vi "Engineer Ambitiously One LIne.vi"() -> ()   [LabVIEW 2025]
uses:
  <vilib>/Analysis/2dsp.llb/Complex FFT.vi
  <vilib>/Analysis/1siggen.llb/Ramp Pattern by Samples.vi
  <vilib>/Analysis/2dsp.llb/Resample (constant to constant, complex single-channel).vi
  <vilib>/Analysis/NI_AALPro.lvlib
  <vilib>/Analysis/NI_AALBase.lvlib
panel:
  out "Centerpoint Offset":cdb=-0.010717500369908635-0.08034946253234411i
  in  "Individual Plots Per Vector":bool
  in  "milliseconds to wait":u32=5
  out "XY Graph":cluster{"XY Graph - Light":cdb[]}[](graph)
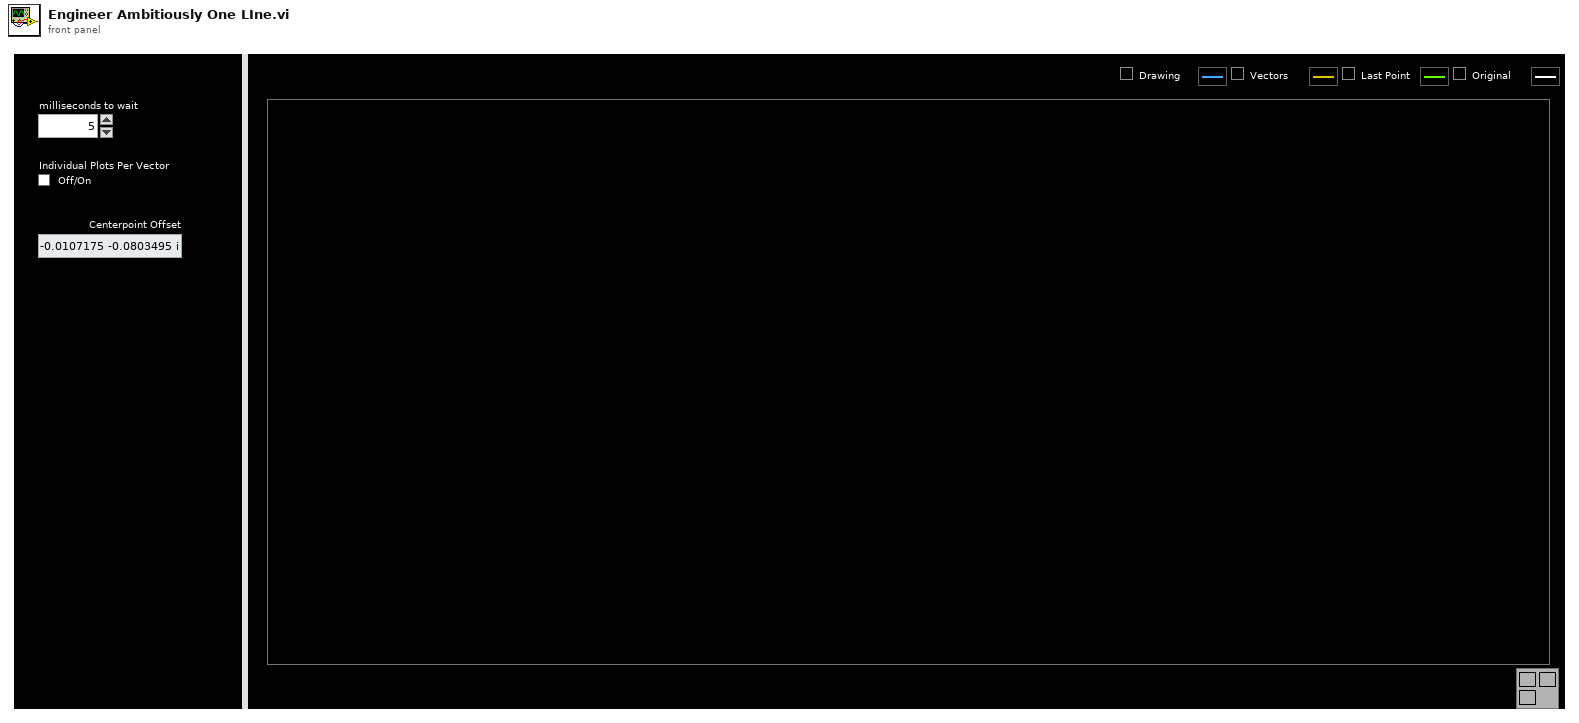
[diagram p1: front panel]
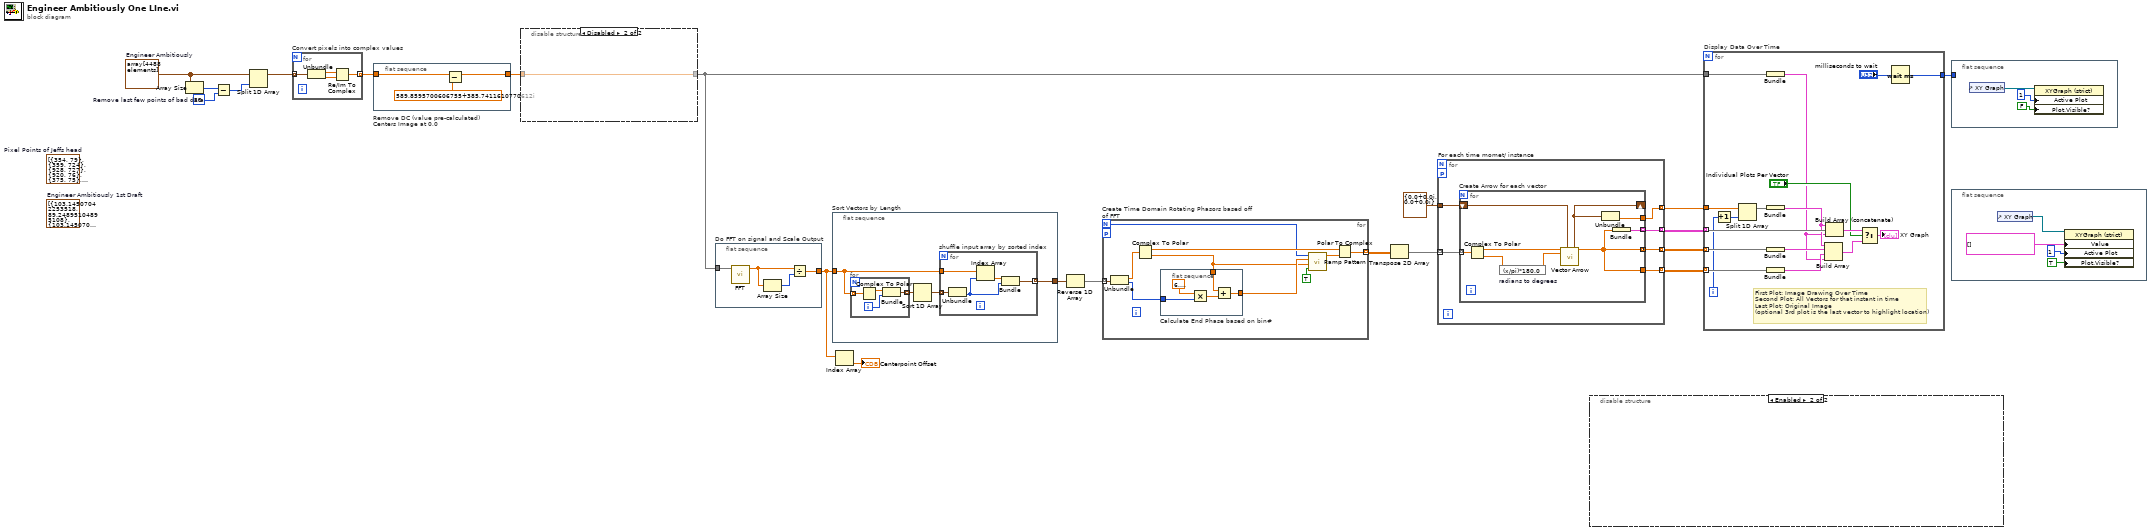
[diagram p0: block diagram]
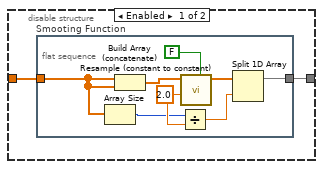
[diagram p2: hidden frame]
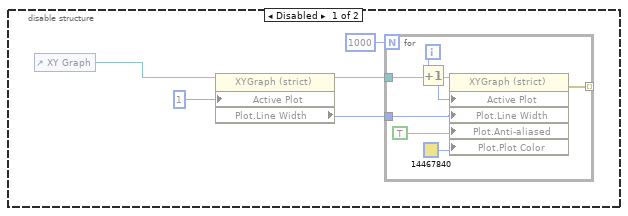
[diagram p3: hidden frame]
diagram:
  w9 = 20  # Remove last few points of bad data
  (unwired) cluster{"X":dbl, "Y":dbl}[] [{"X"=103.14507042253518, "Y"=89.24895104895108}, {"X"=103.14507042253518, "Y"=93.26013986013993}, {"X"=103.14507042253518, "Y"=95.2657342657343}, {"X"=102.14366197183094, "Y"=96.26853146853148}, {"X"=102.14366197183094, "Y"=97.27132867132866}, {"X"=102.14366197183094, "Y"=98.27412587412596}, {"X"=102.14366197183094, "Y"=99.27692307692314}, {"X"=102.14366197183094, "Y"=100.27972027972032}, {"X"=102.14366197183094, "Y"=101.2825174825175}, {"X"=102.14366197183094, "Y"=102.28531468531469}, {"X"=102.14366197183094, "Y"=103.28811188811187}, {"X"=102.14366197183094, "Y"=104.29090909090917}, {"X"=102.14366197183094, "Y"=105.29370629370635}, {"X"=102.14366197183094, "Y"=106.29650349650353}, {"X"=102.14366197183094, "Y"=107.29930069930072}, {"X"=101.14225352112672, "Y"=108.3020979020979}, {"X"=101.14225352112672, "Y"=109.30489510489508}, {"X"=101.14225352112672, "Y"=110.30769230769238}, {"X"=101.14225352112672, "Y"=111.31048951048956}, {"X"=101.14225352112672, "Y"=112.31328671328674}, {"X"=101.14225352112672, "Y"=113.31608391608393}, {"X"=101.14225352112672, "Y"=114.31888111888111}, {"X"=101.14225352112672, "Y"=115.3216783216784}, {"X"=101.14225352112672, "Y"=116.32447552447559}, {"X"=100.1408450704225, "Y"=118.33006993006995}, {"X"=100.1408450704225, "Y"=121.33846153846162}, {"X"=100.1408450704225, "Y"=123.34405594405598}, {"X"=100.1408450704225, "Y"=124.34685314685316}, {"X"=99.13943661971828, "Y"=125.34965034965035}, {"X"=98.13802816901406, "Y"=127.35524475524483}, {"X"=97.13661971830982, "Y"=130.36363636363637}, {"X"=96.1352112676056, "Y"=133.37202797202804}, {"X"=95.13380281690138, "Y"=135.3776223776224}, {"X"=94.13239436619716, "Y"=138.38601398601406}, {"X"=93.13098591549291, "Y"=139.38881118881125}, {"X"=92.1295774647887, "Y"=141.3944055944056}, {"X"=91.12816901408448, "Y"=143.39999999999998}, {"X"=90.12676056338026, "Y"=146.40839160839164}, {"X"=89.12535211267601, "Y"=148.413986013986}, {"X"=88.1239436619718, "Y"=150.41958041958048}, {"X"=86.12112676056336, "Y"=154.43076923076922}, {"X"=85.11971830985914, "Y"=157.43916083916088}, {"X"=84.11830985915489, "Y"=160.44755244755243}, {"X"=82.11549295774645, "Y"=164.45874125874127}, {"X"=81.11408450704224, "Y"=167.46713286713293}, {"X"=79.11126760563377, "Y"=172.48111888111896}, {"X"=78.10985915492955, "Y"=175.4895104895105}, {"X"=77.10845070422533, "Y"=178.49790209790217}, {"X"=76.10704225352109, "Y"=180.50349650349654}, {"X"=75.10563380281687, "Y"=182.5090909090909}, {"X"=73.10281690140843, "Y"=186.52027972027975}, {"X"=72.10140845070418, "Y"=188.5258741258741}, {"X"=71.09999999999997, "Y"=190.5314685314686}, {"X"=69.09718309859153, "Y"=193.53986013986014}, {"X"=66.09295774647885, "Y"=196.5482517482518}, {"X"=64.09014084507041, "Y"=199.55664335664335}, {"X"=62.08732394366194, "Y"=200.55944055944053}, {"X"=60.084507042253506, "Y"=203.5678321678322}, {"X"=59.08309859154926, "Y"=205.57342657342662}, {"X"=57.08028169014082, "Y"=208.58181818181822}, {"X"=56.078873239436604, "Y"=209.5846153846154}, {"X"=56.078873239436604, "Y"=211.59020979020983}, {"X"=55.07746478873236, "Y"=212.593006993007}, {"X"=55.07746478873236, "Y"=213.59580419580425}, {"X"=54.07605633802814, "Y"=213.59580419580425}, {"X"=54.07605633802814, "Y"=214.59860139860143}, {"X"=53.07464788732392, "Y"=215.6013986013986}, {"X"=53.07464788732392, "Y"=216.60419580419585}, {"X"=52.0732394366197, "Y"=216.60419580419585}, {"X"=52.0732394366197, "Y"=217.60699300699304}, {"X"=52.0732394366197, "Y"=216.60419580419585}, {"X"=54.07605633802814, "Y"=214.59860139860143}, {"X"=56.078873239436604, "Y"=211.59020979020983}, {"X"=59.08309859154926, "Y"=208.58181818181822}, {"X"=63.08873239436616, "Y"=203.5678321678322}, {"X"=65.09154929577463, "Y"=202.565034965035}, {"X"=68.09577464788731, "Y"=199.55664335664335}, {"X"=71.09999999999997, "Y"=198.55384615384617}, {"X"=73.10281690140843, "Y"=196.5482517482518}, {"X"=76.10704225352109, "Y"=194.54265734265732}, {"X"=77.10845070422533, "Y"=193.53986013986014}, {"X"=79.11126760563377, "Y"=192.53706293706296}, {"X"=82.11549295774645, "Y"=191.53426573426577}, {"X"=84.11830985915489, "Y"=190.5314685314686}, {"X"=86.12112676056336, "Y"=189.5286713286714}, {"X"=87.12253521126758, "Y"=189.5286713286714}, {"X"=89.12535211267601, "Y"=188.5258741258741}, {"X"=90.12676056338026, "Y"=188.5258741258741}, {"X"=92.1295774647887, "Y"=188.5258741258741}, {"X"=95.13380281690138, "Y"=190.5314685314686}, {"X"=98.13802816901406, "Y"=191.53426573426577}, {"X"=101.14225352112672, "Y"=192.53706293706296}, {"X"=104.1464788732394, "Y"=193.53986013986014}, {"X"=107.15070422535209, "Y"=194.54265734265732}, {"X"=110.15492957746474, "Y"=195.54545454545462}, {"X"=112.15774647887321, "Y"=195.54545454545462}, {"X"=114.16056338028164, "Y"=195.54545454545462}, {"X"=115.16197183098589, "Y"=196.5482517482518}, {"X"=116.16338028169011, "Y"=196.5482517482518}, {"X"=117.16478873239433, "Y"=196.5482517482518}, {"X"=118.16619718309855, "Y"=196.5482517482518}, {"X"=119.16760563380276, "Y"=196.5482517482518}, {"X"=118.16619718309855, "Y"=195.54545454545462}, {"X"=140.1971830985915, "Y"=210.5874125874126}, {"X"=141.19859154929574, "Y"=210.5874125874126}, {"X"=145.20422535211264, "Y"=209.5846153846154}, {"X"=145.20422535211264, "Y"=208.58181818181822}, {"X"=146.20563380281686, "Y"=208.58181818181822}, {"X"=148.2084507042253, "Y"=207.57902097902098}, {"X"=151.21267605633798, "Y"=207.57902097902098}, {"X"=154.21690140845067, "Y"=206.5762237762238}, {"X"=158.22253521126757, "Y"=205.57342657342662}, {"X"=161.22676056338022, "Y"=204.57062937062938}, {"X"=164.2309859154929, "Y"=204.57062937062938}, {"X"=167.2352112676056, "Y"=203.5678321678322}, {"X"=170.23943661971825, "Y"=203.5678321678322}, {"X"=174.24507042253515, "Y"=202.565034965035}, {"X"=176.24788732394362, "Y"=201.56223776223783}, {"X"=178.25070422535205, "Y"=200.55944055944053}, {"X"=179.2521126760563, "Y"=200.55944055944053}, {"X"=180.25352112676052, "Y"=200.55944055944053}, {"X"=183.25774647887317, "Y"=199.55664335664335}, {"X"=184.2591549295774, "Y"=199.55664335664335}, {"X"=185.2605633802816, "Y"=199.55664335664335}, {"X"=185.2605633802816, "Y"=198.55384615384617}, {"X"=186.26197183098589, "Y"=198.55384615384617}, {"X"=185.2605633802816, "Y"=198.55384615384617}, {"X"=184.2591549295774, "Y"=198.55384615384617}, {"X"=180.25352112676052, "Y"=199.55664335664335}, {"X"=177.24929577464783, "Y"=200.55944055944053}, {"X"=173.24366197183093, "Y"=201.56223776223783}, {"X"=171.2408450704225, "Y"=202.565034965035}, {"X"=168.2366197183098, "Y"=203.5678321678322}, {"X"=166.23380281690135, "Y"=203.5678321678322}, {"X"=163.2295774647887, "Y"=204.57062937062938}, {"X"=161.22676056338022, "Y"=204.57062937062938}, {"X"=158.22253521126757, "Y"=205.57342657342662}, {"X"=156.2197183098591, "Y"=205.57342657342662}, {"X"=155.21830985915489, "Y"=206.5762237762238}, {"X"=153.21549295774642, "Y"=206.5762237762238}, {"X"=152.2140845070422, "Y"=207.57902097902098}, {"X"=150.21126760563376, "Y"=207.57902097902098}, {"X"=148.2084507042253, "Y"=207.57902097902098}, {"X"=147.20704225352108, "Y"=207.57902097902098}, {"X"=145.20422535211264, "Y"=208.58181818181822}, {"X"=144.2028169014084, "Y"=208.58181818181822}, {"X"=143.20140845070418, "Y"=208.58181818181822}, {"X"=143.20140845070418, "Y"=209.5846153846154}, {"X"=142.19999999999996, "Y"=209.5846153846154}, {"X"=141.19859154929574, "Y"=209.5846153846154}, {"X"=140.1971830985915, "Y"=208.58181818181822}, {"X"=140.1971830985915, "Y"=207.57902097902098}, {"X"=140.1971830985915, "Y"=206.5762237762238}, {"X"=139.19577464788728, "Y"=206.5762237762238}, {"X"=139.19577464788728, "Y"=205.57342657342662}, {"X"=139.19577464788728, "Y"=204.57062937062938}, {"X"=138.19436619718306, "Y"=204.57062937062938}, {"X"=138.19436619718306, "Y"=203.5678321678322}, {"X"=138.19436619718306, "Y"=202.565034965035}, {"X"=138.19436619718306, "Y"=201.56223776223783}, {"X"=138.19436619718306, "Y"=200.55944055944053}, {"X"=138.19436619718306, "Y"=199.55664335664335}, {"X"=138.19436619718306, "Y"=197.55104895104898}, {"X"=139.19577464788728, "Y"=195.54545454545462}, {"X"=139.19577464788728, "Y"=193.53986013986014}, {"X"=140.1971830985915, "Y"=192.53706293706296}, {"X"=140.1971830985915, "Y"=190.5314685314686}, {"X"=141.19859154929574, "Y"=187.52307692307693}, {"X"=142.19999999999996, "Y"=186.52027972027975}, {"X"=143.20140845070418, "Y"=183.51188811188808}, {"X"=143.20140845070418, "Y"=182.5090909090909}, {"X"=144.2028169014084, "Y"=181.50629370629372}, {"X"=145.20422535211264, "Y"=178.49790209790217}, {"X"=145.20422535211264, "Y"=176.4923076923077}, {"X"=146.20563380281686, "Y"=175.4895104895105}, {"X"=147.20704225352108, "Y"=174.48671328671333}, {"X"=147.20704225352108, "Y"=173.48391608391614}, {"X"=147.20704225352108, "Y"=172.48111888111896}, {"X"=148.2084507042253, "Y"=171.47832167832166}, {"X"=148.2084507042253, "Y"=170.47552447552448}, {"X"=148.2084507042253, "Y"=169.4727272727273}, {"X"=148.2084507042253, "Y"=168.46993006993011}, {"X"=148.2084507042253, "Y"=167.46713286713293}, {"X"=149.20985915492952, "Y"=167.46713286713293}, {"X"=150.21126760563376, "Y"=167.46713286713293}, {"X"=150.21126760563376, "Y"=166.46433566433564}, {"X"=151.21267605633798, "Y"=166.46433566433564}, {"X"=153.21549295774642, "Y"=166.46433566433564}, {"X"=155.21830985915489, "Y"=165.46153846153845}, {"X"=159.2239436619718, "Y"=164.45874125874127}, {"X"=162.22816901408447, "Y"=163.4559440559441}, {"X"=165.23239436619713, "Y"=162.4531468531469}, {"X"=168.2366197183098, "Y"=161.45034965034972}, {"X"=172.2422535211267, "Y"=159.44475524475524}, {"X"=175.2464788732394, "Y"=158.44195804195806}, {"X"=178.25070422535205, "Y"=157.43916083916088}, {"X"=182.25633802816895, "Y"=156.4363636363637}, {"X"=185.2605633802816, "Y"=155.4335664335665}, {"X"=187.2633802816901, "Y"=155.4335664335665}, {"X"=190.26760563380276, "Y"=154.43076923076922}, {"X"=192.2704225352112, "Y"=154.43076923076922}, {"X"=193.27183098591541, "Y"=154.43076923076922}, {"X"=194.2732394366197, "Y"=154.43076923076922}, {"X"=195.2746478873239, "Y"=153.42797202797203}, {"X"=196.27605633802813, "Y"=153.42797202797203}, {"X"=197.27746478873235, "Y"=153.42797202797203}, {"X"=198.27887323943656, "Y"=153.42797202797203}, {"X"=199.28028169014078, "Y"=153.42797202797203}, {"X"=200.281690140845, "Y"=153.42797202797203}, {"X"=201.28309859154922, "Y"=153.42797202797203}, {"X"=199.28028169014078, "Y"=153.42797202797203}, {"X"=195.2746478873239, "Y"=154.43076923076922}, {"X"=189.26619718309854, "Y"=155.4335664335665}, {"X"=184.2591549295774, "Y"=155.4335664335665}, {"X"=178.25070422535205, "Y"=157.43916083916088}, {"X"=174.24507042253515, "Y"=158.44195804195806}, {"X"=170.23943661971825, "Y"=160.44755244755243}, {"X"=166.23380281690135, "Y"=161.45034965034972}, {"X"=161.22676056338022, "Y"=164.45874125874127}, {"X"=158.22253521126757, "Y"=165.46153846153845}, {"X"=156.2197183098591, "Y"=166.46433566433564}, {"X"=155.21830985915489, "Y"=166.46433566433564}, {"X"=153.21549295774642, "Y"=167.46713286713293}, {"X"=152.2140845070422, "Y"=167.46713286713293}, {"X"=151.21267605633798, "Y"=167.46713286713293}, {"X"=150.21126760563376, "Y"=167.46713286713293}, {"X"=150.21126760563376, "Y"=168.46993006993011}, {"X"=149.20985915492952, "Y"=168.46993006993011}, {"X"=149.20985915492952, "Y"=170.47552447552448}, {"X"=147.20704225352108, "Y"=173.48391608391614}, {"X"=145.20422535211264, "Y"=177.49510489510487}, {"X"=144.2028169014084, "Y"=179.50069930069935}, {"X"=142.19999999999996, "Y"=182.5090909090909}, {"X"=141.19859154929574, "Y"=184.51468531468538}, {"X"=141.19859154929574, "Y"=185.51748251748256}, {"X"=140.1971830985915, "Y"=185.51748251748256}, {"X"=140.1971830985915, "Y"=186.52027972027975}, {"X"=139.19577464788728, "Y"=188.5258741258741}, {"X"=138.19436619718306, "Y"=188.5258741258741}, {"X"=138.19436619718306, "Y"=189.5286713286714}, {"X"=137.19295774647884, "Y"=189.5286713286714}, {"X"=137.19295774647884, "Y"=190.5314685314686}, {"X"=136.1915492957746, "Y"=190.5314685314686}, {"X"=137.19295774647884, "Y"=191.53426573426577}, {"X"=140.1971830985915, "Y"=190.5314685314686}, {"X"=143.20140845070418, "Y"=190.5314685314686}, {"X"=145.20422535211264, "Y"=190.5314685314686}, {"X"=147.20704225352108, "Y"=189.5286713286714}, {"X"=152.2140845070422, "Y"=189.5286713286714}, {"X"=155.21830985915489, "Y"=188.5258741258741}, {"X"=162.22816901408447, "Y"=186.52027972027975}, {"X"=167.2352112676056, "Y"=185.51748251748256}, {"X"=171.2408450704225, "Y"=184.51468531468538}, {"X"=176.24788732394362, "Y"=183.51188811188808}, {"X"=179.2521126760563, "Y"=182.5090909090909}, {"X"=183.25774647887317, "Y"=180.50349650349654}, {"X"=185.2605633802816, "Y"=180.50349650349654}, {"X"=187.2633802816901, "Y"=180.50349650349654}, {"X"=189.26619718309854, "Y"=179.50069930069935}, {"X"=191.26901408450698, "Y"=179.50069930069935}, {"X"=193.27183098591541, "Y"=179.50069930069935}, {"X"=193.27183098591541, "Y"=178.49790209790217}, {"X"=194.2732394366197, "Y"=178.49790209790217}, {"X"=195.2746478873239, "Y"=178.49790209790217}, {"X"=196.27605633802813, "Y"=178.49790209790217}, {"X"=197.27746478873235, "Y"=178.49790209790217}, {"X"=196.27605633802813, "Y"=178.49790209790217}, {"X"=197.27746478873235, "Y"=178.49790209790217}, {"X"=196.27605633802813, "Y"=178.49790209790217}, {"X"=197.27746478873235, "Y"=178.49790209790217}, {"X"=198.27887323943656, "Y"=178.49790209790217}, {"X"=197.27746478873235, "Y"=178.49790209790217}, {"X"=196.27605633802813, "Y"=178.49790209790217}, {"X"=195.2746478873239, "Y"=178.49790209790217}, {"X"=192.2704225352112, "Y"=179.50069930069935}, {"X"=190.26760563380276, "Y"=180.50349650349654}, {"X"=189.26619718309854, "Y"=180.50349650349654}, {"X"=187.2633802816901, "Y"=180.50349650349654}, {"X"=186.26197183098589, "Y"=181.50629370629372}, {"X"=185.2605633802816, "Y"=181.50629370629372}, {"X"=184.2591549295774, "Y"=181.50629370629372}, {"X"=184.2591549295774, "Y"=182.5090909090909}, {"X"=183.25774647887317, "Y"=182.5090909090909}, {"X"=180.25352112676052, "Y"=183.51188811188808}, {"X"=176.24788732394362, "Y"=184.51468531468538}, {"X"=170.23943661971825, "Y"=185.51748251748256}, {"X"=165.23239436619713, "Y"=186.52027972027975}, {"X"=161.22676056338022, "Y"=187.52307692307693}, {"X"=158.22253521126757, "Y"=187.52307692307693}, {"X"=157.22112676056332, "Y"=187.52307692307693}, {"X"=156.2197183098591, "Y"=188.5258741258741}, {"X"=154.21690140845067, "Y"=188.5258741258741}, {"X"=152.2140845070422, "Y"=188.5258741258741}, {"X"=151.21267605633798, "Y"=189.5286713286714}, {"X"=147.20704225352108, "Y"=189.5286713286714}, {"X"=145.20422535211264, "Y"=189.5286713286714}, {"X"=142.19999999999996, "Y"=190.5314685314686}, {"X"=141.19859154929574, "Y"=190.5314685314686}, {"X"=140.1971830985915, "Y"=190.5314685314686}, {"X"=139.19577464788728, "Y"=190.5314685314686}, {"X"=138.19436619718306, "Y"=190.5314685314686}, {"X"=137.19295774647884, "Y"=190.5314685314686}, {"X"=136.1915492957746, "Y"=190.5314685314686}, {"X"=137.19295774647884, "Y"=190.5314685314686}, {"X"=138.19436619718306, "Y"=189.5286713286714}, {"X"=149.20985915492952, "Y"=168.46993006993011}, {"X"=200.281690140845, "Y"=153.42797202797203}, {"X"=213.29999999999995, "Y"=168.46993006993011}, {"X"=216.3042253521126, "Y"=167.46713286713293}, {"X"=218.30704225352105, "Y"=167.46713286713293}, {"X"=221.31126760563376, "Y"=166.46433566433564}, {"X"=226.31830985915485, "Y"=166.46433566433564}, {"X"=231.325352112676, "Y"=165.46153846153845}, {"X"=236.3323943661971, "Y"=164.45874125874127}, {"X"=243.34225352112668, "Y"=163.4559440559441}, {"X"=247.3478873239436, "Y"=163.4559440559441}, {"X"=251.35352112676048, "Y"=163.4559440559441}, {"X"=254.3577464788732, "Y"=163.4559440559441}, {"X"=256.36056338028163, "Y"=163.4559440559441}, {"X"=258.36338028169007, "Y"=162.4531468531469}, {"X"=259.3647887323943, "Y"=162.4531468531469}, {"X"=261.3676056338027, "Y"=162.4531468531469}, {"X"=262.36901408450694, "Y"=162.4531468531469}, {"X"=263.3704225352112, "Y"=162.4531468531469}, {"X"=264.37183098591544, "Y"=162.4531468531469}, {"X"=264.37183098591544, "Y"=161.45034965034972}, {"X"=265.37323943661966, "Y"=161.45034965034972}, {"X"=266.3746478873239, "Y"=161.45034965034972}, {"X"=267.3760563380281, "Y"=161.45034965034972}, {"X"=268.3774647887323, "Y"=161.45034965034972}, {"X"=268.3774647887323, "Y"=160.44755244755243}, {"X"=269.37887323943653, "Y"=160.44755244755243}, {"X"=269.37887323943653, "Y"=161.45034965034972}, {"X"=268.3774647887323, "Y"=161.45034965034972}, {"X"=267.3760563380281, "Y"=161.45034965034972}, {"X"=265.37323943661966, "Y"=161.45034965034972}, {"X"=262.36901408450694, "Y"=162.4531468531469}, {"X"=255.35915492957741, "Y"=164.45874125874127}, {"X"=249.35070422535205, "Y"=164.45874125874127}, {"X"=243.34225352112668, "Y"=165.46153846153845}, {"X"=240.33802816901402, "Y"=165.46153846153845}, {"X"=236.3323943661971, "Y"=165.46153846153845}, {"X"=234.32957746478866, "Y"=165.46153846153845}, {"X"=232.32676056338022, "Y"=165.46153846153845}, {"X"=231.325352112676, "Y"=166.46433566433564}, {"X"=230.32394366197178, "Y"=166.46433566433564}, {"X"=229.32253521126756, "Y"=166.46433566433564}, {"X"=228.32112676056335, "Y"=166.46433566433564}, {"X"=227.31971830985907, "Y"=166.46433566433564}, {"X"=226.31830985915485, "Y"=165.46153846153845}, {"X"=226.31830985915485, "Y"=166.46433566433564}, {"X"=225.31690140845063, "Y"=167.46713286713293}, {"X"=225.31690140845063, "Y"=168.46993006993011}, {"X"=224.31549295774641, "Y"=171.47832167832166}, {"X"=223.3140845070422, "Y"=174.48671328671333}, {"X"=221.31126760563376, "Y"=177.49510489510487}, {"X"=219.30845070422527, "Y"=180.50349650349654}, {"X"=216.3042253521126, "Y"=185.51748251748256}, {"X"=214.30140845070417, "Y"=189.5286713286714}, {"X"=212.29859154929574, "Y"=191.53426573426577}, {"X"=211.29718309859152, "Y"=193.53986013986014}, {"X"=210.29577464788724, "Y"=195.54545454545462}, {"X"=209.29436619718302, "Y"=195.54545454545462}, {"X"=209.29436619718302, "Y"=196.5482517482518}, {"X"=209.29436619718302, "Y"=197.55104895104898}, {"X"=208.2929577464788, "Y"=197.55104895104898}, {"X"=208.2929577464788, "Y"=198.55384615384617}, {"X"=207.2915492957746, "Y"=199.55664335664335}, {"X"=207.2915492957746, "Y"=200.55944055944053}, {"X"=207.2915492957746, "Y"=199.55664335664335}, {"X"=225.31690140845063, "Y"=166.46433566433564}, {"X"=261.3676056338027, "Y"=161.45034965034972}, {"X"=307.4323943661971, "Y"=155.4335664335665}, {"X"=305.4295774647887, "Y"=151.42237762237767}, {"X"=305.4295774647887, "Y"=150.41958041958048}, {"X"=304.4281690140844, "Y"=150.41958041958048}, {"X"=303.4267605633802, "Y"=150.41958041958048}, {"X"=302.42535211267597, "Y"=150.41958041958048}, {"X"=301.42394366197175, "Y"=150.41958041958048}, {"X"=300.42253521126753, "Y"=150.41958041958048}, {"X"=299.4211267605633, "Y"=150.41958041958048}, {"X"=298.4197183098591, "Y"=150.41958041958048}, {"X"=297.4183098591549, "Y"=150.41958041958048}, {"X"=296.4169014084506, "Y"=150.41958041958048}, {"X"=294.41408450704216, "Y"=151.42237762237767}, {"X"=292.4112676056337, "Y"=151.42237762237767}, {"X"=291.4098591549295, "Y"=151.42237762237767}, {"X"=290.4084507042253, "Y"=151.42237762237767}, {"X"=289.40704225352107, "Y"=151.42237762237767}, {"X"=289.40704225352107, "Y"=152.42517482517485}, {"X"=288.40563380281685, "Y"=152.42517482517485}, {"X"=287.4042253521126, "Y"=152.42517482517485}, {"X"=286.40281690140836, "Y"=153.42797202797203}, {"X"=285.40140845070414, "Y"=154.43076923076922}, {"X"=284.3999999999999, "Y"=154.43076923076922}, {"X"=283.3985915492957, "Y"=155.4335664335665}, {"X"=282.3971830985915, "Y"=156.4363636363637}, {"X"=281.39577464788727, "Y"=156.4363636363637}, {"X"=281.39577464788727, "Y"=157.43916083916088}, {"X"=280.39436619718305, "Y"=158.44195804195806}, {"X"=280.39436619718305, "Y"=159.44475524475524}, {"X"=279.39295774647877, "Y"=161.45034965034972}, {"X"=279.39295774647877, "Y"=162.4531468531469}, {"X"=280.39436619718305, "Y"=163.4559440559441}, {"X"=280.39436619718305, "Y"=164.45874125874127}, {"X"=280.39436619718305, "Y"=166.46433566433564}, {"X"=281.39577464788727, "Y"=167.46713286713293}, {"X"=282.3971830985915, "Y"=168.46993006993011}, {"X"=283.3985915492957, "Y"=169.4727272727273}, {"X"=283.3985915492957, "Y"=170.47552447552448}, {"X"=284.3999999999999, "Y"=170.47552447552448}, {"X"=284.3999999999999, "Y"=171.47832167832166}, {"X"=286.40281690140836, "Y"=173.48391608391614}, {"X"=287.4042253521126, "Y"=174.48671328671333}, {"X"=288.40563380281685, "Y"=174.48671328671333}, {"X"=288.40563380281685, "Y"=175.4895104895105}, {"X"=289.40704225352107, "Y"=176.4923076923077}, {"X"=291.4098591549295, "Y"=178.49790209790217}, {"X"=292.4112676056337, "Y"=179.50069930069935}, {"X"=293.41267605633794, "Y"=180.50349650349654}, {"X"=294.41408450704216, "Y"=181.50629370629372}, {"X"=294.41408450704216, "Y"=182.5090909090909}, {"X"=295.4154929577464, "Y"=184.51468531468538}, {"X"=296.4169014084506, "Y"=184.51468531468538}, {"X"=296.4169014084506, "Y"=186.52027972027975}, {"X"=297.4183098591549, "Y"=186.52027972027975}, {"X"=297.4183098591549, "Y"=187.52307692307693}, {"X"=298.4197183098591, "Y"=187.52307692307693}, {"X"=298.4197183098591, "Y"=188.5258741258741}, {"X"=298.4197183098591, "Y"=189.5286713286714}, {"X"=298.4197183098591, "Y"=190.5314685314686}, {"X"=298.4197183098591, "Y"=191.53426573426577}, {"X"=298.4197183098591, "Y"=192.53706293706296}, {"X"=298.4197183098591, "Y"=193.53986013986014}, {"X"=298.4197183098591, "Y"=194.54265734265732}, {"X"=297.4183098591549, "Y"=194.54265734265732}, {"X"=297.4183098591549, "Y"=195.54545454545462}, {"X"=297.4183098591549, "Y"=196.5482517482518}, {"X"=296.4169014084506, "Y"=196.5482517482518}, {"X"=295.4154929577464, "Y"=196.5482517482518}, {"X"=295.4154929577464, "Y"=197.55104895104898}, {"X"=294.41408450704216, "Y"=197.55104895104898}, {"X"=293.41267605633794, "Y"=197.55104895104898}, {"X"=293.41267605633794, "Y"=198.55384615384617}, {"X"=292.4112676056337, "Y"=198.55384615384617}, {"X"=290.4084507042253, "Y"=198.55384615384617}, {"X"=289.40704225352107, "Y"=198.55384615384617}, {"X"=288.40563380281685, "Y"=198.55384615384617}, {"X"=286.40281690140836, "Y"=199.55664335664335}, {"X"=285.40140845070414, "Y"=199.55664335664335}, {"X"=283.3985915492957, "Y"=199.55664335664335}, {"X"=282.3971830985915, "Y"=199.55664335664335}, {"X"=280.39436619718305, "Y"=199.55664335664335}, {"X"=279.39295774647877, "Y"=199.55664335664335}, {"X"=276.3887323943661, "Y"=199.55664335664335}, {"X"=274.3859154929577, "Y"=199.55664335664335}, {"X"=273.38450704225346, "Y"=200.55944055944053}, {"X"=272.38309859154924, "Y"=200.55944055944053}, {"X"=269.37887323943653, "Y"=200.55944055944053}, {"X"=267.3760563380281, "Y"=200.55944055944053}, {"X"=265.37323943661966, "Y"=200.55944055944053}, {"X"=263.3704225352112, "Y"=200.55944055944053}, {"X"=261.3676056338027, "Y"=200.55944055944053}, {"X"=259.3647887323943, "Y"=199.55664335664335}, {"X"=257.36197183098585, "Y"=199.55664335664335}, {"X"=255.35915492957741, "Y"=199.55664335664335}, {"X"=254.3577464788732, "Y"=199.55664335664335}, {"X"=254.3577464788732, "Y"=198.55384615384617}, {"X"=253.35633802816892, "Y"=198.55384615384617}, {"X"=252.3549295774647, "Y"=198.55384615384617}, {"X"=251.35352112676048, "Y"=198.55384615384617}, {"X"=250.35211267605627, "Y"=198.55384615384617}, {"X"=299.4211267605633, "Y"=190.5314685314686}, {"X"=300.42253521126753, "Y"=180.50349650349654}, {"X"=285.40140845070414, "Y"=169.4727272727273}, {"X"=281.39577464788727, "Y"=155.4335664335665}, {"X"=294.41408450704216, "Y"=148.413986013986}, {"X"=310.43661971830977, "Y"=146.40839160839164}, {"X"=375.5281690140844, "Y"=141.3944055944056}, {"X"=378.5323943661971, "Y"=141.3944055944056}, {"X"=379.5338028169013, "Y"=141.3944055944056}, {"X"=380.5352112676055, "Y"=140.39160839160843}, {"X"=381.53661971830974, "Y"=140.39160839160843}, {"X"=381.53661971830974, "Y"=139.38881118881125}, {"X"=382.538028169014, "Y"=139.38881118881125}, {"X"=383.53943661971823, "Y"=139.38881118881125}, {"X"=384.54084507042245, "Y"=139.38881118881125}, {"X"=384.54084507042245, "Y"=138.38601398601406}, {"X"=385.54225352112667, "Y"=138.38601398601406}, {"X"=387.5450704225351, "Y"=138.38601398601406}, {"X"=389.54788732394354, "Y"=138.38601398601406}, {"X"=390.54929577464776, "Y"=137.38321678321677}, {"X"=391.55070422535204, "Y"=137.38321678321677}, {"X"=392.55211267605625, "Y"=137.38321678321677}, {"X"=394.5549295774647, "Y"=136.38041958041958}, {"X"=395.5563380281689, "Y"=136.38041958041958}, {"X"=397.55915492957735, "Y"=135.3776223776224}, {"X"=399.56197183098584, "Y"=134.37482517482522}, {"X"=402.5661971830985, "Y"=134.37482517482522}, {"X"=404.56901408450693, "Y"=133.37202797202804}, {"X"=406.57183098591537, "Y"=133.37202797202804}, {"X"=408.57464788732386, "Y"=132.36923076923085}, {"X"=410.5774647887323, "Y"=132.36923076923085}, {"X"=412.58028169014074, "Y"=132.36923076923085}, {"X"=414.5830985915492, "Y"=132.36923076923085}, {"X"=416.58591549295767, "Y"=131.36643356643356}, {"X"=417.5873239436619, "Y"=131.36643356643356}, {"X"=419.5901408450703, "Y"=131.36643356643356}, {"X"=421.59295774647876, "Y"=131.36643356643356}, {"X"=422.594366197183, "Y"=130.36363636363637}, {"X"=424.5971830985914, "Y"=130.36363636363637}, {"X"=427.6014084507041, "Y"=129.3608391608392}, {"X"=430.6056338028168, "Y"=129.3608391608392}, {"X"=432.6084507042252, "Y"=129.3608391608392}, {"X"=435.61267605633793, "Y"=129.3608391608392}, {"X"=438.61690140845064, "Y"=128.358041958042}, {"X"=441.62112676056324, "Y"=128.358041958042}, {"X"=443.6239436619717, "Y"=128.358041958042}, {"X"=446.6281690140844, "Y"=128.358041958042}, {"X"=447.62957746478867, "Y"=128.358041958042}, {"X"=450.63380281690127, "Y"=128.358041958042}, {"X"=452.6366197183097, "Y"=128.358041958042}, {"X"=453.638028169014, "Y"=128.358041958042}, {"X"=455.6408450704224, "Y"=128.358041958042}, {"X"=457.64366197183085, "Y"=128.358041958042}, {"X"=458.6450704225351, "Y"=128.358041958042}, {"X"=460.64788732394356, "Y"=128.358041958042}, {"X"=461.6492957746477, "Y"=128.358041958042}, {"X"=462.650704225352, "Y"=128.358041958042}, {"X"=463.6521126760563, "Y"=128.358041958042}, {"X"=464.65352112676044, "Y"=128.358041958042}, {"X"=465.6549295774647, "Y"=128.358041958042}, {"X"=466.6563380281689, "Y"=128.358041958042}, {"X"=467.65774647887315, "Y"=128.358041958042}, {"X"=468.6591549295773, "Y"=128.358041958042}, {"X"=469.6605633802816, "Y"=128.358041958042}, {"X"=470.66197183098575, "Y"=128.358041958042}, {"X"=471.66338028169, "Y"=128.358041958042}, {"X"=472.6647887323943, "Y"=128.358041958042}, {"X"=471.66338028169, "Y"=128.358041958042}, {"X"=472.6647887323943, "Y"=128.358041958042}, {"X"=471.66338028169, "Y"=128.358041958042}, {"X"=470.66197183098575, "Y"=128.358041958042}, {"X"=469.6605633802816, "Y"=128.358041958042}, {"X"=468.6591549295773, "Y"=128.358041958042}, {"X"=467.65774647887315, "Y"=128.358041958042}, {"X"=466.6563380281689, "Y"=128.358041958042}, {"X"=465.6549295774647, "Y"=128.358041958042}, {"X"=463.6521126760563, "Y"=129.3608391608392}, {"X"=460.64788732394356, "Y"=129.3608391608392}, {"X"=457.64366197183085, "Y"=129.3608391608392}, {"X"=454.63943661971814, "Y"=130.36363636363637}, {"X"=451.63521126760554, "Y"=130.36363636363637}, {"X"=448.63098591549283, "Y"=130.36363636363637}, {"X"=446.6281690140844, "Y"=131.36643356643356}, {"X"=443.6239436619717, "Y"=131.36643356643356}, {"X"=440.6197183098591, "Y"=131.36643356643356}, {"X"=437.61549295774637, "Y"=131.36643356643356}, {"X"=435.61267605633793, "Y"=131.36643356643356}, {"X"=433.6098591549295, "Y"=131.36643356643356}, {"X"=431.607042253521, "Y"=131.36643356643356}, {"X"=428.60281690140835, "Y"=131.36643356643356}, {"X"=425.5985915492957, "Y"=131.36643356643356}, {"X"=423.5957746478872, "Y"=131.36643356643356}, {"X"=421.59295774647876, "Y"=131.36643356643356}, {"X"=419.5901408450703, "Y"=131.36643356643356}, {"X"=418.5887323943661, "Y"=131.36643356643356}, {"X"=416.58591549295767, "Y"=131.36643356643356}, {"X"=415.5845070422534, "Y"=131.36643356643356}, {"X"=414.5830985915492, "Y"=131.36643356643356}, {"X"=413.58169014084496, "Y"=131.36643356643356}, {"X"=412.58028169014074, "Y"=131.36643356643356}, {"X"=411.5788732394365, "Y"=131.36643356643356}, {"X"=410.5774647887323, "Y"=131.36643356643356}, {"X"=409.5760563380281, "Y"=131.36643356643356}, {"X"=408.57464788732386, "Y"=131.36643356643356}, {"X"=407.5732394366196, "Y"=131.36643356643356}, {"X"=406.57183098591537, "Y"=131.36643356643356}, {"X"=406.57183098591537, "Y"=132.36923076923085}, {"X"=405.57042253521115, "Y"=132.36923076923085}, {"X"=405.57042253521115, "Y"=133.37202797202804}, {"X"=404.56901408450693, "Y"=133.37202797202804}, {"X"=403.5676056338027, "Y"=134.37482517482522}, {"X"=402.5661971830985, "Y"=134.37482517482522}, {"X"=401.5647887323943, "Y"=137.38321678321677}, {"X"=400.56338028169006, "Y"=137.38321678321677}, {"X"=399.56197183098584, "Y"=138.38601398601406}, {"X"=398.56056338028156, "Y"=140.39160839160843}, {"X"=396.5577464788731, "Y"=143.39999999999998}, {"X"=394.5549295774647, "Y"=144.40279720279727}, {"X"=393.5535211267605, "Y"=146.40839160839164}, {"X"=391.55070422535204, "Y"=147.41118881118882}, {"X"=390.54929577464776, "Y"=148.413986013986}, {"X"=388.5464788732393, "Y"=149.4167832167833}, {"X"=387.5450704225351, "Y"=150.41958041958048}, {"X"=385.54225352112667, "Y"=151.42237762237767}, {"X"=384.54084507042245, "Y"=152.42517482517485}, {"X"=383.53943661971823, "Y"=153.42797202797203}, {"X"=382.538028169014, "Y"=154.43076923076922}, {"X"=381.53661971830974, "Y"=156.4363636363637}, {"X"=380.5352112676055, "Y"=159.44475524475524}, {"X"=379.5338028169013, "Y"=160.44755244755243}, {"X"=379.5338028169013, "Y"=162.4531468531469}, {"X"=377.53098591549286, "Y"=165.46153846153845}, {"X"=377.53098591549286, "Y"=167.46713286713293}, {"X"=376.52957746478864, "Y"=168.46993006993011}, {"X"=375.5281690140844, "Y"=170.47552447552448}, {"X"=375.5281690140844, "Y"=171.47832167832166}, {"X"=375.5281690140844, "Y"=172.48111888111896}, {"X"=374.5267605633802, "Y"=172.48111888111896}, {"X"=374.5267605633802, "Y"=173.48391608391614}, {"X"=373.52535211267593, "Y"=174.48671328671333}, {"X"=373.52535211267593, "Y"=175.4895104895105}, {"X"=372.5239436619717, "Y"=175.4895104895105}, {"X"=372.5239436619717, "Y"=176.4923076923077}, {"X"=372.5239436619717, "Y"=177.49510489510487}, {"X"=371.5225352112675, "Y"=179.50069930069935}, {"X"=371.5225352112675, "Y"=180.50349650349654}, {"X"=371.5225352112675, "Y"=181.50629370629372}, {"X"=371.5225352112675, "Y"=182.5090909090909}, {"X"=371.5225352112675, "Y"=183.51188811188808}, {"X"=371.5225352112675, "Y"=184.51468531468538}, {"X"=371.5225352112675, "Y"=185.51748251748256}, {"X"=371.5225352112675, "Y"=186.52027972027975}, {"X"=370.5211267605633, "Y"=187.52307692307693}, {"X"=370.5211267605633, "Y"=188.5258741258741}, {"X"=370.5211267605633, "Y"=189.5286713286714}, {"X"=370.5211267605633, "Y"=190.5314685314686}, {"X"=370.5211267605633, "Y"=191.53426573426577}, {"X"=370.5211267605633, "Y"=192.53706293706296}, {"X"=370.5211267605633, "Y"=193.53986013986014}, {"X"=370.5211267605633, "Y"=194.54265734265732}, {"X"=371.5225352112675, "Y"=195.54545454545462}, {"X"=371.5225352112675, "Y"=196.5482517482518}, {"X"=371.5225352112675, "Y"=197.55104895104898}, {"X"=371.5225352112675, "Y"=198.55384615384617}, {"X"=372.5239436619717, "Y"=198.55384615384617}, {"X"=372.5239436619717, "Y"=199.55664335664335}, {"X"=373.52535211267593, "Y"=199.55664335664335}, {"X"=374.5267605633802, "Y"=200.55944055944053}, {"X"=375.5281690140844, "Y"=200.55944055944053}, {"X"=376.52957746478864, "Y"=200.55944055944053}, {"X"=376.52957746478864, "Y"=201.56223776223783}, {"X"=378.5323943661971, "Y"=201.56223776223783}, {"X"=379.5338028169013, "Y"=201.56223776223783}, {"X"=382.538028169014, "Y"=201.56223776223783}, {"X"=384.54084507042245, "Y"=201.56223776223783}, {"X"=386.5436619718309, "Y"=201.56223776223783}, {"X"=387.5450704225351, "Y"=201.56223776223783}, {"X"=389.54788732394354, "Y"=200.55944055944053}, {"X"=391.55070422535204, "Y"=200.55944055944053}, {"X"=393.5535211267605, "Y"=200.55944055944053}, {"X"=395.5563380281689, "Y"=199.55664335664335}, {"X"=397.55915492957735, "Y"=199.55664335664335}, {"X"=399.56197183098584, "Y"=198.55384615384617}, {"X"=402.5661971830985, "Y"=198.55384615384617}, {"X"=404.56901408450693, "Y"=197.55104895104898}, {"X"=406.57183098591537, "Y"=197.55104895104898}, {"X"=409.5760563380281, "Y"=196.5482517482518}, {"X"=410.5774647887323, "Y"=195.54545454545462}, {"X"=412.58028169014074, "Y"=195.54545454545462}, {"X"=414.5830985915492, "Y"=195.54545454545462}, {"X"=417.5873239436619, "Y"=193.53986013986014}, {"X"=419.5901408450703, "Y"=193.53986013986014}, {"X"=421.59295774647876, "Y"=192.53706293706296}, {"X"=423.5957746478872, "Y"=191.53426573426577}, {"X"=425.5985915492957, "Y"=191.53426573426577}, {"X"=427.6014084507041, "Y"=190.5314685314686}, {"X"=429.60422535211256, "Y"=190.5314685314686}, {"X"=430.6056338028168, "Y"=189.5286713286714}, {"X"=431.607042253521, "Y"=189.5286713286714}, {"X"=432.6084507042252, "Y"=188.5258741258741}, {"X"=433.6098591549295, "Y"=188.5258741258741}, {"X"=434.6112676056337, "Y"=188.5258741258741}, {"X"=435.61267605633793, "Y"=188.5258741258741}, {"X"=435.61267605633793, "Y"=187.52307692307693}, {"X"=435.61267605633793, "Y"=188.5258741258741}, {"X"=434.6112676056337, "Y"=188.5258741258741}, {"X"=434.6112676056337, "Y"=187.52307692307693}, {"X"=373.52535211267593, "Y"=198.55384615384617}, {"X"=367.5169014084506, "Y"=185.51748251748256}, {"X"=373.52535211267593, "Y"=173.48391608391614}, {"X"=373.52535211267593, "Y"=174.48671328671333}, {"X"=378.5323943661971, "Y"=173.48391608391614}, {"X"=379.5338028169013, "Y"=173.48391608391614}, {"X"=380.5352112676055, "Y"=173.48391608391614}, {"X"=381.53661971830974, "Y"=173.48391608391614}, {"X"=382.538028169014, "Y"=173.48391608391614}, {"X"=383.53943661971823, "Y"=173.48391608391614}, {"X"=383.53943661971823, "Y"=172.48111888111896}, {"X"=384.54084507042245, "Y"=172.48111888111896}, {"X"=385.54225352112667, "Y"=172.48111888111896}, {"X"=387.5450704225351, "Y"=172.48111888111896}, {"X"=388.5464788732393, "Y"=172.48111888111896}, {"X"=389.54788732394354, "Y"=172.48111888111896}, {"X"=390.54929577464776, "Y"=172.48111888111896}, {"X"=392.55211267605625, "Y"=171.47832167832166}, {"X"=393.5535211267605, "Y"=171.47832167832166}, {"X"=394.5549295774647, "Y"=171.47832167832166}, {"X"=395.5563380281689, "Y"=171.47832167832166}, {"X"=396.5577464788731, "Y"=171.47832167832166}, {"X"=398.56056338028156, "Y"=170.47552447552448}, {"X"=399.56197183098584, "Y"=170.47552447552448}, {"X"=401.5647887323943, "Y"=170.47552447552448}, {"X"=402.5661971830985, "Y"=169.4727272727273}, {"X"=403.5676056338027, "Y"=169.4727272727273}, {"X"=405.57042253521115, "Y"=169.4727272727273}, {"X"=406.57183098591537, "Y"=168.46993006993011}, {"X"=408.57464788732386, "Y"=168.46993006993011}, {"X"=410.5774647887323, "Y"=168.46993006993011}, {"X"=412.58028169014074, "Y"=167.46713286713293}, {"X"=413.58169014084496, "Y"=167.46713286713293}, {"X"=415.5845070422534, "Y"=167.46713286713293}, {"X"=418.5887323943661, "Y"=167.46713286713293}, {"X"=419.5901408450703, "Y"=167.46713286713293}, {"X"=420.59154929577454, "Y"=166.46433566433564}, {"X"=421.59295774647876, "Y"=166.46433566433564}, {"X"=423.5957746478872, "Y"=166.46433566433564}, {"X"=423.5957746478872, "Y"=165.46153846153845}, {"X"=424.5971830985914, "Y"=165.46153846153845}, {"X"=425.5985915492957, "Y"=165.46153846153845}, {"X"=427.6014084507041, "Y"=164.45874125874127}, {"X"=428.60281690140835, "Y"=164.45874125874127}, {"X"=430.6056338028168, "Y"=164.45874125874127}, {"X"=431.607042253521, "Y"=164.45874125874127}, {"X"=433.6098591549295, "Y"=164.45874125874127}, {"X"=435.61267605633793, "Y"=164.45874125874127}, {"X"=436.61408450704215, "Y"=163.4559440559441}, {"X"=437.61549295774637, "Y"=163.4559440559441}, {"X"=438.61690140845064, "Y"=163.4559440559441}, {"X"=439.6183098591548, "Y"=163.4559440559441}, {"X"=440.6197183098591, "Y"=163.4559440559441}, {"X"=441.62112676056324, "Y"=162.4531468531469}, {"X"=442.6225352112675, "Y"=162.4531468531469}, {"X"=443.6239436619717, "Y"=162.4531468531469}, {"X"=444.62535211267596, "Y"=162.4531468531469}, {"X"=444.62535211267596, "Y"=163.4559440559441}, {"X"=445.6267605633801, "Y"=163.4559440559441}, {"X"=445.6267605633801, "Y"=162.4531468531469}, {"X"=445.6267605633801, "Y"=163.4559440559441}, {"X"=444.62535211267596, "Y"=163.4559440559441}, {"X"=443.6239436619717, "Y"=163.4559440559441}, {"X"=442.6225352112675, "Y"=163.4559440559441}, {"X"=441.62112676056324, "Y"=163.4559440559441}, {"X"=440.6197183098591, "Y"=163.4559440559441}, {"X"=439.6183098591548, "Y"=163.4559440559441}, {"X"=438.61690140845064, "Y"=163.4559440559441}, {"X"=437.61549295774637, "Y"=163.4559440559441}, {"X"=434.6112676056337, "Y"=163.4559440559441}, {"X"=429.60422535211256, "Y"=164.45874125874127}, {"X"=425.5985915492957, "Y"=164.45874125874127}, {"X"=422.594366197183, "Y"=164.45874125874127}, {"X"=419.5901408450703, "Y"=165.46153846153845}, {"X"=417.5873239436619, "Y"=165.46153846153845}, {"X"=414.5830985915492, "Y"=167.46713286713293}, {"X"=411.5788732394365, "Y"=167.46713286713293}, {"X"=409.5760563380281, "Y"=168.46993006993011}, {"X"=406.57183098591537, "Y"=169.4727272727273}, {"X"=403.5676056338027, "Y"=169.4727272727273}, {"X"=402.5661971830985, "Y"=170.47552447552448}, {"X"=401.5647887323943, "Y"=170.47552447552448}, {"X"=400.56338028169006, "Y"=170.47552447552448}, {"X"=399.56197183098584, "Y"=170.47552447552448}, {"X"=396.5577464788731, "Y"=170.47552447552448}, {"X"=392.55211267605625, "Y"=171.47832167832166}, {"X"=389.54788732394354, "Y"=172.48111888111896}, {"X"=384.54084507042245, "Y"=172.48111888111896}, {"X"=382.538028169014, "Y"=172.48111888111896}, {"X"=381.53661971830974, "Y"=173.48391608391614}, {"X"=380.5352112676055, "Y"=173.48391608391614}, {"X"=379.5338028169013, "Y"=173.48391608391614}, {"X"=378.5323943661971, "Y"=173.48391608391614}, {"X"=377.53098591549286, "Y"=173.48391608391614}, {"X"=376.52957746478864, "Y"=173.48391608391614}, {"X"=375.5281690140844, "Y"=173.48391608391614}, {"X"=374.5267605633802, "Y"=173.48391608391614}, {"X"=374.5267605633802, "Y"=172.48111888111896}, {"X"=375.5281690140844, "Y"=172.48111888111896}, {"X"=406.57183098591537, "Y"=131.36643356643356}, {"X"=470.66197183098575, "Y"=128.358041958042}, {"X"=408.57464788732386, "Y"=132.36923076923085}, {"X"=368.51830985915484, "Y"=178.49790209790217}, {"X"=372.5239436619717, "Y"=197.55104895104898}, {"X"=434.6112676056337, "Y"=187.52307692307693}, {"X"=442.6225352112675, "Y"=192.53706293706296}, {"X"=446.6281690140844, "Y"=191.53426573426577}, {"X"=448.63098591549283, "Y"=190.5314685314686}, {"X"=448.63098591549283, "Y"=189.5286713286714}, {"X"=450.63380281690127, "Y"=188.5258741258741}, {"X"=453.638028169014, "Y"=186.52027972027975}, {"X"=454.63943661971814, "Y"=185.51748251748256}, {"X"=455.6408450704224, "Y"=184.51468531468538}, {"X"=456.6422535211267, "Y"=183.51188811188808}, {"X"=458.6450704225351, "Y"=181.50629370629372}, {"X"=461.6492957746477, "Y"=178.49790209790217}, {"X"=463.6521126760563, "Y"=177.49510489510487}, {"X"=464.65352112676044, "Y"=176.4923076923077}, {"X"=465.6549295774647, "Y"=175.4895104895105}, {"X"=466.6563380281689, "Y"=173.48391608391614}, {"X"=467.65774647887315, "Y"=173.48391608391614}, {"X"=468.6591549295773, "Y"=171.47832167832166}, {"X"=469.6605633802816, "Y"=170.47552447552448}, {"X"=472.6647887323943, "Y"=167.46713286713293}, {"X"=473.66619718309846, "Y"=166.46433566433564}, {"X"=475.6690140845069, "Y"=164.45874125874127}, {"X"=477.67183098591534, "Y"=161.45034965034972}, {"X"=478.6732394366196, "Y"=160.44755244755243}, {"X"=478.6732394366196, "Y"=158.44195804195806}, {"X"=480.67605633802805, "Y"=156.4363636363637}, {"X"=482.6788732394365, "Y"=154.43076923076922}, {"X"=483.68028169014076, "Y"=153.42797202797203}, {"X"=485.6830985915492, "Y"=152.42517482517485}, {"X"=486.68450704225336, "Y"=151.42237762237767}, {"X"=486.68450704225336, "Y"=150.41958041958048}, {"X"=488.6873239436618, "Y"=149.4167832167833}, {"X"=489.68873239436607, "Y"=148.413986013986}, {"X"=491.6915492957745, "Y"=146.40839160839164}, {"X"=492.6929577464788, "Y"=145.40559440559446}, {"X"=492.6929577464788, "Y"=144.40279720279727}, {"X"=493.69436619718294, "Y"=143.39999999999998}, {"X"=494.6957746478872, "Y"=142.3972027972028}, {"X"=495.6971830985914, "Y"=141.3944055944056}, {"X"=496.69859154929566, "Y"=141.3944055944056}, {"X"=496.69859154929566, "Y"=140.39160839160843}, {"X"=497.69999999999993, "Y"=139.38881118881125}, {"X"=498.7014084507041, "Y"=138.38601398601406}, {"X"=498.7014084507041, "Y"=137.38321678321677}, {"X"=499.70281690140837, "Y"=137.38321678321677}, {"X"=499.70281690140837, "Y"=136.38041958041958}, {"X"=499.70281690140837, "Y"=135.3776223776224}, {"X"=500.70422535211253, "Y"=135.3776223776224}, {"X"=500.70422535211253, "Y"=136.38041958041958}, {"X"=500.70422535211253, "Y"=137.38321678321677}, {"X"=500.70422535211253, "Y"=138.38601398601406}, {"X"=500.70422535211253, "Y"=139.38881118881125}, {"X"=499.70281690140837, "Y"=139.38881118881125}, {"X"=499.70281690140837, "Y"=140.39160839160843}, {"X"=499.70281690140837, "Y"=141.3944055944056}, {"X"=499.70281690140837, "Y"=142.3972027972028}, {"X"=498.7014084507041, "Y"=146.40839160839164}, {"X"=497.69999999999993, "Y"=147.41118881118882}, {"X"=496.69859154929566, "Y"=149.4167832167833}, {"X"=496.69859154929566, "Y"=151.42237762237767}, {"X"=495.6971830985914, "Y"=152.42517482517485}, {"X"=495.6971830985914, "Y"=154.43076923076922}, {"X"=494.6957746478872, "Y"=157.43916083916088}, {"X"=493.69436619718294, "Y"=159.44475524475524}, {"X"=493.69436619718294, "Y"=161.45034965034972}, {"X"=492.6929577464788, "Y"=164.45874125874127}, {"X"=492.6929577464788, "Y"=166.46433566433564}, {"X"=491.6915492957745, "Y"=168.46993006993011}, {"X"=491.6915492957745, "Y"=170.47552447552448}, {"X"=490.69014084507035, "Y"=172.48111888111896}, {"X"=490.69014084507035, "Y"=173.48391608391614}, {"X"=489.68873239436607, "Y"=175.4895104895105}, {"X"=489.68873239436607, "Y"=177.49510489510487}, {"X"=488.6873239436618, "Y"=179.50069930069935}, {"X"=488.6873239436618, "Y"=180.50349650349654}, {"X"=488.6873239436618, "Y"=181.50629370629372}, {"X"=488.6873239436618, "Y"=182.5090909090909}, {"X"=488.6873239436618, "Y"=183.51188811188808}, {"X"=488.6873239436618, "Y"=184.51468531468538}, {"X"=488.6873239436618, "Y"=185.51748251748256}, {"X"=488.6873239436618, "Y"=186.52027972027975}, {"X"=488.6873239436618, "Y"=187.52307692307693}, {"X"=488.6873239436618, "Y"=188.5258741258741}, {"X"=489.68873239436607, "Y"=189.5286713286714}, {"X"=490.69014084507035, "Y"=189.5286713286714}, {"X"=490.69014084507035, "Y"=190.5314685314686}, {"X"=491.6915492957745, "Y"=190.5314685314686}, {"X"=492.6929577464788, "Y"=189.5286713286714}, {"X"=493.69436619718294, "Y"=189.5286713286714}, {"X"=494.6957746478872, "Y"=189.5286713286714}, {"X"=494.6957746478872, "Y"=188.5258741258741}, {"X"=496.69859154929566, "Y"=188.5258741258741}, {"X"=497.69999999999993, "Y"=186.52027972027975}, {"X"=498.7014084507041, "Y"=185.51748251748256}, {"X"=500.70422535211253, "Y"=183.51188811188808}, {"X"=502.70704225352097, "Y"=181.50629370629372}, {"X"=504.7098591549294, "Y"=179.50069930069935}, {"X"=505.7112676056337, "Y"=178.49790209790217}, {"X"=508.7154929577464, "Y"=175.4895104895105}, {"X"=509.71690140845055, "Y"=173.48391608391614}, {"X"=510.71830985915483, "Y"=172.48111888111896}, {"X"=511.719718309859, "Y"=169.4727272727273}, {"X"=513.7225352112674, "Y"=167.46713286713293}, {"X"=514.7239436619717, "Y"=165.46153846153845}, {"X"=515.725352112676, "Y"=164.45874125874127}, {"X"=516.7267605633801, "Y"=162.4531468531469}, {"X"=518.7295774647886, "Y"=159.44475524475524}, {"X"=520.732394366197, "Y"=156.4363636363637}, {"X"=521.7338028169013, "Y"=155.4335664335665}, {"X"=523.7366197183097, "Y"=152.42517482517485}, {"X"=524.738028169014, "Y"=150.41958041958048}, {"X"=525.7394366197182, "Y"=148.413986013986}, {"X"=526.7408450704224, "Y"=147.41118881118882}, {"X"=527.7422535211266, "Y"=146.40839160839164}, {"X"=528.7436619718309, "Y"=144.40279720279727}, {"X"=530.7464788732393, "Y"=143.39999999999998}, {"X"=531.7478873239436, "Y"=142.3972027972028}, {"X"=532.7492957746477, "Y"=141.3944055944056}, {"X"=534.7521126760562, "Y"=138.38601398601406}, {"X"=535.7535211267605, "Y"=137.38321678321677}, {"X"=536.7549295774646, "Y"=136.38041958041958}, {"X"=536.7549295774646, "Y"=135.3776223776224}, {"X"=537.7563380281689, "Y"=134.37482517482522}, {"X"=538.7577464788731, "Y"=132.36923076923085}, {"X"=539.7591549295773, "Y"=130.36363636363637}, {"X"=541.7619718309858, "Y"=128.358041958042}, {"X"=541.7619718309858, "Y"=127.35524475524483}, {"X"=542.76338028169, "Y"=126.35244755244753}, {"X"=543.7647887323942, "Y"=125.34965034965035}, {"X"=544.7661971830985, "Y"=124.34685314685316}, {"X"=544.7661971830985, "Y"=123.34405594405598}, {"X"=544.7661971830985, "Y"=122.3412587412588}, {"X"=545.7676056338026, "Y"=122.3412587412588}, {"X"=545.7676056338026, "Y"=121.33846153846162}, {"X"=546.7690140845069, "Y"=121.33846153846162}, {"X"=546.7690140845069, "Y"=120.33566433566432}, {"X"=601.8464788732393, "Y"=129.3608391608392}, {"X"=601.8464788732393, "Y"=131.36643356643356}, {"X"=604.8507042253519, "Y"=127.35524475524483}, {"X"=605.8521126760562, "Y"=126.35244755244753}, {"X"=605.8521126760562, "Y"=125.34965034965035}, {"X"=605.8521126760562, "Y"=124.34685314685316}, {"X"=604.8507042253519, "Y"=123.34405594405598}, {"X"=604.8507042253519, "Y"=122.3412587412588}, {"X"=603.8492957746478, "Y"=122.3412587412588}, {"X"=602.8478873239435, "Y"=122.3412587412588}, {"X"=602.8478873239435, "Y"=121.33846153846162}, {"X"=601.8464788732393, "Y"=121.33846153846162}, {"X"=600.8450704225351, "Y"=121.33846153846162}, {"X"=599.8436619718308, "Y"=121.33846153846162}, {"X"=598.8422535211266, "Y"=121.33846153846162}, {"X"=597.8408450704223, "Y"=121.33846153846162}, {"X"=596.8394366197182, "Y"=122.3412587412588}, {"X"=594.8366197183097, "Y"=122.3412587412588}, {"X"=592.8338028169013, "Y"=122.3412587412588}, {"X"=592.8338028169013, "Y"=123.34405594405598}, {"X"=589.8295774647886, "Y"=124.34685314685316}, {"X"=588.8281690140843, "Y"=125.34965034965035}, {"X"=586.8253521126759, "Y"=125.34965034965035}, {"X"=583.8211267605633, "Y"=126.35244755244753}, {"X"=582.819718309859, "Y"=127.35524475524483}, {"X"=580.8169014084506, "Y"=128.358041958042}, {"X"=578.8140845070421, "Y"=129.3608391608392}, {"X"=576.8112676056337, "Y"=130.36363636363637}, {"X"=573.807042253521, "Y"=132.36923076923085}, {"X"=572.8056338028167, "Y"=133.37202797202804}, {"X"=571.8042253521126, "Y"=135.3776223776224}, {"X"=570.8028169014083, "Y"=135.3776223776224}, {"X"=568.7999999999998, "Y"=137.38321678321677}, {"X"=567.7985915492957, "Y"=138.38601398601406}, {"X"=566.7971830985914, "Y"=140.39160839160843}, {"X"=565.7957746478872, "Y"=141.3944055944056}, {"X"=563.7929577464787, "Y"=143.39999999999998}, {"X"=562.7915492957745, "Y"=144.40279720279727}, {"X"=560.7887323943661, "Y"=145.40559440559446}, {"X"=559.7873239436618, "Y"=146.40839160839164}, {"X"=558.7859154929577, "Y"=147.41118881118882}, {"X"=557.7845070422534, "Y"=148.413986013986}, {"X"=557.7845070422534, "Y"=149.4167832167833}, {"X"=556.7830985915491, "Y"=150.41958041958048}, {"X"=554.7802816901407, "Y"=152.42517482517485}, {"X"=553.7788732394365, "Y"=154.43076923076922}, {"X"=552.7774647887322, "Y"=156.4363636363637}, {"X"=551.7760563380281, "Y"=157.43916083916088}, {"X"=550.7746478873238, "Y"=159.44475524475524}, {"X"=549.7732394366196, "Y"=161.45034965034972}, {"X"=549.7732394366196, "Y"=162.4531468531469}, {"X"=547.7704225352111, "Y"=165.46153846153845}, {"X"=546.7690140845069, "Y"=167.46713286713293}, {"X"=546.7690140845069, "Y"=169.4727272727273}, {"X"=545.7676056338026, "Y"=170.47552447552448}, {"X"=544.7661971830985, "Y"=171.47832167832166}, {"X"=544.7661971830985, "Y"=173.48391608391614}, {"X"=543.7647887323942, "Y"=174.48671328671333}, {"X"=542.76338028169, "Y"=176.4923076923077}, {"X"=542.76338028169, "Y"=178.49790209790217}, {"X"=541.7619718309858, "Y"=180.50349650349654}, {"X"=541.7619718309858, "Y"=181.50629370629372}, {"X"=542.76338028169, "Y"=181.50629370629372}, {"X"=542.76338028169, "Y"=183.51188811188808}, {"X"=542.76338028169, "Y"=185.51748251748256}, {"X"=543.7647887323942, "Y"=186.52027972027975}, {"X"=544.7661971830985, "Y"=187.52307692307693}, {"X"=546.7690140845069, "Y"=187.52307692307693}, {"X"=547.7704225352111, "Y"=187.52307692307693}, {"X"=548.7718309859154, "Y"=188.5258741258741}, {"X"=551.7760563380281, "Y"=188.5258741258741}, {"X"=552.7774647887322, "Y"=188.5258741258741}, {"X"=554.7802816901407, "Y"=188.5258741258741}, {"X"=556.7830985915491, "Y"=187.52307692307693}, {"X"=558.7859154929577, "Y"=187.52307692307693}, {"X"=560.7887323943661, "Y"=186.52027972027975}, {"X"=562.7915492957745, "Y"=185.51748251748256}, {"X"=564.794366197183, "Y"=183.51188811188808}, {"X"=567.7985915492957, "Y"=181.50629370629372}, {"X"=568.7999999999998, "Y"=180.50349650349654}, {"X"=569.8014084507041, "Y"=178.49790209790217}, {"X"=570.8028169014083, "Y"=176.4923076923077}, {"X"=571.8042253521126, "Y"=173.48391608391614}, {"X"=572.8056338028167, "Y"=172.48111888111896}, {"X"=572.8056338028167, "Y"=170.47552447552448}, {"X"=572.8056338028167, "Y"=169.4727272727273}, {"X"=572.8056338028167, "Y"=168.46993006993011}, {"X"=572.8056338028167, "Y"=165.46153846153845}, {"X"=572.8056338028167, "Y"=164.45874125874127}, {"X"=572.8056338028167, "Y"=163.4559440559441}, {"X"=571.8042253521126, "Y"=163.4559440559441}, {"X"=571.8042253521126, "Y"=162.4531468531469}, {"X"=571.8042253521126, "Y"=161.45034965034972}, {"X"=570.8028169014083, "Y"=160.44755244755243}, {"X"=570.8028169014083, "Y"=159.44475524475524}, {"X"=570.8028169014083, "Y"=158.44195804195806}, {"X"=570.8028169014083, "Y"=159.44475524475524}, {"X"=571.8042253521126, "Y"=159.44475524475524}, {"X"=572.8056338028167, "Y"=160.44755244755243}, {"X"=573.807042253521, "Y"=160.44755244755243}, {"X"=574.8084507042253, "Y"=160.44755244755243}, {"X"=575.8098591549294, "Y"=160.44755244755243}, {"X"=576.8112676056337, "Y"=160.44755244755243}, {"X"=578.8140845070421, "Y"=160.44755244755243}, {"X"=580.8169014084506, "Y"=160.44755244755243}, {"X"=581.8183098591547, "Y"=160.44755244755243}, {"X"=583.8211267605633, "Y"=160.44755244755243}, {"X"=585.8239436619717, "Y"=160.44755244755243}, {"X"=586.8253521126759, "Y"=160.44755244755243}, {"X"=588.8281690140843, "Y"=161.45034965034972}, {"X"=589.8295774647886, "Y"=161.45034965034972}, {"X"=589.8295774647886, "Y"=162.4531468531469}, {"X"=590.8309859154928, "Y"=162.4531468531469}, {"X"=591.832394366197, "Y"=162.4531468531469}, {"X"=591.832394366197, "Y"=163.4559440559441}, {"X"=593.8352112676055, "Y"=163.4559440559441}, {"X"=594.8366197183097, "Y"=163.4559440559441}, {"X"=595.8380281690139, "Y"=163.4559440559441}, {"X"=595.8380281690139, "Y"=162.4531468531469}, {"X"=595.8380281690139, "Y"=163.4559440559441}, {"X"=595.8380281690139, "Y"=162.4531468531469}, {"X"=595.8380281690139, "Y"=163.4559440559441}, {"X"=593.8352112676055, "Y"=165.46153846153845}, {"X"=592.8338028169013, "Y"=168.46993006993011}, {"X"=590.8309859154928, "Y"=171.47832167832166}, {"X"=588.8281690140843, "Y"=174.48671328671333}, {"X"=587.8267605633802, "Y"=176.4923076923077}, {"X"=585.8239436619717, "Y"=179.50069930069935}, {"X"=585.8239436619717, "Y"=181.50629370629372}, {"X"=584.8225352112674, "Y"=181.50629370629372}, {"X"=584.8225352112674, "Y"=182.5090909090909}, {"X"=584.8225352112674, "Y"=183.51188811188808}, {"X"=583.8211267605633, "Y"=183.51188811188808}, {"X"=583.8211267605633, "Y"=184.51468531468538}, {"X"=583.8211267605633, "Y"=185.51748251748256}, {"X"=582.819718309859, "Y"=185.51748251748256}, {"X"=582.819718309859, "Y"=186.52027972027975}, {"X"=581.8183098591547, "Y"=187.52307692307693}, {"X"=581.8183098591547, "Y"=188.5258741258741}, {"X"=580.8169014084506, "Y"=188.5258741258741}, {"X"=580.8169014084506, "Y"=187.52307692307693}, {"X"=582.819718309859, "Y"=187.52307692307693}, {"X"=591.832394366197, "Y"=187.52307692307693}, {"X"=593.8352112676055, "Y"=187.52307692307693}, {"X"=594.8366197183097, "Y"=187.52307692307693}, {"X"=595.8380281690139, "Y"=187.52307692307693}, {"X"=596.8394366197182, "Y"=186.52027972027975}, {"X"=599.8436619718308, "Y"=186.52027972027975}, {"X"=603.8492957746478, "Y"=185.51748251748256}, {"X"=604.8507042253519, "Y"=184.51468531468538}, {"X"=607.8549295774646, "Y"=183.51188811188808}, {"X"=609.8577464788731, "Y"=182.5090909090909}, {"X"=611.8605633802815, "Y"=182.5090909090909}, {"X"=614.8647887323942, "Y"=181.50629370629372}, {"X"=616.8676056338027, "Y"=180.50349650349654}, {"X"=617.869014084507, "Y"=180.50349650349654}, {"X"=619.8718309859154, "Y"=179.50069930069935}, {"X"=621.8746478873238, "Y"=178.49790209790217}, {"X"=624.8788732394364, "Y"=177.49510489510487}, {"X"=625.8802816901407, "Y"=176.4923076923077}, {"X"=626.881690140845, "Y"=176.4923076923077}, {"X"=627.8830985915491, "Y"=175.4895104895105}, {"X"=628.8845070422534, "Y"=175.4895104895105}, {"X"=629.8859154929576, "Y"=175.4895104895105}, {"X"=630.8873239436618, "Y"=174.48671328671333}, {"X"=631.888732394366, "Y"=174.48671328671333}, {"X"=632.8901408450703, "Y"=174.48671328671333}, {"X"=631.888732394366, "Y"=174.48671328671333}, {"X"=629.8859154929576, "Y"=174.48671328671333}, {"X"=624.8788732394364, "Y"=176.4923076923077}, {"X"=621.8746478873238, "Y"=177.49510489510487}, {"X"=619.8718309859154, "Y"=178.49790209790217}, {"X"=615.8661971830984, "Y"=180.50349650349654}, {"X"=613.86338028169, "Y"=181.50629370629372}, {"X"=612.8619718309858, "Y"=181.50629370629372}, {"X"=610.8591549295774, "Y"=183.51188811188808}, {"X"=609.8577464788731, "Y"=183.51188811188808}, {"X"=608.8563380281689, "Y"=183.51188811188808}, {"X"=608.8563380281689, "Y"=184.51468531468538}, {"X"=607.8549295774646, "Y"=184.51468531468538}, {"X"=607.8549295774646, "Y"=183.51188811188808}, {"X"=609.8577464788731, "Y"=182.5090909090909}, {"X"=610.8591549295774, "Y"=180.50349650349654}, {"X"=611.8605633802815, "Y"=177.49510489510487}, {"X"=612.8619718309858, "Y"=175.4895104895105}, {"X"=612.8619718309858, "Y"=173.48391608391614}, {"X"=614.8647887323942, "Y"=170.47552447552448}, {"X"=614.8647887323942, "Y"=169.4727272727273}, {"X"=615.8661971830984, "Y"=166.46433566433564}, {"X"=616.8676056338027, "Y"=164.45874125874127}, {"X"=617.869014084507, "Y"=162.4531468531469}, {"X"=617.869014084507, "Y"=160.44755244755243}, {"X"=618.8704225352111, "Y"=159.44475524475524}, {"X"=619.8718309859154, "Y"=156.4363636363637}, {"X"=621.8746478873238, "Y"=152.42517482517485}, {"X"=622.876056338028, "Y"=151.42237762237767}, {"X"=622.876056338028, "Y"=150.41958041958048}, {"X"=624.8788732394364, "Y"=147.41118881118882}, {"X"=626.881690140845, "Y"=145.40559440559446}, {"X"=627.8830985915491, "Y"=142.3972027972028}, {"X"=628.8845070422534, "Y"=141.3944055944056}, {"X"=629.8859154929576, "Y"=139.38881118881125}, {"X"=630.8873239436618, "Y"=136.38041958041958}, {"X"=631.888732394366, "Y"=136.38041958041958}, {"X"=631.888732394366, "Y"=135.3776223776224}, {"X"=632.8901408450703, "Y"=135.3776223776224}, {"X"=632.8901408450703, "Y"=134.37482517482522}, {"X"=632.8901408450703, "Y"=133.37202797202804}, {"X"=633.8915492957744, "Y"=133.37202797202804}, {"X"=632.8901408450703, "Y"=133.37202797202804}, {"X"=631.888732394366, "Y"=133.37202797202804}, {"X"=630.8873239436618, "Y"=133.37202797202804}, {"X"=629.8859154929576, "Y"=134.37482517482522}, {"X"=628.8845070422534, "Y"=134.37482517482522}, {"X"=624.8788732394364, "Y"=135.3776223776224}, {"X"=621.8746478873238, "Y"=135.3776223776224}, {"X"=618.8704225352111, "Y"=136.38041958041958}, {"X"=615.8661971830984, "Y"=136.38041958041958}, {"X"=612.8619718309858, "Y"=136.38041958041958}, {"X"=610.8591549295774, "Y"=137.38321678321677}, {"X"=609.8577464788731, "Y"=137.38321678321677}, {"X"=608.8563380281689, "Y"=137.38321678321677}, {"X"=607.8549295774646, "Y"=137.38321678321677}, {"X"=606.8535211267604, "Y"=138.38601398601406}, {"X"=605.8521126760562, "Y"=138.38601398601406}, {"X"=606.8535211267604, "Y"=138.38601398601406}, {"X"=607.8549295774646, "Y"=137.38321678321677}, {"X"=608.8563380281689, "Y"=137.38321678321677}, {"X"=609.8577464788731, "Y"=137.38321678321677}, {"X"=612.8619718309858, "Y"=137.38321678321677}, {"X"=615.8661971830984, "Y"=136.38041958041958}, {"X"=619.8718309859154, "Y"=135.3776223776224}, {"X"=623.8774647887323, "Y"=134.37482517482522}, {"X"=627.8830985915491, "Y"=133.37202797202804}, {"X"=631.888732394366, "Y"=133.37202797202804}, {"X"=637.8971830985914, "Y"=132.36923076923085}, {"X"=641.9028169014083, "Y"=131.36643356643356}, {"X"=645.9084507042252, "Y"=130.36363636363637}, {"X"=649.914084507042, "Y"=130.36363636363637}, {"X"=651.9169014084506, "Y"=129.3608391608392}, {"X"=653.919718309859, "Y"=129.3608391608392}, {"X"=655.9225352112675, "Y"=129.3608391608392}, {"X"=656.9239436619716, "Y"=129.3608391608392}, {"X"=657.9253521126759, "Y"=129.3608391608392}, {"X"=658.9267605633801, "Y"=129.3608391608392}, {"X"=659.9281690140843, "Y"=129.3608391608392}, {"X"=660.9295774647886, "Y"=129.3608391608392}, {"X"=661.9309859154928, "Y"=129.3608391608392}, {"X"=662.9323943661971, "Y"=129.3608391608392}, {"X"=662.9323943661971, "Y"=130.36363636363637}, {"X"=661.9309859154928, "Y"=130.36363636363637}, {"X"=661.9309859154928, "Y"=129.3608391608392}, {"X"=630.8873239436618, "Y"=134.37482517482522}, {"X"=608.8563380281689, "Y"=174.48671328671333}, {"X"=631.888732394366, "Y"=172.48111888111896}, {"X"=637.8971830985914, "Y"=174.48671328671333}, {"X"=640.901408450704, "Y"=176.4923076923077}, {"X"=641.9028169014083, "Y"=175.4895104895105}, {"X"=642.9042253521126, "Y"=174.48671328671333}, {"X"=643.9056338028167, "Y"=174.48671328671333}, {"X"=646.9098591549294, "Y"=172.48111888111896}, {"X"=649.914084507042, "Y"=170.47552447552448}, {"X"=651.9169014084506, "Y"=168.46993006993011}, {"X"=653.919718309859, "Y"=166.46433566433564}, {"X"=653.919718309859, "Y"=165.46153846153845}, {"X"=654.9211267605632, "Y"=164.45874125874127}, {"X"=656.9239436619716, "Y"=163.4559440559441}, {"X"=657.9253521126759, "Y"=161.45034965034972}, {"X"=659.9281690140843, "Y"=160.44755244755243}, {"X"=660.9295774647886, "Y"=158.44195804195806}, {"X"=663.9338028169012, "Y"=156.4363636363637}, {"X"=664.9352112676055, "Y"=154.43076923076922}, {"X"=665.9366197183097, "Y"=153.42797202797203}, {"X"=667.9394366197181, "Y"=153.42797202797203}, {"X"=668.9408450704224, "Y"=151.42237762237767}, {"X"=670.9436619718308, "Y"=150.41958041958048}, {"X"=672.9464788732392, "Y"=148.413986013986}, {"X"=675.950704225352, "Y"=147.41118881118882}, {"X"=677.9535211267604, "Y"=146.40839160839164}, {"X"=678.9549295774647, "Y"=145.40559440559446}, {"X"=679.9563380281688, "Y"=144.40279720279727}, {"X"=682.9605633802815, "Y"=140.39160839160843}, {"X"=683.9619718309857, "Y"=140.39160839160843}, {"X"=683.9619718309857, "Y"=139.38881118881125}, {"X"=684.96338028169, "Y"=139.38881118881125}, {"X"=684.96338028169, "Y"=138.38601398601406}, {"X"=685.9647887323943, "Y"=138.38601398601406}, {"X"=685.9647887323943, "Y"=137.38321678321677}, {"X"=685.9647887323943, "Y"=136.38041958041958}, {"X"=685.9647887323943, "Y"=137.38321678321677}, {"X"=685.9647887323943, "Y"=138.38601398601406}, {"X"=684.96338028169, "Y"=139.38881118881125}, {"X"=684.96338028169, "Y"=140.39160839160843}, {"X"=683.9619718309857, "Y"=141.3944055944056}, {"X"=683.9619718309857, "Y"=143.39999999999998}, {"X"=681.9591549295773, "Y"=147.41118881118882}, {"X"=681.9591549295773, "Y"=149.4167832167833}, {"X"=680.9577464788731, "Y"=151.42237762237767}, {"X"=679.9563380281688, "Y"=154.43076923076922}, {"X"=679.9563380281688, "Y"=156.4363636363637}, {"X"=678.9549295774647, "Y"=157.43916083916088}, {"X"=678.9549295774647, "Y"=158.44195804195806}, {"X"=678.9549295774647, "Y"=159.44475524475524}, {"X"=678.9549295774647, "Y"=160.44755244755243}, {"X"=678.9549295774647, "Y"=161.45034965034972}, {"X"=678.9549295774647, "Y"=162.4531468531469}, {"X"=678.9549295774647, "Y"=163.4559440559441}, {"X"=679.9563380281688, "Y"=163.4559440559441}, {"X"=679.9563380281688, "Y"=164.45874125874127}, {"X"=680.9577464788731, "Y"=164.45874125874127}, {"X"=681.9591549295773, "Y"=163.4559440559441}, {"X"=683.9619718309857, "Y"=163.4559440559441}, {"X"=685.9647887323943, "Y"=162.4531468531469}, {"X"=688.9690140845069, "Y"=160.44755244755243}, {"X"=688.9690140845069, "Y"=159.44475524475524}, {"X"=691.9732394366196, "Y"=157.43916083916088}, {"X"=693.976056338028, "Y"=155.4335664335665}, {"X"=694.9774647887323, "Y"=154.43076923076922}, {"X"=696.9802816901407, "Y"=154.43076923076922}, {"X"=698.9830985915492, "Y"=152.42517482517485}, {"X"=700.9859154929576, "Y"=151.42237762237767}, {"X"=703.9901408450703, "Y"=149.4167832167833}, {"X"=704.9915492957745, "Y"=149.4167832167833}, {"X"=707.9957746478872, "Y"=147.41118881118882}, {"X"=710.9999999999998, "Y"=145.40559440559446}, {"X"=713.0028169014083, "Y"=143.39999999999998}, {"X"=715.0056338028168, "Y"=142.3972027972028}, {"X"=717.0084507042252, "Y"=141.3944055944056}, {"X"=719.0112676056336, "Y"=139.38881118881125}, {"X"=721.0140845070421, "Y"=137.38321678321677}, {"X"=724.0183098591548, "Y"=136.38041958041958}, {"X"=726.0211267605632, "Y"=133.37202797202804}, {"X"=728.0239436619717, "Y"=131.36643356643356}, {"X"=729.0253521126759, "Y"=130.36363636363637}, {"X"=730.0267605633801, "Y"=130.36363636363637}, {"X"=731.0281690140844, "Y"=128.358041958042}, {"X"=732.0295774647885, "Y"=127.35524475524483}, {"X"=733.0309859154928, "Y"=126.35244755244753}, {"X"=733.0309859154928, "Y"=125.34965034965035}, {"X"=734.032394366197, "Y"=124.34685314685316}, {"X"=734.032394366197, "Y"=123.34405594405598}, {"X"=734.032394366197, "Y"=122.3412587412588}, {"X"=735.0338028169012, "Y"=122.3412587412588}, {"X"=739.0394366197181, "Y"=126.35244755244753}, {"X"=737.0366197183097, "Y"=130.36363636363637}, {"X"=736.0352112676054, "Y"=131.36643356643356}, {"X"=736.0352112676054, "Y"=132.36923076923085}, {"X"=735.0338028169012, "Y"=133.37202797202804}, {"X"=734.032394366197, "Y"=135.3776223776224}, {"X"=733.0309859154928, "Y"=137.38321678321677}, {"X"=731.0281690140844, "Y"=140.39160839160843}, {"X"=730.0267605633801, "Y"=144.40279720279727}, {"X"=729.0253521126759, "Y"=145.40559440559446}, {"X"=728.0239436619717, "Y"=147.41118881118882}, {"X"=728.0239436619717, "Y"=149.4167832167833}, {"X"=727.0225352112674, "Y"=149.4167832167833}, {"X"=727.0225352112674, "Y"=150.41958041958048}, {"X"=727.0225352112674, "Y"=151.42237762237767}, {"X"=726.0211267605632, "Y"=152.42517482517485}, {"X"=726.0211267605632, "Y"=153.42797202797203}, {"X"=726.0211267605632, "Y"=154.43076923076922}, {"X"=725.019718309859, "Y"=154.43076923076922}, {"X"=725.019718309859, "Y"=156.4363636363637}, {"X"=725.019718309859, "Y"=157.43916083916088}, {"X"=724.0183098591548, "Y"=158.44195804195806}, {"X"=724.0183098591548, "Y"=160.44755244755243}, {"X"=724.0183098591548, "Y"=161.45034965034972}, {"X"=723.0169014084505, "Y"=161.45034965034972}, {"X"=724.0183098591548, "Y"=161.45034965034972}, {"X"=724.0183098591548, "Y"=162.4531468531469}, {"X"=724.0183098591548, "Y"=163.4559440559441}, {"X"=725.019718309859, "Y"=163.4559440559441}, {"X"=725.019718309859, "Y"=164.45874125874127}, {"X"=726.0211267605632, "Y"=164.45874125874127}, {"X"=727.0225352112674, "Y"=164.45874125874127}, {"X"=728.0239436619717, "Y"=164.45874125874127}, {"X"=729.0253521126759, "Y"=164.45874125874127}, {"X"=731.0281690140844, "Y"=164.45874125874127}, {"X"=733.0309859154928, "Y"=164.45874125874127}, {"X"=736.0352112676054, "Y"=163.4559440559441}, {"X"=737.0366197183097, "Y"=163.4559440559441}, {"X"=740.0408450704224, "Y"=163.4559440559441}, {"X"=743.045070422535, "Y"=162.4531468531469}, {"X"=745.0478873239434, "Y"=162.4531468531469}, {"X"=748.0521126760561, "Y"=162.4531468531469}, {"X"=750.0549295774646, "Y"=162.4531468531469}, {"X"=753.0591549295773, "Y"=161.45034965034972}, {"X"=755.0619718309857, "Y"=161.45034965034972}, {"X"=757.0647887323942, "Y"=161.45034965034972}, {"X"=760.0690140845069, "Y"=160.44755244755243}, {"X"=762.0718309859153, "Y"=160.44755244755243}, {"X"=763.0732394366196, "Y"=160.44755244755243}, {"X"=764.0746478873237, "Y"=160.44755244755243}, {"X"=766.0774647887322, "Y"=160.44755244755243}, {"X"=767.0788732394365, "Y"=160.44755244755243}, {"X"=768.0802816901406, "Y"=159.44475524475524}, {"X"=769.0816901408449, "Y"=159.44475524475524}, {"X"=769.0816901408449, "Y"=158.44195804195806}, {"X"=770.0830985915491, "Y"=158.44195804195806}, {"X"=771.0845070422533, "Y"=157.43916083916088}, {"X"=772.0859154929576, "Y"=157.43916083916088}, {"X"=770.0830985915491, "Y"=157.43916083916088}, {"X"=768.0802816901406, "Y"=158.44195804195806}, {"X"=766.0774647887322, "Y"=158.44195804195806}, {"X"=763.0732394366196, "Y"=159.44475524475524}, {"X"=760.0690140845069, "Y"=160.44755244755243}, {"X"=756.06338028169, "Y"=160.44755244755243}, {"X"=754.0605633802816, "Y"=161.45034965034972}, {"X"=750.0549295774646, "Y"=161.45034965034972}, {"X"=747.050704225352, "Y"=161.45034965034972}, {"X"=746.0492957746477, "Y"=162.4531468531469}, {"X"=742.0436619718308, "Y"=163.4559440559441}, {"X"=740.0408450704224, "Y"=163.4559440559441}, {"X"=739.0394366197181, "Y"=163.4559440559441}, {"X"=736.0352112676054, "Y"=163.4559440559441}, {"X"=735.0338028169012, "Y"=163.4559440559441}, {"X"=733.0309859154928, "Y"=164.45874125874127}, {"X"=732.0295774647885, "Y"=164.45874125874127}, {"X"=731.0281690140844, "Y"=164.45874125874127}, {"X"=729.0253521126759, "Y"=164.45874125874127}, {"X"=728.0239436619717, "Y"=164.45874125874127}, {"X"=727.0225352112674, "Y"=164.45874125874127}, {"X"=727.0225352112674, "Y"=163.4559440559441}, {"X"=727.0225352112674, "Y"=164.45874125874127}, {"X"=726.0211267605632, "Y"=163.4559440559441}, {"X"=725.019718309859, "Y"=161.45034965034972}, {"X"=725.019718309859, "Y"=160.44755244755243}, {"X"=725.019718309859, "Y"=159.44475524475524}, {"X"=725.019718309859, "Y"=157.43916083916088}, {"X"=725.019718309859, "Y"=156.4363636363637}, {"X"=726.0211267605632, "Y"=154.43076923076922}, {"X"=726.0211267605632, "Y"=153.42797202797203}, {"X"=727.0225352112674, "Y"=151.42237762237767}, {"X"=728.0239436619717, "Y"=148.413986013986}, {"X"=728.0239436619717, "Y"=147.41118881118882}, {"X"=728.0239436619717, "Y"=146.40839160839164}, {"X"=729.0253521126759, "Y"=146.40839160839164}, {"X"=729.0253521126759, "Y"=145.40559440559446}, {"X"=729.0253521126759, "Y"=144.40279720279727}, {"X"=729.0253521126759, "Y"=143.39999999999998}, {"X"=729.0253521126759, "Y"=144.40279720279727}, {"X"=730.0267605633801, "Y"=144.40279720279727}, {"X"=731.0281690140844, "Y"=144.40279720279727}, {"X"=732.0295774647885, "Y"=144.40279720279727}, {"X"=733.0309859154928, "Y"=144.40279720279727}, {"X"=734.032394366197, "Y"=144.40279720279727}, {"X"=738.038028169014, "Y"=144.40279720279727}, {"X"=741.0422535211266, "Y"=143.39999999999998}, {"X"=743.045070422535, "Y"=143.39999999999998}, {"X"=746.0492957746477, "Y"=142.3972027972028}, {"X"=750.0549295774646, "Y"=142.3972027972028}, {"X"=751.0563380281689, "Y"=141.3944055944056}, {"X"=753.0591549295773, "Y"=141.3944055944056}, {"X"=755.0619718309857, "Y"=141.3944055944056}, {"X"=757.0647887323942, "Y"=141.3944055944056}, {"X"=758.0661971830984, "Y"=140.39160839160843}, {"X"=759.0676056338026, "Y"=140.39160839160843}, {"X"=760.0690140845069, "Y"=140.39160839160843}, {"X"=761.070422535211, "Y"=140.39160839160843}, {"X"=762.0718309859153, "Y"=140.39160839160843}, {"X"=763.0732394366196, "Y"=140.39160839160843}, {"X"=764.0746478873237, "Y"=140.39160839160843}, {"X"=764.0746478873237, "Y"=139.38881118881125}, {"X"=765.076056338028, "Y"=139.38881118881125}, {"X"=766.0774647887322, "Y"=139.38881118881125}, {"X"=766.0774647887322, "Y"=138.38601398601406}, {"X"=766.0774647887322, "Y"=139.38881118881125}, {"X"=765.076056338028, "Y"=139.38881118881125}, {"X"=763.0732394366196, "Y"=139.38881118881125}, {"X"=763.0732394366196, "Y"=140.39160839160843}, {"X"=762.0718309859153, "Y"=140.39160839160843}, {"X"=759.0676056338026, "Y"=140.39160839160843}, {"X"=757.0647887323942, "Y"=141.3944055944056}, {"X"=751.0563380281689, "Y"=142.3972027972028}, {"X"=747.050704225352, "Y"=143.39999999999998}, {"X"=744.0464788732393, "Y"=143.39999999999998}, {"X"=741.0422535211266, "Y"=143.39999999999998}, {"X"=740.0408450704224, "Y"=144.40279720279727}, {"X"=739.0394366197181, "Y"=144.40279720279727}, {"X"=738.038028169014, "Y"=144.40279720279727}, {"X"=737.0366197183097, "Y"=144.40279720279727}, {"X"=736.0352112676054, "Y"=144.40279720279727}, {"X"=735.0338028169012, "Y"=145.40559440559446}, {"X"=734.032394366197, "Y"=145.40559440559446}, {"X"=733.0309859154928, "Y"=145.40559440559446}, {"X"=732.0295774647885, "Y"=145.40559440559446}, {"X"=731.0281690140844, "Y"=145.40559440559446}, {"X"=731.0281690140844, "Y"=146.40839160839164}, {"X"=730.0267605633801, "Y"=145.40559440559446}, {"X"=730.0267605633801, "Y"=143.39999999999998}, {"X"=731.0281690140844, "Y"=142.3972027972028}, {"X"=731.0281690140844, "Y"=140.39160839160843}, {"X"=733.0309859154928, "Y"=137.38321678321677}, {"X"=734.032394366197, "Y"=135.3776223776224}, {"X"=735.0338028169012, "Y"=133.37202797202804}, {"X"=736.0352112676054, "Y"=132.36923076923085}, {"X"=736.0352112676054, "Y"=131.36643356643356}, {"X"=737.0366197183097, "Y"=131.36643356643356}, {"X"=737.0366197183097, "Y"=129.3608391608392}, {"X"=738.038028169014, "Y"=128.358041958042}, {"X"=738.038028169014, "Y"=127.35524475524483}, {"X"=739.0394366197181, "Y"=127.35524475524483}, {"X"=739.0394366197181, "Y"=126.35244755244753}, {"X"=739.0394366197181, "Y"=125.34965034965035}, {"X"=739.0394366197181, "Y"=124.34685314685316}, {"X"=740.0408450704224, "Y"=124.34685314685316}, {"X"=740.0408450704224, "Y"=123.34405594405598}, {"X"=741.0422535211266, "Y"=123.34405594405598}, {"X"=742.0436619718308, "Y"=123.34405594405598}, {"X"=743.045070422535, "Y"=123.34405594405598}, {"X"=744.0464788732393, "Y"=122.3412587412588}, {"X"=747.050704225352, "Y"=122.3412587412588}, {"X"=748.0521126760561, "Y"=121.33846153846162}, {"X"=749.0535211267604, "Y"=121.33846153846162}, {"X"=753.0591549295773, "Y"=120.33566433566432}, {"X"=756.06338028169, "Y"=120.33566433566432}, {"X"=758.0661971830984, "Y"=120.33566433566432}, {"X"=760.0690140845069, "Y"=119.33286713286714}, {"X"=763.0732394366196, "Y"=119.33286713286714}, {"X"=764.0746478873237, "Y"=118.33006993006995}, {"X"=768.0802816901406, "Y"=117.32727272727277}, {"X"=770.0830985915491, "Y"=117.32727272727277}, {"X"=772.0859154929576, "Y"=117.32727272727277}, {"X"=774.088732394366, "Y"=117.32727272727277}, {"X"=776.0915492957745, "Y"=117.32727272727277}, {"X"=777.0929577464786, "Y"=117.32727272727277}, {"X"=778.0943661971829, "Y"=116.32447552447559}, {"X"=779.0957746478871, "Y"=116.32447552447559}, {"X"=780.0971830985914, "Y"=116.32447552447559}, {"X"=781.0985915492956, "Y"=116.32447552447559}, {"X"=782.0999999999998, "Y"=116.32447552447559}, {"X"=783.1014084507041, "Y"=116.32447552447559}, {"X"=784.1028169014082, "Y"=116.32447552447559}, {"X"=783.1014084507041, "Y"=116.32447552447559}, {"X"=782.0999999999998, "Y"=115.3216783216784}, {"X"=799.1239436619717, "Y"=120.33566433566432}, {"X"=795.1183098591547, "Y"=125.34965034965035}, {"X"=794.1169014084505, "Y"=125.34965034965035}, {"X"=793.1154929577463, "Y"=127.35524475524483}, {"X"=792.1140845070421, "Y"=128.358041958042}, {"X"=791.1126760563378, "Y"=130.36363636363637}, {"X"=790.1112676056337, "Y"=131.36643356643356}, {"X"=789.1098591549294, "Y"=133.37202797202804}, {"X"=786.1056338028167, "Y"=137.38321678321677}, {"X"=785.1042253521125, "Y"=138.38601398601406}, {"X"=785.1042253521125, "Y"=140.39160839160843}, {"X"=783.1014084507041, "Y"=142.3972027972028}, {"X"=782.0999999999998, "Y"=142.3972027972028}, {"X"=782.0999999999998, "Y"=143.39999999999998}, {"X"=781.0985915492956, "Y"=144.40279720279727}, {"X"=780.0971830985914, "Y"=146.40839160839164}, {"X"=779.0957746478871, "Y"=147.41118881118882}, {"X"=779.0957746478871, "Y"=148.413986013986}, {"X"=779.0957746478871, "Y"=149.4167832167833}, {"X"=778.0943661971829, "Y"=150.41958041958048}, {"X"=777.0929577464786, "Y"=151.42237762237767}, {"X"=777.0929577464786, "Y"=152.42517482517485}, {"X"=776.0915492957745, "Y"=152.42517482517485}, {"X"=776.0915492957745, "Y"=153.42797202797203}, {"X"=776.0915492957745, "Y"=154.43076923076922}, {"X"=776.0915492957745, "Y"=155.4335664335665}, {"X"=776.0915492957745, "Y"=156.4363636363637}, {"X"=777.0929577464786, "Y"=156.4363636363637}, {"X"=778.0943661971829, "Y"=157.43916083916088}, {"X"=779.0957746478871, "Y"=157.43916083916088}, {"X"=780.0971830985914, "Y"=157.43916083916088}, {"X"=780.0971830985914, "Y"=158.44195804195806}, {"X"=781.0985915492956, "Y"=158.44195804195806}, {"X"=783.1014084507041, "Y"=159.44475524475524}, {"X"=784.1028169014082, "Y"=159.44475524475524}, {"X"=786.1056338028167, "Y"=159.44475524475524}, {"X"=788.1084507042252, "Y"=158.44195804195806}, {"X"=790.1112676056337, "Y"=157.43916083916088}, {"X"=792.1140845070421, "Y"=157.43916083916088}, {"X"=794.1169014084505, "Y"=156.4363636363637}, {"X"=797.1211267605632, "Y"=156.4363636363637}, {"X"=800.1253521126758, "Y"=156.4363636363637}, {"X"=801.1267605633801, "Y"=155.4335664335665}, {"X"=803.1295774647886, "Y"=155.4335664335665}, {"X"=804.1309859154927, "Y"=154.43076923076922}, {"X"=805.132394366197, "Y"=154.43076923076922}, {"X"=808.1366197183097, "Y"=153.42797202797203}, {"X"=809.1380281690139, "Y"=153.42797202797203}, {"X"=810.1394366197181, "Y"=153.42797202797203}, {"X"=811.1408450704223, "Y"=153.42797202797203}, {"X"=812.1422535211266, "Y"=153.42797202797203}, {"X"=813.1436619718307, "Y"=153.42797202797203}, {"X"=814.145070422535, "Y"=153.42797202797203}, {"X"=815.1464788732393, "Y"=153.42797202797203}, {"X"=816.1478873239435, "Y"=153.42797202797203}, {"X"=817.1492957746477, "Y"=153.42797202797203}, {"X"=817.1492957746477, "Y"=154.43076923076922}, {"X"=817.1492957746477, "Y"=153.42797202797203}, {"X"=817.1492957746477, "Y"=154.43076923076922}, {"X"=817.1492957746477, "Y"=153.42797202797203}, {"X"=816.1478873239435, "Y"=153.42797202797203}, {"X"=815.1464788732393, "Y"=154.43076923076922}, {"X"=814.145070422535, "Y"=154.43076923076922}, {"X"=813.1436619718307, "Y"=154.43076923076922}, {"X"=811.1408450704223, "Y"=154.43076923076922}, {"X"=811.1408450704223, "Y"=155.4335664335665}, {"X"=810.1394366197181, "Y"=155.4335664335665}, {"X"=806.1338028169013, "Y"=156.4363636363637}, {"X"=803.1295774647886, "Y"=156.4363636363637}, {"X"=801.1267605633801, "Y"=157.43916083916088}, {"X"=799.1239436619717, "Y"=157.43916083916088}, {"X"=795.1183098591547, "Y"=157.43916083916088}, {"X"=793.1154929577463, "Y"=157.43916083916088}, {"X"=789.1098591549294, "Y"=157.43916083916088}, {"X"=787.107042253521, "Y"=157.43916083916088}, {"X"=784.1028169014082, "Y"=156.4363636363637}, {"X"=781.0985915492956, "Y"=156.4363636363637}, {"X"=780.0971830985914, "Y"=156.4363636363637}, {"X"=780.0971830985914, "Y"=155.4335664335665}, {"X"=778.0943661971829, "Y"=155.4335664335665}, {"X"=776.0915492957745, "Y"=154.43076923076922}, {"X"=775.0901408450702, "Y"=153.42797202797203}, {"X"=775.0901408450702, "Y"=152.42517482517485}, {"X"=775.0901408450702, "Y"=151.42237762237767}, {"X"=775.0901408450702, "Y"=150.41958041958048}, {"X"=775.0901408450702, "Y"=148.413986013986}, {"X"=775.0901408450702, "Y"=147.41118881118882}, {"X"=776.0915492957745, "Y"=146.40839160839164}, {"X"=777.0929577464786, "Y"=145.40559440559446}, {"X"=778.0943661971829, "Y"=145.40559440559446}, {"X"=778.0943661971829, "Y"=144.40279720279727}, {"X"=779.0957746478871, "Y"=144.40279720279727}, {"X"=780.0971830985914, "Y"=143.39999999999998}, {"X"=780.0971830985914, "Y"=142.3972027972028}, {"X"=780.0971830985914, "Y"=141.3944055944056}, {"X"=780.0971830985914, "Y"=140.39160839160843}, {"X"=781.0985915492956, "Y"=140.39160839160843}, {"X"=780.0971830985914, "Y"=140.39160839160843}, {"X"=780.0971830985914, "Y"=141.3944055944056}, {"X"=781.0985915492956, "Y"=141.3944055944056}, {"X"=782.0999999999998, "Y"=141.3944055944056}, {"X"=783.1014084507041, "Y"=141.3944055944056}, {"X"=784.1028169014082, "Y"=141.3944055944056}, {"X"=787.107042253521, "Y"=141.3944055944056}, {"X"=789.1098591549294, "Y"=141.3944055944056}, {"X"=793.1154929577463, "Y"=141.3944055944056}, {"X"=797.1211267605632, "Y"=140.39160839160843}, {"X"=802.1281690140843, "Y"=140.39160839160843}, {"X"=805.132394366197, "Y"=139.38881118881125}, {"X"=807.1352112676054, "Y"=139.38881118881125}, {"X"=810.1394366197181, "Y"=139.38881118881125}, {"X"=812.1422535211266, "Y"=138.38601398601406}, {"X"=815.1464788732393, "Y"=138.38601398601406}, {"X"=819.1521126760562, "Y"=138.38601398601406}, {"X"=820.1535211267603, "Y"=137.38321678321677}, {"X"=821.1549295774646, "Y"=137.38321678321677}, {"X"=822.1563380281688, "Y"=137.38321678321677}, {"X"=824.1591549295773, "Y"=137.38321678321677}, {"X"=826.1619718309857, "Y"=137.38321678321677}, {"X"=827.1633802816899, "Y"=137.38321678321677}, {"X"=828.1647887323942, "Y"=137.38321678321677}, {"X"=829.1661971830983, "Y"=137.38321678321677}, {"X"=830.1676056338026, "Y"=137.38321678321677}, {"X"=831.1690140845069, "Y"=137.38321678321677}, {"X"=831.1690140845069, "Y"=136.38041958041958}, {"X"=832.1704225352111, "Y"=136.38041958041958}, {"X"=832.1704225352111, "Y"=136.38041958041958}, {"X"=830.1676056338026, "Y"=136.38041958041958}, {"X"=828.1647887323942, "Y"=137.38321678321677}, {"X"=821.1549295774646, "Y"=138.38601398601406}, {"X"=816.1478873239435, "Y"=138.38601398601406}, {"X"=809.1380281690139, "Y"=140.39160839160843}, {"X"=806.1338028169013, "Y"=140.39160839160843}, {"X"=800.1253521126758, "Y"=141.3944055944056}, {"X"=797.1211267605632, "Y"=141.3944055944056}, {"X"=795.1183098591547, "Y"=142.3972027972028}, {"X"=792.1140845070421, "Y"=142.3972027972028}, {"X"=789.1098591549294, "Y"=142.3972027972028}, {"X"=788.1084507042252, "Y"=142.3972027972028}, {"X"=787.107042253521, "Y"=142.3972027972028}, {"X"=786.1056338028167, "Y"=142.3972027972028}, {"X"=785.1042253521125, "Y"=142.3972027972028}, {"X"=784.1028169014082, "Y"=142.3972027972028}, {"X"=783.1014084507041, "Y"=142.3972027972028}, {"X"=782.0999999999998, "Y"=142.3972027972028}, {"X"=781.0985915492956, "Y"=142.3972027972028}, {"X"=780.0971830985914, "Y"=142.3972027972028}, {"X"=781.0985915492956, "Y"=141.3944055944056}, {"X"=781.0985915492956, "Y"=140.39160839160843}, {"X"=782.0999999999998, "Y"=139.38881118881125}, {"X"=783.1014084507041, "Y"=138.38601398601406}, {"X"=785.1042253521125, "Y"=136.38041958041958}, {"X"=786.1056338028167, "Y"=134.37482517482522}, {"X"=789.1098591549294, "Y"=131.36643356643356}, {"X"=790.1112676056337, "Y"=130.36363636363637}, {"X"=790.1112676056337, "Y"=129.3608391608392}, {"X"=791.1126760563378, "Y"=127.35524475524483}, {"X"=792.1140845070421, "Y"=126.35244755244753}, {"X"=793.1154929577463, "Y"=125.34965034965035}, {"X"=793.1154929577463, "Y"=124.34685314685316}, {"X"=794.1169014084505, "Y"=123.34405594405598}, {"X"=794.1169014084505, "Y"=122.3412587412588}, {"X"=795.1183098591547, "Y"=121.33846153846162}, {"X"=795.1183098591547, "Y"=120.33566433566432}, {"X"=796.119718309859, "Y"=120.33566433566432}, {"X"=797.1211267605632, "Y"=120.33566433566432}, {"X"=798.1225352112674, "Y"=120.33566433566432}, {"X"=800.1253521126758, "Y"=120.33566433566432}, {"X"=802.1281690140843, "Y"=120.33566433566432}, {"X"=804.1309859154927, "Y"=120.33566433566432}, {"X"=809.1380281690139, "Y"=119.33286713286714}, {"X"=812.1422535211266, "Y"=118.33006993006995}, {"X"=817.1492957746477, "Y"=118.33006993006995}, {"X"=819.1521126760562, "Y"=118.33006993006995}, {"X"=824.1591549295773, "Y"=118.33006993006995}, {"X"=827.1633802816899, "Y"=117.32727272727277}, {"X"=829.1661971830983, "Y"=117.32727272727277}, {"X"=831.1690140845069, "Y"=117.32727272727277}, {"X"=833.1718309859153, "Y"=117.32727272727277}, {"X"=835.1746478873238, "Y"=118.33006993006995}, {"X"=836.1760563380279, "Y"=118.33006993006995}, {"X"=837.1774647887322, "Y"=118.33006993006995}, {"X"=838.1788732394364, "Y"=118.33006993006995}, {"X"=839.1802816901406, "Y"=118.33006993006995}, {"X"=840.1816901408449, "Y"=118.33006993006995}, {"X"=841.1830985915491, "Y"=118.33006993006995}, {"X"=842.1845070422534, "Y"=118.33006993006995}, {"X"=841.1830985915491, "Y"=118.33006993006995}, {"X"=842.1845070422534, "Y"=118.33006993006995}, {"X"=841.1830985915491, "Y"=118.33006993006995}, {"X"=797.1211267605632, "Y"=120.33566433566432}, {"X"=775.0901408450702, "Y"=150.41958041958048}, {"X"=814.145070422535, "Y"=155.4335664335665}, {"X"=826.1619718309857, "Y"=161.45034965034972}, {"X"=832.1704225352111, "Y"=156.4363636363637}, {"X"=835.1746478873238, "Y"=154.43076923076922}, {"X"=836.1760563380279, "Y"=153.42797202797203}, {"X"=836.1760563380279, "Y"=152.42517482517485}, {"X"=837.1774647887322, "Y"=151.42237762237767}, {"X"=839.1802816901406, "Y"=148.413986013986}, {"X"=840.1816901408449, "Y"=146.40839160839164}, {"X"=841.1830985915491, "Y"=144.40279720279727}, {"X"=842.1845070422534, "Y"=143.39999999999998}, {"X"=843.1859154929575, "Y"=140.39160839160843}, {"X"=844.1873239436618, "Y"=140.39160839160843}, {"X"=844.1873239436618, "Y"=139.38881118881125}, {"X"=846.1901408450702, "Y"=136.38041958041958}, {"X"=846.1901408450702, "Y"=135.3776223776224}, {"X"=848.1929577464787, "Y"=133.37202797202804}, {"X"=848.1929577464787, "Y"=131.36643356643356}, {"X"=848.1929577464787, "Y"=130.36363636363637}, {"X"=849.194366197183, "Y"=130.36363636363637}, {"X"=849.194366197183, "Y"=129.3608391608392}, {"X"=849.194366197183, "Y"=128.358041958042}, {"X"=849.194366197183, "Y"=127.35524475524483}, {"X"=850.1957746478871, "Y"=126.35244755244753}, {"X"=850.1957746478871, "Y"=125.34965034965035}, {"X"=850.1957746478871, "Y"=124.34685314685316}, {"X"=850.1957746478871, "Y"=123.34405594405598}, {"X"=851.1971830985914, "Y"=123.34405594405598}, {"X"=852.1985915492955, "Y"=122.3412587412588}, {"X"=853.1999999999998, "Y"=121.33846153846162}, {"X"=854.201408450704, "Y"=121.33846153846162}, {"X"=854.201408450704, "Y"=120.33566433566432}, {"X"=855.2028169014083, "Y"=120.33566433566432}, {"X"=856.2042253521124, "Y"=119.33286713286714}, {"X"=857.2056338028167, "Y"=118.33006993006995}, {"X"=858.207042253521, "Y"=118.33006993006995}, {"X"=859.2084507042251, "Y"=117.32727272727277}, {"X"=860.2098591549294, "Y"=117.32727272727277}, {"X"=862.2126760563378, "Y"=116.32447552447559}, {"X"=864.2154929577463, "Y"=116.32447552447559}, {"X"=864.2154929577463, "Y"=115.3216783216784}, {"X"=866.2183098591547, "Y"=115.3216783216784}, {"X"=867.219718309859, "Y"=115.3216783216784}, {"X"=869.2225352112674, "Y"=115.3216783216784}, {"X"=871.2253521126759, "Y"=114.31888111888111}, {"X"=872.22676056338, "Y"=114.31888111888111}, {"X"=873.2281690140843, "Y"=114.31888111888111}, {"X"=874.2295774647886, "Y"=114.31888111888111}, {"X"=875.2309859154927, "Y"=114.31888111888111}, {"X"=876.232394366197, "Y"=114.31888111888111}, {"X"=877.2338028169012, "Y"=114.31888111888111}, {"X"=878.2352112676055, "Y"=114.31888111888111}, {"X"=878.2352112676055, "Y"=115.3216783216784}, {"X"=879.2366197183096, "Y"=115.3216783216784}, {"X"=880.2380281690139, "Y"=115.3216783216784}, {"X"=881.239436619718, "Y"=115.3216783216784}, {"X"=881.239436619718, "Y"=116.32447552447559}, {"X"=882.2408450704223, "Y"=116.32447552447559}, {"X"=882.2408450704223, "Y"=117.32727272727277}, {"X"=882.2408450704223, "Y"=118.33006993006995}, {"X"=882.2408450704223, "Y"=119.33286713286714}, {"X"=882.2408450704223, "Y"=120.33566433566432}, {"X"=882.2408450704223, "Y"=121.33846153846162}, {"X"=881.239436619718, "Y"=121.33846153846162}, {"X"=881.239436619718, "Y"=122.3412587412588}, {"X"=880.2380281690139, "Y"=123.34405594405598}, {"X"=878.2352112676055, "Y"=125.34965034965035}, {"X"=878.2352112676055, "Y"=126.35244755244753}, {"X"=877.2338028169012, "Y"=127.35524475524483}, {"X"=875.2309859154927, "Y"=128.358041958042}, {"X"=873.2281690140843, "Y"=129.3608391608392}, {"X"=871.2253521126759, "Y"=130.36363636363637}, {"X"=869.2225352112674, "Y"=131.36643356643356}, {"X"=867.219718309859, "Y"=132.36923076923085}, {"X"=865.2169014084506, "Y"=133.37202797202804}, {"X"=863.214084507042, "Y"=134.37482517482522}, {"X"=862.2126760563378, "Y"=135.3776223776224}, {"X"=859.2084507042251, "Y"=136.38041958041958}, {"X"=857.2056338028167, "Y"=137.38321678321677}, {"X"=855.2028169014083, "Y"=139.38881118881125}, {"X"=854.201408450704, "Y"=139.38881118881125}, {"X"=852.1985915492955, "Y"=140.39160839160843}, {"X"=849.194366197183, "Y"=141.3944055944056}, {"X"=849.194366197183, "Y"=142.3972027972028}, {"X"=847.1915492957744, "Y"=142.3972027972028}, {"X"=847.1915492957744, "Y"=143.39999999999998}, {"X"=846.1901408450702, "Y"=143.39999999999998}, {"X"=845.188732394366, "Y"=143.39999999999998}, {"X"=845.188732394366, "Y"=144.40279720279727}, {"X"=844.1873239436618, "Y"=144.40279720279727}, {"X"=844.1873239436618, "Y"=145.40559440559446}, {"X"=843.1859154929575, "Y"=145.40559440559446}, {"X"=844.1873239436618, "Y"=145.40559440559446}, {"X"=844.1873239436618, "Y"=146.40839160839164}, {"X"=845.188732394366, "Y"=146.40839160839164}, {"X"=848.1929577464787, "Y"=147.41118881118882}, {"X"=850.1957746478871, "Y"=148.413986013986}, {"X"=853.1999999999998, "Y"=149.4167832167833}, {"X"=855.2028169014083, "Y"=150.41958041958048}, {"X"=856.2042253521124, "Y"=151.42237762237767}, {"X"=859.2084507042251, "Y"=152.42517482517485}, {"X"=862.2126760563378, "Y"=153.42797202797203}, {"X"=865.2169014084506, "Y"=154.43076923076922}, {"X"=868.2211267605632, "Y"=156.4363636363637}, {"X"=869.2225352112674, "Y"=157.43916083916088}, {"X"=872.22676056338, "Y"=159.44475524475524}, {"X"=874.2295774647886, "Y"=160.44755244755243}, {"X"=875.2309859154927, "Y"=161.45034965034972}, {"X"=876.232394366197, "Y"=162.4531468531469}, {"X"=877.2338028169012, "Y"=163.4559440559441}, {"X"=878.2352112676055, "Y"=164.45874125874127}, {"X"=879.2366197183096, "Y"=164.45874125874127}, {"X"=880.2380281690139, "Y"=165.46153846153845}, {"X"=881.239436619718, "Y"=165.46153846153845}, {"X"=881.239436619718, "Y"=166.46433566433564}, {"X"=881.239436619718, "Y"=167.46713286713293}, {"X"=882.2408450704223, "Y"=167.46713286713293}, {"X"=883.2422535211266, "Y"=167.46713286713293}, {"X"=883.2422535211266, "Y"=168.46993006993011}, {"X"=884.2436619718308, "Y"=168.46993006993011}, {"X"=883.2422535211266, "Y"=168.46993006993011}, {"X"=892.2549295774646, "Y"=165.46153846153845}, {"X"=896.2605633802815, "Y"=168.46993006993011}, {"X"=900.2661971830984, "Y"=167.46713286713293}, {"X"=902.2690140845068, "Y"=167.46713286713293}, {"X"=906.2746478873237, "Y"=166.46433566433564}, {"X"=911.2816901408448, "Y"=165.46153846153845}, {"X"=920.2943661971829, "Y"=163.4559440559441}, {"X"=925.301408450704, "Y"=162.4531468531469}, {"X"=937.3183098591547, "Y"=159.44475524475524}, {"X"=945.3295774647885, "Y"=157.43916083916088}, {"X"=952.3394366197182, "Y"=156.4363636363637}, {"X"=963.3549295774645, "Y"=156.4363636363637}, {"X"=970.3647887323942, "Y"=158.44195804195806}, {"X"=977.3746478873237, "Y"=162.4531468531469}, {"X"=982.3816901408449, "Y"=166.46433566433564}, {"X"=984.3845070422532, "Y"=169.4727272727273}, {"X"=987.388732394366, "Y"=174.48671328671333}, {"X"=989.3915492957743, "Y"=181.50629370629372}, {"X"=988.3901408450703, "Y"=187.52307692307693}, {"X"=986.3873239436617, "Y"=192.53706293706296}, {"X"=983.3830985915491, "Y"=197.55104895104898}, {"X"=978.376056338028, "Y"=202.565034965035}, {"X"=975.3718309859152, "Y"=205.57342657342662}, {"X"=972.3676056338026, "Y"=207.57902097902098}, {"X"=968.3619718309857, "Y"=210.5874125874126}, {"X"=962.3535211267603, "Y"=212.593006993007}, {"X"=959.3492957746477, "Y"=213.59580419580425}, {"X"=956.3450704225351, "Y"=213.59580419580425}, {"X"=951.3380281690139, "Y"=214.59860139860143}, {"X"=948.3338028169012, "Y"=214.59860139860143}, {"X"=945.3295774647885, "Y"=214.59860139860143}, {"X"=937.3183098591547, "Y"=214.59860139860143}, {"X"=933.3126760563379, "Y"=214.59860139860143}, {"X"=928.3056338028167, "Y"=213.59580419580425}, {"X"=922.2971830985913, "Y"=213.59580419580425}, {"X"=914.2859154929575, "Y"=212.593006993007}, {"X"=908.2774647887322, "Y"=212.593006993007}, {"X"=902.2690140845068, "Y"=212.593006993007}, {"X"=893.2563380281688, "Y"=212.593006993007}, {"X"=888.2492957746476, "Y"=212.593006993007}, {"X"=880.2380281690139, "Y"=211.59020979020983}, {"X"=870.2239436619716, "Y"=210.5874125874126}, {"X"=863.214084507042, "Y"=208.58181818181822}, {"X"=857.2056338028167, "Y"=207.57902097902098}, {"X"=852.1985915492955, "Y"=206.5762237762238}, {"X"=840.1816901408449, "Y"=204.57062937062938}, {"X"=832.1704225352111, "Y"=203.5678321678322}, {"X"=826.1619718309857, "Y"=202.565034965035}, {"X"=817.1492957746477, "Y"=202.565034965035}, {"X"=806.1338028169013, "Y"=200.55944055944053}, {"X"=797.1211267605632, "Y"=199.55664335664335}, {"X"=786.1056338028167, "Y"=198.55384615384617}, {"X"=770.0830985915491, "Y"=197.55104895104898}, {"X"=757.0647887323942, "Y"=197.55104895104898}, {"X"=742.0436619718308, "Y"=196.5482517482518}, {"X"=728.0239436619717, "Y"=195.54545454545462}, {"X"=707.9957746478872, "Y"=195.54545454545462}, {"X"=692.9746478873237, "Y"=195.54545454545462}, {"X"=681.9591549295773, "Y"=195.54545454545462}, {"X"=666.9380281690139, "Y"=196.5482517482518}, {"X"=651.9169014084506, "Y"=196.5482517482518}, {"X"=630.8873239436618, "Y"=196.5482517482518}, {"X"=616.8676056338027, "Y"=197.55104895104898}, {"X"=599.8436619718308, "Y"=198.55384615384617}, {"X"=583.8211267605633, "Y"=200.55944055944053}, {"X"=562.7915492957745, "Y"=202.565034965035}, {"X"=547.7704225352111, "Y"=204.57062937062938}, {"X"=532.7492957746477, "Y"=207.57902097902098}, {"X"=524.738028169014, "Y"=208.58181818181822}, {"X"=503.70845070422524, "Y"=212.593006993007}, {"X"=495.6971830985914, "Y"=213.59580419580425}, {"X"=483.68028169014076, "Y"=214.59860139860143}, {"X"=473.66619718309846, "Y"=215.6013986013986}, {"X"=459.6464788732393, "Y"=216.60419580419585}, {"X"=447.62957746478867, "Y"=217.60699300699304}, {"X"=436.61408450704215, "Y"=218.60979020979022}, {"X"=426.5999999999999, "Y"=219.61258741258746}, {"X"=413.58169014084496, "Y"=220.61538461538464}, {"X"=403.5676056338027, "Y"=220.61538461538464}, {"X"=392.55211267605625, "Y"=221.61818181818182}, {"X"=385.54225352112667, "Y"=221.61818181818182}, {"X"=369.51971830985906, "Y"=220.61538461538464}, {"X"=358.5042253521126, "Y"=220.61538461538464}, {"X"=350.4929577464788, "Y"=220.61538461538464}, {"X"=339.47746478873233, "Y"=219.61258741258746}, {"X"=328.4619718309858, "Y"=218.60979020979022}, {"X"=313.4408450704224, "Y"=217.60699300699304}, {"X"=302.42535211267597, "Y"=215.6013986013986}, {"X"=290.4084507042253, "Y"=215.6013986013986}, {"X"=278.39154929577455, "Y"=215.6013986013986}, {"X"=265.37323943661966, "Y"=215.6013986013986}, {"X"=252.3549295774647, "Y"=216.60419580419585}, {"X"=241.33943661971824, "Y"=217.60699300699304}, {"X"=231.325352112676, "Y"=218.60979020979022}, {"X"=214.30140845070417, "Y"=219.61258741258746}, {"X"=204.28732394366193, "Y"=220.61538461538464}, {"X"=194.2732394366197, "Y"=221.61818181818182}, {"X"=185.2605633802816, "Y"=222.62097902097906}, {"X"=179.2521126760563, "Y"=223.62377622377625}, {"X"=169.23802816901403, "Y"=225.62937062937067}, {"X"=158.22253521126757, "Y"=227.63496503496503}, {"X"=147.20704225352108, "Y"=229.64055944055946}, {"X"=129.18169014084503, "Y"=233.6517482517483}, {"X"=118.16619718309855, "Y"=235.65734265734267}, {"X"=104.1464788732394, "Y"=237.6629370629371}, {"X"=92.1295774647887, "Y"=240.6713286713287}, {"X"=80.11267605633799, "Y"=242.67692307692312}, {"X"=68.09577464788731, "Y"=244.68251748251748}, {"X"=55.07746478873236, "Y"=247.6909090909091}, {"X"=43.060563380281664, "Y"=249.6965034965035}, {"X"=31.04366197183097, "Y"=253.70769230769235}, {"X"=13.018309859154911, "Y"=259.72447552447557}, {"X"=1.0014084507042185, "Y"=263.73566433566435}, {"X"=-10.01408450704227, "Y"=268.7496503496504}, {"X"=-20.02816901408451, "Y"=273.7636363636364}, {"X"=-31.043661971830993, "Y"=279.7804195804196}, {"X"=-40.056338028169016, "Y"=284.7944055944056}, {"X"=-47.066197183098595, "Y"=289.8083916083916}, {"X"=-53.07464788732395, "Y"=295.8251748251748}, {"X"=-59.083098591549295, "Y"=300.83916083916085}, {"X"=-66.09295774647887, "Y"=309.86433566433567}, {"X"=-71.1, "Y"=317.8867132867133}, {"X"=-77.10845070422535, "Y"=328.91748251748254}, {"X"=-83.1169014084507, "Y"=337.94265734265736}, {"X"=-89.12535211267604, "Y"=348.9734265734266}, {"X"=-92.12957746478872, "Y"=357.9986013986014}, {"X"=-93.13098591549294, "Y"=367.0237762237762}, {"X"=-93.13098591549294, "Y"=372.03776223776225}, {"X"=-92.12957746478872, "Y"=376.04895104895104}, {"X"=-90.12676056338027, "Y"=385.0741258741259}, {"X"=-86.12112676056337, "Y"=394.0993006993007}, {"X"=-84.11830985915492, "Y"=397.10769230769233}, {"X"=-82.11549295774647, "Y"=400.11608391608394}, {"X"=-79.1112676056338, "Y"=402.12167832167836}, {"X"=-74.10422535211268, "Y"=405.13006993006996}, {"X"=-69.09718309859154, "Y"=406.13286713286715}, {"X"=-64.09014084507042, "Y"=408.13846153846157}, {"X"=-58.08169014084507, "Y"=410.14405594405594}, {"X"=-54.07605633802817, "Y"=410.14405594405594}, {"X"=-51.0718309859155, "Y"=409.14125874125875}, {"X"=-46.06478873239437, "Y"=407.13566433566433}, {"X"=-39.05492957746479, "Y"=403.12447552447554}, {"X"=-34.04788732394367, "Y"=399.11328671328675}, {"X"=-29.04084507042254, "Y"=395.1020979020979}, {"X"=-23.032394366197188, "Y"=391.0909090909091}, {"X"=-19.026760563380293, "Y"=387.0797202797203}, {"X"=-16.022535211267616, "Y"=385.0741258741259}, {"X"=-13.01830985915494, "Y"=383.0685314685315}, {"X"=-11.015492957746488, "Y"=381.06293706293707}, {"X"=-6.008450704225368, "Y"=377.0517482517483}, {"X"=-4.0056338028169165, "Y"=374.0433566433567}, {"X"=-1.4210854715202004e-14, "Y"=372.03776223776225}, {"X"=2.002816901408437, "Y"=370.03216783216783}, {"X"=6.008450704225339, "Y"=367.0237762237762}, {"X"=8.01126760563379, "Y"=366.02097902097904}, {"X"=10.014084507042242, "Y"=365.01818181818186}, {"X"=13.018309859154911, "Y"=364.0153846153846}, {"X"=15.021126760563362, "Y"=364.0153846153846}, {"X"=17.023943661971813, "Y"=364.0153846153846}, {"X"=18.025352112676046, "Y"=364.0153846153846}, {"X"=20.028169014084497, "Y"=364.0153846153846}, {"X"=21.029577464788716, "Y"=364.0153846153846}, {"X"=22.030985915492934, "Y"=365.01818181818186}, {"X"=22.030985915492934, "Y"=366.02097902097904}, {"X"=22.030985915492934, "Y"=365.01818181818186}, {"X"=21.029577464788716, "Y"=364.0153846153846}, {"X"=16.022535211267595, "Y"=368.02657342657346}, {"X"=20.028169014084497, "Y"=369.02937062937065}, {"X"=21.029577464788716, "Y"=369.02937062937065}, {"X"=23.032394366197167, "Y"=368.02657342657346}, {"X"=23.032394366197167, "Y"=367.0237762237762}, {"X"=24.033802816901385, "Y"=366.02097902097904}, {"X"=26.036619718309836, "Y"=364.0153846153846}, {"X"=28.039436619718288, "Y"=362.00979020979025}, {"X"=30.04225352112674, "Y"=360.00419580419583}, {"X"=31.04366197183097, "Y"=359.0013986013986}, {"X"=34.04788732394364, "Y"=355.993006993007}, {"X"=35.049295774647874, "Y"=353.9874125874126}, {"X"=37.05211267605631, "Y"=352.9846153846154}, {"X"=38.05352112676054, "Y"=350.979020979021}, {"X"=40.056338028168994, "Y"=349.9762237762238}, {"X"=41.05774647887321, "Y"=348.9734265734266}, {"X"=44.0619718309859, "Y"=345.965034965035}, {"X"=46.06478873239435, "Y"=344.9622377622378}, {"X"=47.066197183098566, "Y"=342.9566433566434}, {"X"=49.06901408450702, "Y"=340.95104895104896}, {"X"=51.07183098591547, "Y"=339.9482517482518}, {"X"=53.07464788732392, "Y"=337.94265734265736}, {"X"=55.07746478873236, "Y"=336.9398601398602}, {"X"=59.08309859154926, "Y"=333.93146853146857}, {"X"=61.085915492957724, "Y"=331.92587412587415}, {"X"=62.08732394366194, "Y"=329.9202797202797}, {"X"=64.09014084507041, "Y"=328.91748251748254}, {"X"=66.09295774647885, "Y"=326.9118881118881}, {"X"=68.09577464788731, "Y"=323.9034965034965}, {"X"=69.09718309859153, "Y"=322.90069930069933}, {"X"=70.09859154929575, "Y"=320.8951048951049}, {"X"=73.10281690140843, "Y"=316.8839160839161}, {"X"=74.10422535211265, "Y"=314.8783216783217}, {"X"=75.10563380281687, "Y"=311.8699300699301}, {"X"=76.10704225352109, "Y"=308.8615384615385}, {"X"=77.10845070422533, "Y"=306.85594405594406}, {"X"=78.10985915492955, "Y"=304.8503496503497}, {"X"=79.11126760563377, "Y"=303.84755244755246}, {"X"=79.11126760563377, "Y"=302.8447552447553}, {"X"=79.11126760563377, "Y"=301.84195804195804}, {"X"=80.11267605633799, "Y"=300.83916083916085}, {"X"=80.11267605633799, "Y"=299.83636363636367}, {"X"=81.11408450704224, "Y"=298.83356643356643}, {"X"=81.11408450704224, "Y"=297.83076923076925}, {"X"=82.11549295774645, "Y"=295.8251748251748}, {"X"=83.11690140845067, "Y"=294.82237762237764}, {"X"=83.11690140845067, "Y"=293.81958041958046}, {"X"=83.11690140845067, "Y"=292.8167832167832}, {"X"=84.11830985915489, "Y"=292.8167832167832}, {"X"=84.11830985915489, "Y"=291.81398601398604}, {"X"=84.11830985915489, "Y"=290.81118881118886}, {"X"=85.11971830985914, "Y"=289.8083916083916}, {"X"=85.11971830985914, "Y"=288.80559440559443}, {"X"=85.11971830985914, "Y"=289.8083916083916}, {"X"=85.11971830985914, "Y"=290.81118881118886}, {"X"=85.11971830985914, "Y"=291.81398601398604}, {"X"=85.11971830985914, "Y"=293.81958041958046}, {"X"=85.11971830985914, "Y"=294.82237762237764}, {"X"=85.11971830985914, "Y"=295.8251748251748}, {"X"=85.11971830985914, "Y"=297.83076923076925}, {"X"=85.11971830985914, "Y"=299.83636363636367}, {"X"=84.11830985915489, "Y"=301.84195804195804}, {"X"=84.11830985915489, "Y"=303.84755244755246}, {"X"=84.11830985915489, "Y"=306.85594405594406}, {"X"=84.11830985915489, "Y"=309.86433566433567}, {"X"=83.11690140845067, "Y"=313.8755244755245}, {"X"=83.11690140845067, "Y"=316.8839160839161}, {"X"=81.11408450704224, "Y"=322.90069930069933}, {"X"=80.11267605633799, "Y"=326.9118881118881}, {"X"=80.11267605633799, "Y"=327.91468531468536}, {"X"=78.10985915492955, "Y"=333.93146853146857}, {"X"=77.10845070422533, "Y"=337.94265734265736}, {"X"=76.10704225352109, "Y"=340.95104895104896}, {"X"=75.10563380281687, "Y"=342.9566433566434}, {"X"=74.10422535211265, "Y"=345.965034965035}, {"X"=74.10422535211265, "Y"=347.9706293706294}, {"X"=73.10281690140843, "Y"=349.9762237762238}, {"X"=72.10140845070418, "Y"=352.9846153846154}, {"X"=71.09999999999997, "Y"=356.9958041958042}, {"X"=70.09859154929575, "Y"=357.9986013986014}, {"X"=69.09718309859153, "Y"=361.006993006993}, {"X"=68.09577464788731, "Y"=363.01258741258744}, {"X"=68.09577464788731, "Y"=365.01818181818186}, {"X"=67.09436619718306, "Y"=367.0237762237762}, {"X"=67.09436619718306, "Y"=368.02657342657346}, {"X"=67.09436619718306, "Y"=369.02937062937065}, {"X"=66.09295774647885, "Y"=369.02937062937065}, {"X"=66.09295774647885, "Y"=370.03216783216783}, {"X"=66.09295774647885, "Y"=371.03496503496507}, {"X"=66.09295774647885, "Y"=372.03776223776225}, {"X"=65.09154929577463, "Y"=372.03776223776225}, {"X"=65.09154929577463, "Y"=373.04055944055943}, {"X"=65.09154929577463, "Y"=374.0433566433567}, {"X"=64.09014084507041, "Y"=374.0433566433567}, {"X"=64.09014084507041, "Y"=375.04615384615386}, {"X"=64.09014084507041, "Y"=376.04895104895104}, {"X"=63.08873239436616, "Y"=376.04895104895104}, {"X"=63.08873239436616, "Y"=375.04615384615386}, {"X"=64.09014084507041, "Y"=375.04615384615386}, {"X"=63.08873239436616, "Y"=375.04615384615386}, {"X"=63.08873239436616, "Y"=374.0433566433567}, {"X"=63.08873239436616, "Y"=373.04055944055943}, {"X"=64.09014084507041, "Y"=373.04055944055943}, {"X"=64.09014084507041, "Y"=372.03776223776225}, {"X"=65.09154929577463, "Y"=370.03216783216783}, {"X"=65.09154929577463, "Y"=368.02657342657346}, {"X"=66.09295774647885, "Y"=367.0237762237762}, {"X"=67.09436619718306, "Y"=364.0153846153846}, {"X"=69.09718309859153, "Y"=359.0013986013986}, {"X"=70.09859154929575, "Y"=356.9958041958042}, {"X"=72.10140845070418, "Y"=351.9818181818182}, {"X"=73.10281690140843, "Y"=348.9734265734266}, {"X"=74.10422535211265, "Y"=346.96783216783217}, {"X"=74.10422535211265, "Y"=345.965034965035}, {"X"=75.10563380281687, "Y"=344.9622377622378}, {"X"=75.10563380281687, "Y"=343.95944055944057}, {"X"=75.10563380281687, "Y"=342.9566433566434}, {"X"=75.10563380281687, "Y"=341.9538461538462}, {"X"=75.10563380281687, "Y"=340.95104895104896}, {"X"=75.10563380281687, "Y"=339.9482517482518}, {"X"=75.10563380281687, "Y"=340.95104895104896}, {"X"=74.10422535211265, "Y"=340.95104895104896}, {"X"=73.10281690140843, "Y"=340.95104895104896}, {"X"=73.10281690140843, "Y"=341.9538461538462}, {"X"=72.10140845070418, "Y"=341.9538461538462}, {"X"=71.09999999999997, "Y"=341.9538461538462}, {"X"=71.09999999999997, "Y"=342.9566433566434}, {"X"=70.09859154929575, "Y"=342.9566433566434}, {"X"=68.09577464788731, "Y"=343.95944055944057}, {"X"=64.09014084507041, "Y"=344.9622377622378}, {"X"=63.08873239436616, "Y"=344.9622377622378}, {"X"=60.084507042253506, "Y"=345.965034965035}, {"X"=57.08028169014082, "Y"=346.96783216783217}, {"X"=55.07746478873236, "Y"=346.96783216783217}, {"X"=51.07183098591547, "Y"=346.96783216783217}, {"X"=48.0676056338028, "Y"=346.96783216783217}, {"X"=47.066197183098566, "Y"=346.96783216783217}, {"X"=45.063380281690115, "Y"=346.96783216783217}, {"X"=44.0619718309859, "Y"=346.96783216783217}, {"X"=43.060563380281664, "Y"=346.96783216783217}, {"X"=42.059154929577446, "Y"=346.96783216783217}, {"X"=41.05774647887321, "Y"=346.96783216783217}, {"X"=43.060563380281664, "Y"=346.96783216783217}, {"X"=45.063380281690115, "Y"=347.9706293706294}, {"X"=47.066197183098566, "Y"=347.9706293706294}, {"X"=52.0732394366197, "Y"=347.9706293706294}, {"X"=53.07464788732392, "Y"=347.9706293706294}, {"X"=58.08169014084504, "Y"=346.96783216783217}, {"X"=59.08309859154926, "Y"=345.965034965035}, {"X"=62.08732394366194, "Y"=344.9622377622378}, {"X"=65.09154929577463, "Y"=343.95944055944057}, {"X"=67.09436619718306, "Y"=343.95944055944057}, {"X"=67.09436619718306, "Y"=342.9566433566434}, {"X"=69.09718309859153, "Y"=342.9566433566434}, {"X"=70.09859154929575, "Y"=341.9538461538462}, {"X"=71.09999999999997, "Y"=341.9538461538462}, {"X"=72.10140845070418, "Y"=340.95104895104896}, {"X"=73.10281690140843, "Y"=340.95104895104896}, {"X"=74.10422535211265, "Y"=340.95104895104896}, {"X"=74.10422535211265, "Y"=339.9482517482518}, {"X"=75.10563380281687, "Y"=339.9482517482518}, {"X"=76.10704225352109, "Y"=339.9482517482518}, {"X"=77.10845070422533, "Y"=339.9482517482518}, {"X"=77.10845070422533, "Y"=338.94545454545454}, {"X"=78.10985915492955, "Y"=338.94545454545454}, {"X"=77.10845070422533, "Y"=338.94545454545454}, {"X"=76.10704225352109, "Y"=338.94545454545454}, {"X"=116.16338028169011, "Y"=307.8587412587413}, {"X"=115.16197183098589, "Y"=307.8587412587413}, {"X"=112.15774647887321, "Y"=316.8839160839161}, {"X"=111.15633802816899, "Y"=317.8867132867133}, {"X"=110.15492957746474, "Y"=319.8923076923077}, {"X"=110.15492957746474, "Y"=322.90069930069933}, {"X"=109.15352112676052, "Y"=324.90629370629375}, {"X"=108.1521126760563, "Y"=325.90909090909093}, {"X"=107.15070422535209, "Y"=329.9202797202797}, {"X"=105.14788732394362, "Y"=334.93426573426575}, {"X"=104.1464788732394, "Y"=337.94265734265736}, {"X"=102.14366197183094, "Y"=340.95104895104896}, {"X"=101.14225352112672, "Y"=343.95944055944057}, {"X"=99.13943661971828, "Y"=346.96783216783217}, {"X"=97.13661971830982, "Y"=349.9762237762238}, {"X"=97.13661971830982, "Y"=350.979020979021}, {"X"=96.1352112676056, "Y"=352.9846153846154}, {"X"=95.13380281690138, "Y"=353.9874125874126}, {"X"=94.13239436619716, "Y"=355.993006993007}, {"X"=94.13239436619716, "Y"=356.9958041958042}, {"X"=93.13098591549291, "Y"=357.9986013986014}, {"X"=93.13098591549291, "Y"=360.00419580419583}, {"X"=92.1295774647887, "Y"=362.00979020979025}, {"X"=92.1295774647887, "Y"=363.01258741258744}, {"X"=91.12816901408448, "Y"=364.0153846153846}, {"X"=91.12816901408448, "Y"=365.01818181818186}, {"X"=91.12816901408448, "Y"=366.02097902097904}, {"X"=90.12676056338026, "Y"=366.02097902097904}, {"X"=90.12676056338026, "Y"=367.0237762237762}, {"X"=91.12816901408448, "Y"=367.0237762237762}, {"X"=91.12816901408448, "Y"=366.02097902097904}, {"X"=91.12816901408448, "Y"=365.01818181818186}, {"X"=92.1295774647887, "Y"=364.0153846153846}, {"X"=93.13098591549291, "Y"=362.00979020979025}, {"X"=93.13098591549291, "Y"=361.006993006993}, {"X"=95.13380281690138, "Y"=356.9958041958042}, {"X"=100.1408450704225, "Y"=351.9818181818182}, {"X"=102.14366197183094, "Y"=347.9706293706294}, {"X"=105.14788732394362, "Y"=344.9622377622378}, {"X"=109.15352112676052, "Y"=340.95104895104896}, {"X"=111.15633802816899, "Y"=337.94265734265736}, {"X"=114.16056338028164, "Y"=334.93426573426575}, {"X"=116.16338028169011, "Y"=332.9286713286713}, {"X"=119.16760563380276, "Y"=329.9202797202797}, {"X"=121.17042253521123, "Y"=326.9118881118881}, {"X"=123.17323943661967, "Y"=322.90069930069933}, {"X"=125.17605633802813, "Y"=319.8923076923077}, {"X"=126.17746478873235, "Y"=317.8867132867133}, {"X"=127.17887323943657, "Y"=315.8811188811189}, {"X"=129.18169014084503, "Y"=312.8727272727273}, {"X"=130.18309859154925, "Y"=309.86433566433567}, {"X"=132.18591549295772, "Y"=306.85594405594406}, {"X"=133.18732394366194, "Y"=305.8531468531469}, {"X"=134.18873239436616, "Y"=304.8503496503497}, {"X"=134.18873239436616, "Y"=303.84755244755246}, {"X"=135.19014084507037, "Y"=302.8447552447553}, {"X"=136.1915492957746, "Y"=301.84195804195804}, {"X"=137.19295774647884, "Y"=300.83916083916085}, {"X"=138.19436619718306, "Y"=300.83916083916085}, {"X"=138.19436619718306, "Y"=299.83636363636367}, {"X"=139.19577464788728, "Y"=299.83636363636367}, {"X"=140.1971830985915, "Y"=299.83636363636367}, {"X"=140.1971830985915, "Y"=300.83916083916085}, {"X"=141.19859154929574, "Y"=300.83916083916085}, {"X"=141.19859154929574, "Y"=301.84195804195804}, {"X"=140.1971830985915, "Y"=303.84755244755246}, {"X"=140.1971830985915, "Y"=306.85594405594406}, {"X"=139.19577464788728, "Y"=310.8671328671329}, {"X"=138.19436619718306, "Y"=313.8755244755245}, {"X"=138.19436619718306, "Y"=318.8895104895105}, {"X"=137.19295774647884, "Y"=322.90069930069933}, {"X"=136.1915492957746, "Y"=326.9118881118881}, {"X"=134.18873239436616, "Y"=330.92307692307696}, {"X"=133.18732394366194, "Y"=333.93146853146857}, {"X"=132.18591549295772, "Y"=336.9398601398602}, {"X"=131.18450704225347, "Y"=339.9482517482518}, {"X"=130.18309859154925, "Y"=340.95104895104896}, {"X"=128.18028169014082, "Y"=344.9622377622378}, {"X"=127.17887323943657, "Y"=346.96783216783217}, {"X"=126.17746478873235, "Y"=348.9734265734266}, {"X"=124.17464788732391, "Y"=350.979020979021}, {"X"=123.17323943661967, "Y"=353.9874125874126}, {"X"=122.17183098591545, "Y"=355.993006993007}, {"X"=121.17042253521123, "Y"=355.993006993007}, {"X"=121.17042253521123, "Y"=357.9986013986014}, {"X"=120.16901408450701, "Y"=360.00419580419583}, {"X"=120.16901408450701, "Y"=361.006993006993}, {"X"=119.16760563380276, "Y"=362.00979020979025}, {"X"=119.16760563380276, "Y"=363.01258741258744}, {"X"=119.16760563380276, "Y"=364.0153846153846}, {"X"=118.16619718309855, "Y"=365.01818181818186}, {"X"=118.16619718309855, "Y"=366.02097902097904}, {"X"=118.16619718309855, "Y"=367.0237762237762}, {"X"=118.16619718309855, "Y"=366.02097902097904}, {"X"=119.16760563380276, "Y"=366.02097902097904}, {"X"=119.16760563380276, "Y"=365.01818181818186}, {"X"=120.16901408450701, "Y"=363.01258741258744}, {"X"=123.17323943661967, "Y"=356.9958041958042}, {"X"=126.17746478873235, "Y"=352.9846153846154}, {"X"=129.18169014084503, "Y"=347.9706293706294}, {"X"=132.18591549295772, "Y"=343.95944055944057}, {"X"=136.1915492957746, "Y"=337.94265734265736}, {"X"=139.19577464788728, "Y"=333.93146853146857}, {"X"=142.19999999999996, "Y"=329.9202797202797}, {"X"=146.20563380281686, "Y"=325.90909090909093}, {"X"=148.2084507042253, "Y"=323.9034965034965}, {"X"=150.21126760563376, "Y"=319.8923076923077}, {"X"=153.21549295774642, "Y"=316.8839160839161}, {"X"=155.21830985915489, "Y"=313.8755244755245}, {"X"=156.2197183098591, "Y"=312.8727272727273}, {"X"=157.22112676056332, "Y"=310.8671328671329}, {"X"=158.22253521126757, "Y"=309.86433566433567}, {"X"=159.2239436619718, "Y"=308.8615384615385}, {"X"=160.225352112676, "Y"=308.8615384615385}, {"X"=160.225352112676, "Y"=307.8587412587413}, {"X"=161.22676056338022, "Y"=307.8587412587413}, {"X"=163.2295774647887, "Y"=307.8587412587413}, {"X"=163.2295774647887, "Y"=308.8615384615385}, {"X"=163.2295774647887, "Y"=309.86433566433567}, {"X"=164.2309859154929, "Y"=309.86433566433567}, {"X"=164.2309859154929, "Y"=311.8699300699301}, {"X"=164.2309859154929, "Y"=314.8783216783217}, {"X"=164.2309859154929, "Y"=316.8839160839161}, {"X"=164.2309859154929, "Y"=319.8923076923077}, {"X"=164.2309859154929, "Y"=321.8979020979021}, {"X"=163.2295774647887, "Y"=324.90629370629375}, {"X"=162.22816901408447, "Y"=327.91468531468536}, {"X"=161.22676056338022, "Y"=332.9286713286713}, {"X"=160.225352112676, "Y"=335.93706293706293}, {"X"=158.22253521126757, "Y"=338.94545454545454}, {"X"=157.22112676056332, "Y"=342.9566433566434}, {"X"=155.21830985915489, "Y"=345.965034965035}, {"X"=153.21549295774642, "Y"=348.9734265734266}, {"X"=151.21267605633798, "Y"=351.9818181818182}, {"X"=150.21126760563376, "Y"=354.9902097902098}, {"X"=149.20985915492952, "Y"=357.9986013986014}, {"X"=148.2084507042253, "Y"=361.006993006993}, {"X"=147.20704225352108, "Y"=361.006993006993}, {"X"=146.20563380281686, "Y"=363.01258741258744}, {"X"=146.20563380281686, "Y"=364.0153846153846}, {"X"=145.20422535211264, "Y"=366.02097902097904}, {"X"=144.2028169014084, "Y"=367.0237762237762}, {"X"=144.2028169014084, "Y"=368.02657342657346}, {"X"=144.2028169014084, "Y"=369.02937062937065}, {"X"=144.2028169014084, "Y"=370.03216783216783}, {"X"=143.20140845070418, "Y"=371.03496503496507}, {"X"=143.20140845070418, "Y"=372.03776223776225}, {"X"=142.19999999999996, "Y"=372.03776223776225}, {"X"=142.19999999999996, "Y"=373.04055944055943}, {"X"=142.19999999999996, "Y"=372.03776223776225}, {"X"=142.19999999999996, "Y"=371.03496503496507}, {"X"=174.24507042253515, "Y"=364.0153846153846}, {"X"=172.2422535211267, "Y"=369.02937062937065}, {"X"=177.24929577464783, "Y"=361.006993006993}, {"X"=178.25070422535205, "Y"=357.9986013986014}, {"X"=178.25070422535205, "Y"=356.9958041958042}, {"X"=179.2521126760563, "Y"=354.9902097902098}, {"X"=179.2521126760563, "Y"=353.9874125874126}, {"X"=180.25352112676052, "Y"=351.9818181818182}, {"X"=181.25492957746474, "Y"=348.9734265734266}, {"X"=182.25633802816895, "Y"=344.9622377622378}, {"X"=183.25774647887317, "Y"=341.9538461538462}, {"X"=184.2591549295774, "Y"=338.94545454545454}, {"X"=185.2605633802816, "Y"=336.9398601398602}, {"X"=185.2605633802816, "Y"=332.9286713286713}, {"X"=187.2633802816901, "Y"=327.91468531468536}, {"X"=188.26478873239432, "Y"=324.90629370629375}, {"X"=188.26478873239432, "Y"=321.8979020979021}, {"X"=189.26619718309854, "Y"=318.8895104895105}, {"X"=189.26619718309854, "Y"=317.8867132867133}, {"X"=189.26619718309854, "Y"=316.8839160839161}, {"X"=189.26619718309854, "Y"=315.8811188811189}, {"X"=189.26619718309854, "Y"=314.8783216783217}, {"X"=189.26619718309854, "Y"=313.8755244755245}, {"X"=189.26619718309854, "Y"=312.8727272727273}, {"X"=189.26619718309854, "Y"=311.8699300699301}, {"X"=189.26619718309854, "Y"=312.8727272727273}, {"X"=188.26478873239432, "Y"=312.8727272727273}, {"X"=188.26478873239432, "Y"=313.8755244755245}, {"X"=179.2521126760563, "Y"=308.8615384615385}, {"X"=182.25633802816895, "Y"=309.86433566433567}, {"X"=184.2591549295774, "Y"=307.8587412587413}, {"X"=185.2605633802816, "Y"=306.85594405594406}, {"X"=186.26197183098589, "Y"=306.85594405594406}, {"X"=187.2633802816901, "Y"=305.8531468531469}, {"X"=188.26478873239432, "Y"=305.8531468531469}, {"X"=190.26760563380276, "Y"=303.84755244755246}, {"X"=194.2732394366197, "Y"=302.8447552447553}, {"X"=195.2746478873239, "Y"=302.8447552447553}, {"X"=199.28028169014078, "Y"=301.84195804195804}, {"X"=202.28450704225344, "Y"=301.84195804195804}, {"X"=205.28873239436615, "Y"=300.83916083916085}, {"X"=207.2915492957746, "Y"=300.83916083916085}, {"X"=208.2929577464788, "Y"=299.83636363636367}, {"X"=209.29436619718302, "Y"=299.83636363636367}, {"X"=210.29577464788724, "Y"=299.83636363636367}, {"X"=211.29718309859152, "Y"=299.83636363636367}, {"X"=212.29859154929574, "Y"=299.83636363636367}, {"X"=213.29999999999995, "Y"=299.83636363636367}, {"X"=213.29999999999995, "Y"=300.83916083916085}, {"X"=214.30140845070417, "Y"=300.83916083916085}, {"X"=214.30140845070417, "Y"=301.84195804195804}, {"X"=214.30140845070417, "Y"=302.8447552447553}, {"X"=214.30140845070417, "Y"=303.84755244755246}, {"X"=213.29999999999995, "Y"=303.84755244755246}, {"X"=212.29859154929574, "Y"=305.8531468531469}, {"X"=211.29718309859152, "Y"=307.8587412587413}, {"X"=209.29436619718302, "Y"=309.86433566433567}, {"X"=208.2929577464788, "Y"=311.8699300699301}, {"X"=207.2915492957746, "Y"=313.8755244755245}, {"X"=205.28873239436615, "Y"=315.8811188811189}, {"X"=201.28309859154922, "Y"=319.8923076923077}, {"X"=199.28028169014078, "Y"=321.8979020979021}, {"X"=196.27605633802813, "Y"=323.9034965034965}, {"X"=193.27183098591541, "Y"=325.90909090909093}, {"X"=192.2704225352112, "Y"=326.9118881118881}, {"X"=191.26901408450698, "Y"=327.91468531468536}, {"X"=190.26760563380276, "Y"=327.91468531468536}, {"X"=190.26760563380276, "Y"=328.91748251748254}, {"X"=189.26619718309854, "Y"=328.91748251748254}, {"X"=188.26478873239432, "Y"=329.9202797202797}, {"X"=187.2633802816901, "Y"=329.9202797202797}, {"X"=187.2633802816901, "Y"=330.92307692307696}, {"X"=187.2633802816901, "Y"=330.92307692307696}, {"X"=188.26478873239432, "Y"=329.9202797202797}, {"X"=189.26619718309854, "Y"=329.9202797202797}, {"X"=191.26901408450698, "Y"=328.91748251748254}, {"X"=194.2732394366197, "Y"=327.91468531468536}, {"X"=198.27887323943656, "Y"=327.91468531468536}, {"X"=200.281690140845, "Y"=327.91468531468536}, {"X"=203.2859154929577, "Y"=327.91468531468536}, {"X"=205.28873239436615, "Y"=328.91748251748254}, {"X"=206.29014084507037, "Y"=329.9202797202797}, {"X"=208.2929577464788, "Y"=330.92307692307696}, {"X"=209.29436619718302, "Y"=330.92307692307696}, {"X"=210.29577464788724, "Y"=332.9286713286713}, {"X"=211.29718309859152, "Y"=333.93146853146857}, {"X"=212.29859154929574, "Y"=335.93706293706293}, {"X"=214.30140845070417, "Y"=338.94545454545454}, {"X"=215.3028169014084, "Y"=340.95104895104896}, {"X"=216.3042253521126, "Y"=340.95104895104896}, {"X"=216.3042253521126, "Y"=341.9538461538462}, {"X"=216.3042253521126, "Y"=342.9566433566434}, {"X"=217.30563380281683, "Y"=342.9566433566434}, {"X"=217.30563380281683, "Y"=343.95944055944057}, {"X"=218.30704225352105, "Y"=344.9622377622378}, {"X"=218.30704225352105, "Y"=346.96783216783217}, {"X"=218.30704225352105, "Y"=347.9706293706294}, {"X"=218.30704225352105, "Y"=349.9762237762238}, {"X"=217.30563380281683, "Y"=349.9762237762238}, {"X"=217.30563380281683, "Y"=351.9818181818182}, {"X"=215.3028169014084, "Y"=353.9874125874126}, {"X"=214.30140845070417, "Y"=354.9902097902098}, {"X"=212.29859154929574, "Y"=355.993006993007}, {"X"=208.2929577464788, "Y"=357.9986013986014}, {"X"=206.29014084507037, "Y"=359.0013986013986}, {"X"=203.2859154929577, "Y"=360.00419580419583}, {"X"=200.281690140845, "Y"=362.00979020979025}, {"X"=194.2732394366197, "Y"=364.0153846153846}, {"X"=191.26901408450698, "Y"=365.01818181818186}, {"X"=188.26478873239432, "Y"=366.02097902097904}, {"X"=186.26197183098589, "Y"=366.02097902097904}, {"X"=184.2591549295774, "Y"=366.02097902097904}, {"X"=182.25633802816895, "Y"=367.0237762237762}, {"X"=180.25352112676052, "Y"=367.0237762237762}, {"X"=179.2521126760563, "Y"=368.02657342657346}, {"X"=178.25070422535205, "Y"=368.02657342657346}, {"X"=177.24929577464783, "Y"=368.02657342657346}, {"X"=176.24788732394362, "Y"=368.02657342657346}, {"X"=176.24788732394362, "Y"=369.02937062937065}, {"X"=175.2464788732394, "Y"=369.02937062937065}, {"X"=174.24507042253515, "Y"=369.02937062937065}, {"X"=174.24507042253515, "Y"=370.03216783216783}, {"X"=175.2464788732394, "Y"=369.02937062937065}, {"X"=175.2464788732394, "Y"=368.02657342657346}, {"X"=216.3042253521126, "Y"=352.9846153846154}, {"X"=223.3140845070422, "Y"=351.9818181818182}, {"X"=225.31690140845063, "Y"=353.9874125874126}, {"X"=230.32394366197178, "Y"=352.9846153846154}, {"X"=235.33098591549287, "Y"=350.979020979021}, {"X"=237.33380281690137, "Y"=350.979020979021}, {"X"=242.34084507042246, "Y"=349.9762237762238}, {"X"=246.3464788732394, "Y"=348.9734265734266}, {"X"=248.34929577464783, "Y"=348.9734265734266}, {"X"=256.36056338028163, "Y"=346.96783216783217}, {"X"=261.3676056338027, "Y"=344.9622377622378}, {"X"=264.37183098591544, "Y"=344.9622377622378}, {"X"=267.3760563380281, "Y"=343.95944055944057}, {"X"=269.37887323943653, "Y"=342.9566433566434}, {"X"=270.38028169014075, "Y"=342.9566433566434}, {"X"=271.381690140845, "Y"=342.9566433566434}, {"X"=272.38309859154924, "Y"=342.9566433566434}, {"X"=271.381690140845, "Y"=342.9566433566434}, {"X"=271.381690140845, "Y"=341.9538461538462}, {"X"=270.38028169014075, "Y"=341.9538461538462}, {"X"=269.37887323943653, "Y"=341.9538461538462}, {"X"=236.3323943661971, "Y"=349.9762237762238}, {"X"=233.32816901408444, "Y"=350.979020979021}, {"X"=236.3323943661971, "Y"=345.965034965035}, {"X"=238.3352112676056, "Y"=341.9538461538462}, {"X"=238.3352112676056, "Y"=339.9482517482518}, {"X"=239.3366197183098, "Y"=338.94545454545454}, {"X"=240.33802816901402, "Y"=337.94265734265736}, {"X"=241.33943661971824, "Y"=335.93706293706293}, {"X"=242.34084507042246, "Y"=333.93146853146857}, {"X"=244.3436619718309, "Y"=330.92307692307696}, {"X"=246.3464788732394, "Y"=327.91468531468536}, {"X"=246.3464788732394, "Y"=326.9118881118881}, {"X"=247.3478873239436, "Y"=323.9034965034965}, {"X"=249.35070422535205, "Y"=320.8951048951049}, {"X"=250.35211267605627, "Y"=318.8895104895105}, {"X"=251.35352112676048, "Y"=315.8811188811189}, {"X"=252.3549295774647, "Y"=314.8783216783217}, {"X"=253.35633802816892, "Y"=312.8727272727273}, {"X"=253.35633802816892, "Y"=311.8699300699301}, {"X"=254.3577464788732, "Y"=308.8615384615385}, {"X"=255.35915492957741, "Y"=307.8587412587413}, {"X"=255.35915492957741, "Y"=306.85594405594406}, {"X"=256.36056338028163, "Y"=306.85594405594406}, {"X"=256.36056338028163, "Y"=305.8531468531469}, {"X"=256.36056338028163, "Y"=304.8503496503497}, {"X"=255.35915492957741, "Y"=304.8503496503497}, {"X"=254.3577464788732, "Y"=304.8503496503497}, {"X"=253.35633802816892, "Y"=304.8503496503497}, {"X"=252.3549295774647, "Y"=305.8531468531469}, {"X"=250.35211267605627, "Y"=305.8531468531469}, {"X"=249.35070422535205, "Y"=305.8531468531469}, {"X"=247.3478873239436, "Y"=306.85594405594406}, {"X"=245.34507042253517, "Y"=306.85594405594406}, {"X"=241.33943661971824, "Y"=307.8587412587413}, {"X"=237.33380281690137, "Y"=308.8615384615385}, {"X"=236.3323943661971, "Y"=309.86433566433567}, {"X"=235.33098591549287, "Y"=310.8671328671329}, {"X"=234.32957746478866, "Y"=310.8671328671329}, {"X"=233.32816901408444, "Y"=310.8671328671329}, {"X"=232.32676056338022, "Y"=310.8671328671329}, {"X"=231.325352112676, "Y"=310.8671328671329}, {"X"=231.325352112676, "Y"=311.8699300699301}, {"X"=231.325352112676, "Y"=310.8671328671329}, {"X"=232.32676056338022, "Y"=310.8671328671329}, {"X"=234.32957746478866, "Y"=310.8671328671329}, {"X"=237.33380281690137, "Y"=309.86433566433567}, {"X"=244.3436619718309, "Y"=308.8615384615385}, {"X"=250.35211267605627, "Y"=307.8587412587413}, {"X"=259.3647887323943, "Y"=306.85594405594406}, {"X"=260.3661971830985, "Y"=305.8531468531469}, {"X"=267.3760563380281, "Y"=304.8503496503497}, {"X"=271.381690140845, "Y"=303.84755244755246}, {"X"=275.3873239436619, "Y"=302.8447552447553}, {"X"=276.3887323943661, "Y"=302.8447552447553}, {"X"=277.39014084507033, "Y"=302.8447552447553}, {"X"=280.39436619718305, "Y"=302.8447552447553}, {"X"=281.39577464788727, "Y"=301.84195804195804}, {"X"=282.3971830985915, "Y"=301.84195804195804}, {"X"=283.3985915492957, "Y"=301.84195804195804}, {"X"=284.3999999999999, "Y"=301.84195804195804}, {"X"=285.40140845070414, "Y"=301.84195804195804}, {"X"=284.3999999999999, "Y"=301.84195804195804}, {"X"=296.4169014084506, "Y"=310.8671328671329}, {"X"=297.4183098591549, "Y"=310.8671328671329}, {"X"=301.42394366197175, "Y"=308.8615384615385}, {"X"=308.43380281690133, "Y"=306.85594405594406}, {"X"=311.438028169014, "Y"=305.8531468531469}, {"X"=313.4408450704224, "Y"=304.8503496503497}, {"X"=316.44507042253514, "Y"=303.84755244755246}, {"X"=319.4492957746478, "Y"=303.84755244755246}, {"X"=320.450704225352, "Y"=303.84755244755246}, {"X"=325.45774647887316, "Y"=302.8447552447553}, {"X"=327.4605633802816, "Y"=301.84195804195804}, {"X"=329.46338028169004, "Y"=301.84195804195804}, {"X"=330.46478873239425, "Y"=300.83916083916085}, {"X"=332.46760563380275, "Y"=300.83916083916085}, {"X"=333.46901408450697, "Y"=300.83916083916085}, {"X"=334.4704225352112, "Y"=300.83916083916085}, {"X"=335.4718309859154, "Y"=300.83916083916085}, {"X"=336.4732394366196, "Y"=300.83916083916085}, {"X"=337.47464788732384, "Y"=300.83916083916085}, {"X"=338.47605633802806, "Y"=300.83916083916085}, {"X"=338.47605633802806, "Y"=299.83636363636367}, {"X"=337.47464788732384, "Y"=300.83916083916085}, {"X"=335.4718309859154, "Y"=300.83916083916085}, {"X"=329.46338028169004, "Y"=302.8447552447553}, {"X"=325.45774647887316, "Y"=304.8503496503497}, {"X"=323.4549295774647, "Y"=305.8531468531469}, {"X"=321.45211267605623, "Y"=305.8531468531469}, {"X"=320.450704225352, "Y"=305.8531468531469}, {"X"=319.4492957746478, "Y"=306.85594405594406}, {"X"=318.4478873239436, "Y"=305.8531468531469}, {"X"=318.4478873239436, "Y"=306.85594405594406}, {"X"=318.4478873239436, "Y"=305.8531468531469}, {"X"=319.4492957746478, "Y"=305.8531468531469}, {"X"=318.4478873239436, "Y"=306.85594405594406}, {"X"=317.44647887323936, "Y"=307.8587412587413}, {"X"=317.44647887323936, "Y"=308.8615384615385}, {"X"=315.4436619718309, "Y"=311.8699300699301}, {"X"=313.4408450704224, "Y"=315.8811188811189}, {"X"=312.4394366197182, "Y"=317.8867132867133}, {"X"=309.43521126760555, "Y"=321.8979020979021}, {"X"=304.4281690140844, "Y"=328.91748251748254}, {"X"=300.42253521126753, "Y"=333.93146853146857}, {"X"=299.4211267605633, "Y"=335.93706293706293}, {"X"=298.4197183098591, "Y"=337.94265734265736}, {"X"=297.4183098591549, "Y"=337.94265734265736}, {"X"=296.4169014084506, "Y"=339.9482517482518}, {"X"=296.4169014084506, "Y"=340.95104895104896}, {"X"=295.4154929577464, "Y"=340.95104895104896}, {"X"=296.4169014084506, "Y"=339.9482517482518}, {"X"=296.4169014084506, "Y"=338.94545454545454}, {"X"=316.44507042253514, "Y"=304.8503496503497}, {"X"=335.4718309859154, "Y"=299.83636363636367}, {"X"=359.5056338028168, "Y"=301.84195804195804}, {"X"=352.49577464788723, "Y"=303.84755244755246}, {"X"=352.49577464788723, "Y"=304.8503496503497}, {"X"=353.49718309859145, "Y"=304.8503496503497}, {"X"=354.49859154929567, "Y"=303.84755244755246}, {"X"=355.4999999999999, "Y"=303.84755244755246}, {"X"=357.5028169014084, "Y"=303.84755244755246}, {"X"=360.50704225352104, "Y"=303.84755244755246}, {"X"=362.5098591549295, "Y"=303.84755244755246}, {"X"=369.51971830985906, "Y"=301.84195804195804}, {"X"=373.52535211267593, "Y"=300.83916083916085}, {"X"=378.5323943661971, "Y"=299.83636363636367}, {"X"=386.5436619718309, "Y"=297.83076923076925}, {"X"=392.55211267605625, "Y"=296.82797202797207}, {"X"=396.5577464788731, "Y"=295.8251748251748}, {"X"=400.56338028169006, "Y"=294.82237762237764}, {"X"=405.57042253521115, "Y"=294.82237762237764}, {"X"=407.5732394366196, "Y"=294.82237762237764}, {"X"=408.57464788732386, "Y"=294.82237762237764}, {"X"=409.5760563380281, "Y"=293.81958041958046}, {"X"=410.5774647887323, "Y"=293.81958041958046}, {"X"=411.5788732394365, "Y"=293.81958041958046}, {"X"=412.58028169014074, "Y"=293.81958041958046}, {"X"=411.5788732394365, "Y"=293.81958041958046}, {"X"=410.5774647887323, "Y"=294.82237762237764}, {"X"=409.5760563380281, "Y"=294.82237762237764}, {"X"=408.57464788732386, "Y"=294.82237762237764}, {"X"=406.57183098591537, "Y"=294.82237762237764}, {"X"=400.56338028169006, "Y"=296.82797202797207}, {"X"=392.55211267605625, "Y"=297.83076923076925}, {"X"=390.54929577464776, "Y"=297.83076923076925}, {"X"=384.54084507042245, "Y"=298.83356643356643}, {"X"=381.53661971830974, "Y"=298.83356643356643}, {"X"=380.5352112676055, "Y"=299.83636363636367}, {"X"=379.5338028169013, "Y"=299.83636363636367}, {"X"=378.5323943661971, "Y"=299.83636363636367}, {"X"=377.53098591549286, "Y"=299.83636363636367}, {"X"=378.5323943661971, "Y"=299.83636363636367}, {"X"=377.53098591549286, "Y"=299.83636363636367}, {"X"=377.53098591549286, "Y"=300.83916083916085}, {"X"=376.52957746478864, "Y"=303.84755244755246}, {"X"=374.5267605633802, "Y"=311.8699300699301}, {"X"=373.52535211267593, "Y"=313.8755244755245}, {"X"=370.5211267605633, "Y"=321.8979020979021}, {"X"=369.51971830985906, "Y"=325.90909090909093}, {"X"=368.51830985915484, "Y"=329.9202797202797}, {"X"=367.5169014084506, "Y"=332.9286713286713}, {"X"=366.5154929577464, "Y"=333.93146853146857}, {"X"=366.5154929577464, "Y"=335.93706293706293}, {"X"=366.5154929577464, "Y"=336.9398601398602}, {"X"=365.5140845070422, "Y"=336.9398601398602}, {"X"=364.5126760563379, "Y"=336.9398601398602}, {"X"=363.5112676056337, "Y"=336.9398601398602}, {"X"=362.5098591549295, "Y"=337.94265734265736}, {"X"=359.5056338028168, "Y"=338.94545454545454}, {"X"=358.5042253521126, "Y"=338.94545454545454}, {"X"=355.4999999999999, "Y"=339.9482517482518}, {"X"=352.49577464788723, "Y"=340.95104895104896}, {"X"=347.4887323943661, "Y"=341.9538461538462}, {"X"=344.4845070422534, "Y"=342.9566433566434}, {"X"=343.4830985915492, "Y"=342.9566433566434}, {"X"=342.481690140845, "Y"=342.9566433566434}, {"X"=340.47887323943655, "Y"=343.95944055944057}, {"X"=338.47605633802806, "Y"=343.95944055944057}, {"X"=337.47464788732384, "Y"=344.9622377622378}, {"X"=336.4732394366196, "Y"=344.9622377622378}, {"X"=337.47464788732384, "Y"=344.9622377622378}, {"X"=338.47605633802806, "Y"=344.9622377622378}, {"X"=339.47746478873233, "Y"=343.95944055944057}, {"X"=342.481690140845, "Y"=343.95944055944057}, {"X"=346.48732394366186, "Y"=342.9566433566434}, {"X"=352.49577464788723, "Y"=340.95104895104896}, {"X"=357.5028169014084, "Y"=338.94545454545454}, {"X"=367.5169014084506, "Y"=334.93426573426575}, {"X"=375.5281690140844, "Y"=331.92587412587415}, {"X"=381.53661971830974, "Y"=328.91748251748254}, {"X"=385.54225352112667, "Y"=327.91468531468536}, {"X"=390.54929577464776, "Y"=325.90909090909093}, {"X"=393.5535211267605, "Y"=324.90629370629375}, {"X"=395.5563380281689, "Y"=324.90629370629375}, {"X"=396.5577464788731, "Y"=324.90629370629375}, {"X"=396.5577464788731, "Y"=323.9034965034965}, {"X"=397.55915492957735, "Y"=323.9034965034965}, {"X"=422.594366197183, "Y"=297.83076923076925}, {"X"=419.5901408450703, "Y"=301.84195804195804}, {"X"=418.5887323943661, "Y"=303.84755244755246}, {"X"=417.5873239436619, "Y"=303.84755244755246}, {"X"=415.5845070422534, "Y"=304.8503496503497}, {"X"=415.5845070422534, "Y"=306.85594405594406}, {"X"=414.5830985915492, "Y"=307.8587412587413}, {"X"=413.58169014084496, "Y"=308.8615384615385}, {"X"=412.58028169014074, "Y"=309.86433566433567}, {"X"=411.5788732394365, "Y"=311.8699300699301}, {"X"=410.5774647887323, "Y"=312.8727272727273}, {"X"=409.5760563380281, "Y"=314.8783216783217}, {"X"=408.57464788732386, "Y"=316.8839160839161}, {"X"=407.5732394366196, "Y"=318.8895104895105}, {"X"=406.57183098591537, "Y"=320.8951048951049}, {"X"=406.57183098591537, "Y"=321.8979020979021}, {"X"=405.57042253521115, "Y"=321.8979020979021}, {"X"=405.57042253521115, "Y"=322.90069930069933}, {"X"=405.57042253521115, "Y"=323.9034965034965}, {"X"=405.57042253521115, "Y"=324.90629370629375}, {"X"=405.57042253521115, "Y"=325.90909090909093}, {"X"=405.57042253521115, "Y"=326.9118881118881}, {"X"=405.57042253521115, "Y"=327.91468531468536}, {"X"=405.57042253521115, "Y"=328.91748251748254}, {"X"=406.57183098591537, "Y"=329.9202797202797}, {"X"=406.57183098591537, "Y"=330.92307692307696}, {"X"=407.5732394366196, "Y"=330.92307692307696}, {"X"=408.57464788732386, "Y"=331.92587412587415}, {"X"=410.5774647887323, "Y"=331.92587412587415}, {"X"=411.5788732394365, "Y"=331.92587412587415}, {"X"=414.5830985915492, "Y"=331.92587412587415}, {"X"=417.5873239436619, "Y"=329.9202797202797}, {"X"=418.5887323943661, "Y"=329.9202797202797}, {"X"=420.59154929577454, "Y"=327.91468531468536}, {"X"=423.5957746478872, "Y"=325.90909090909093}, {"X"=424.5971830985914, "Y"=324.90629370629375}, {"X"=426.5999999999999, "Y"=323.9034965034965}, {"X"=428.60281690140835, "Y"=322.90069930069933}, {"X"=429.60422535211256, "Y"=321.8979020979021}, {"X"=431.607042253521, "Y"=320.8951048951049}, {"X"=433.6098591549295, "Y"=318.8895104895105}, {"X"=436.61408450704215, "Y"=316.8839160839161}, {"X"=437.61549295774637, "Y"=315.8811188811189}, {"X"=438.61690140845064, "Y"=313.8755244755245}, {"X"=439.6183098591548, "Y"=311.8699300699301}, {"X"=440.6197183098591, "Y"=308.8615384615385}, {"X"=441.62112676056324, "Y"=308.8615384615385}, {"X"=440.6197183098591, "Y"=305.8531468531469}, {"X"=440.6197183098591, "Y"=303.84755244755246}, {"X"=440.6197183098591, "Y"=302.8447552447553}, {"X"=440.6197183098591, "Y"=301.84195804195804}, {"X"=439.6183098591548, "Y"=301.84195804195804}, {"X"=439.6183098591548, "Y"=300.83916083916085}, {"X"=439.6183098591548, "Y"=299.83636363636367}, {"X"=439.6183098591548, "Y"=298.83356643356643}, {"X"=439.6183098591548, "Y"=297.83076923076925}, {"X"=438.61690140845064, "Y"=297.83076923076925}, {"X"=435.61267605633793, "Y"=296.82797202797207}, {"X"=433.6098591549295, "Y"=296.82797202797207}, {"X"=431.607042253521, "Y"=296.82797202797207}, {"X"=430.6056338028168, "Y"=296.82797202797207}, {"X"=428.60281690140835, "Y"=296.82797202797207}, {"X"=426.5999999999999, "Y"=296.82797202797207}, {"X"=425.5985915492957, "Y"=296.82797202797207}, {"X"=424.5971830985914, "Y"=297.83076923076925}, {"X"=422.594366197183, "Y"=298.83356643356643}, {"X"=420.59154929577454, "Y"=299.83636363636367}, {"X"=419.5901408450703, "Y"=300.83916083916085}, {"X"=418.5887323943661, "Y"=301.84195804195804}, {"X"=417.5873239436619, "Y"=302.8447552447553}, {"X"=417.5873239436619, "Y"=303.84755244755246}, {"X"=427.6014084507041, "Y"=296.82797202797207}, {"X"=438.61690140845064, "Y"=294.82237762237764}, {"X"=458.6450704225351, "Y"=298.83356643356643}, {"X"=457.64366197183085, "Y"=301.84195804195804}, {"X"=457.64366197183085, "Y"=302.8447552447553}, {"X"=456.6422535211267, "Y"=303.84755244755246}, {"X"=456.6422535211267, "Y"=304.8503496503497}, {"X"=456.6422535211267, "Y"=305.8531468531469}, {"X"=455.6408450704224, "Y"=307.8587412587413}, {"X"=455.6408450704224, "Y"=308.8615384615385}, {"X"=455.6408450704224, "Y"=309.86433566433567}, {"X"=455.6408450704224, "Y"=310.8671328671329}, {"X"=454.63943661971814, "Y"=313.8755244755245}, {"X"=454.63943661971814, "Y"=314.8783216783217}, {"X"=453.638028169014, "Y"=316.8839160839161}, {"X"=453.638028169014, "Y"=318.8895104895105}, {"X"=453.638028169014, "Y"=319.8923076923077}, {"X"=453.638028169014, "Y"=320.8951048951049}, {"X"=453.638028169014, "Y"=322.90069930069933}, {"X"=452.6366197183097, "Y"=323.9034965034965}, {"X"=452.6366197183097, "Y"=324.90629370629375}, {"X"=452.6366197183097, "Y"=325.90909090909093}, {"X"=452.6366197183097, "Y"=326.9118881118881}, {"X"=452.6366197183097, "Y"=327.91468531468536}, {"X"=453.638028169014, "Y"=328.91748251748254}, {"X"=453.638028169014, "Y"=329.9202797202797}, {"X"=454.63943661971814, "Y"=330.92307692307696}, {"X"=456.6422535211267, "Y"=331.92587412587415}, {"X"=458.6450704225351, "Y"=331.92587412587415}, {"X"=459.6464788732393, "Y"=330.92307692307696}, {"X"=461.6492957746477, "Y"=330.92307692307696}, {"X"=464.65352112676044, "Y"=329.9202797202797}, {"X"=467.65774647887315, "Y"=328.91748251748254}, {"X"=469.6605633802816, "Y"=326.9118881118881}, {"X"=472.6647887323943, "Y"=324.90629370629375}, {"X"=474.66760563380274, "Y"=323.9034965034965}, {"X"=475.6690140845069, "Y"=322.90069930069933}, {"X"=477.67183098591534, "Y"=320.8951048951049}, {"X"=482.6788732394365, "Y"=317.8867132867133}, {"X"=483.68028169014076, "Y"=316.8839160839161}, {"X"=486.68450704225336, "Y"=314.8783216783217}, {"X"=489.68873239436607, "Y"=309.86433566433567}, {"X"=490.69014084507035, "Y"=307.8587412587413}, {"X"=492.6929577464788, "Y"=304.8503496503497}, {"X"=495.6971830985914, "Y"=300.83916083916085}, {"X"=495.6971830985914, "Y"=298.83356643356643}, {"X"=496.69859154929566, "Y"=296.82797202797207}, {"X"=496.69859154929566, "Y"=295.8251748251748}, {"X"=497.69999999999993, "Y"=293.81958041958046}, {"X"=497.69999999999993, "Y"=292.8167832167832}, {"X"=497.69999999999993, "Y"=291.81398601398604}, {"X"=497.69999999999993, "Y"=290.81118881118886}, {"X"=498.7014084507041, "Y"=290.81118881118886}, {"X"=498.7014084507041, "Y"=289.8083916083916}, {"X"=498.7014084507041, "Y"=288.80559440559443}, {"X"=497.69999999999993, "Y"=288.80559440559443}, {"X"=496.69859154929566, "Y"=289.8083916083916}, {"X"=496.69859154929566, "Y"=290.81118881118886}, {"X"=495.6971830985914, "Y"=291.81398601398604}, {"X"=495.6971830985914, "Y"=292.8167832167832}, {"X"=494.6957746478872, "Y"=294.82237762237764}, {"X"=493.69436619718294, "Y"=296.82797202797207}, {"X"=492.6929577464788, "Y"=299.83636363636367}, {"X"=492.6929577464788, "Y"=300.83916083916085}, {"X"=490.69014084507035, "Y"=305.8531468531469}, {"X"=488.6873239436618, "Y"=310.8671328671329}, {"X"=487.68591549295763, "Y"=312.8727272727273}, {"X"=486.68450704225336, "Y"=316.8839160839161}, {"X"=485.6830985915492, "Y"=318.8895104895105}, {"X"=485.6830985915492, "Y"=320.8951048951049}, {"X"=485.6830985915492, "Y"=321.8979020979021}, {"X"=484.6816901408449, "Y"=321.8979020979021}, {"X"=484.6816901408449, "Y"=322.90069930069933}, {"X"=484.6816901408449, "Y"=323.9034965034965}, {"X"=484.6816901408449, "Y"=324.90629370629375}, {"X"=484.6816901408449, "Y"=325.90909090909093}, {"X"=484.6816901408449, "Y"=326.9118881118881}, {"X"=483.68028169014076, "Y"=326.9118881118881}, {"X"=484.6816901408449, "Y"=326.9118881118881}, {"X"=484.6816901408449, "Y"=325.90909090909093}, {"X"=483.68028169014076, "Y"=324.90629370629375}, {"X"=482.6788732394365, "Y"=324.90629370629375}, {"X"=482.6788732394365, "Y"=323.9034965034965}, {"X"=491.6915492957745, "Y"=328.91748251748254}, {"X"=492.6929577464788, "Y"=327.91468531468536}, {"X"=494.6957746478872, "Y"=329.9202797202797}, {"X"=496.69859154929566, "Y"=329.9202797202797}, {"X"=497.69999999999993, "Y"=329.9202797202797}, {"X"=498.7014084507041, "Y"=329.9202797202797}, {"X"=499.70281690140837, "Y"=329.9202797202797}, {"X"=500.70422535211253, "Y"=329.9202797202797}, {"X"=501.7056338028168, "Y"=329.9202797202797}, {"X"=503.70845070422524, "Y"=329.9202797202797}, {"X"=504.7098591549294, "Y"=329.9202797202797}, {"X"=505.7112676056337, "Y"=329.9202797202797}, {"X"=507.7140845070421, "Y"=329.9202797202797}, {"X"=509.71690140845055, "Y"=329.9202797202797}, {"X"=510.71830985915483, "Y"=329.9202797202797}, {"X"=511.719718309859, "Y"=329.9202797202797}, {"X"=513.7225352112674, "Y"=328.91748251748254}, {"X"=514.7239436619717, "Y"=328.91748251748254}, {"X"=515.725352112676, "Y"=328.91748251748254}, {"X"=516.7267605633801, "Y"=328.91748251748254}, {"X"=517.7281690140844, "Y"=328.91748251748254}, {"X"=518.7295774647886, "Y"=327.91468531468536}, {"X"=519.7309859154929, "Y"=327.91468531468536}, {"X"=520.732394366197, "Y"=326.9118881118881}, {"X"=521.7338028169013, "Y"=326.9118881118881}, {"X"=522.7352112676055, "Y"=325.90909090909093}, {"X"=522.7352112676055, "Y"=324.90629370629375}, {"X"=523.7366197183097, "Y"=323.9034965034965}, {"X"=523.7366197183097, "Y"=322.90069930069933}, {"X"=523.7366197183097, "Y"=321.8979020979021}, {"X"=523.7366197183097, "Y"=320.8951048951049}, {"X"=523.7366197183097, "Y"=319.8923076923077}, {"X"=523.7366197183097, "Y"=318.8895104895105}, {"X"=522.7352112676055, "Y"=317.8867132867133}, {"X"=522.7352112676055, "Y"=316.8839160839161}, {"X"=521.7338028169013, "Y"=315.8811188811189}, {"X"=520.732394366197, "Y"=314.8783216783217}, {"X"=520.732394366197, "Y"=313.8755244755245}, {"X"=519.7309859154929, "Y"=313.8755244755245}, {"X"=519.7309859154929, "Y"=312.8727272727273}, {"X"=517.7281690140844, "Y"=311.8699300699301}, {"X"=516.7267605633801, "Y"=309.86433566433567}, {"X"=515.725352112676, "Y"=307.8587412587413}, {"X"=514.7239436619717, "Y"=307.8587412587413}, {"X"=514.7239436619717, "Y"=305.8531468531469}, {"X"=513.7225352112674, "Y"=304.8503496503497}, {"X"=513.7225352112674, "Y"=302.8447552447553}, {"X"=512.7211267605633, "Y"=302.8447552447553}, {"X"=512.7211267605633, "Y"=301.84195804195804}, {"X"=512.7211267605633, "Y"=300.83916083916085}, {"X"=511.719718309859, "Y"=299.83636363636367}, {"X"=511.719718309859, "Y"=298.83356643356643}, {"X"=510.71830985915483, "Y"=297.83076923076925}, {"X"=510.71830985915483, "Y"=296.82797202797207}, {"X"=510.71830985915483, "Y"=295.8251748251748}, {"X"=510.71830985915483, "Y"=294.82237762237764}, {"X"=510.71830985915483, "Y"=293.81958041958046}, {"X"=510.71830985915483, "Y"=292.8167832167832}, {"X"=510.71830985915483, "Y"=291.81398601398604}, {"X"=510.71830985915483, "Y"=290.81118881118886}, {"X"=511.719718309859, "Y"=289.8083916083916}, {"X"=512.7211267605633, "Y"=288.80559440559443}, {"X"=513.7225352112674, "Y"=287.80279720279725}, {"X"=514.7239436619717, "Y"=286.8}, {"X"=516.7267605633801, "Y"=286.8}, {"X"=517.7281690140844, "Y"=285.79720279720283}, {"X"=518.7295774647886, "Y"=285.79720279720283}, {"X"=519.7309859154929, "Y"=285.79720279720283}, {"X"=520.732394366197, "Y"=285.79720279720283}, {"X"=521.7338028169013, "Y"=285.79720279720283}, {"X"=522.7352112676055, "Y"=286.8}, {"X"=523.7366197183097, "Y"=286.8}, {"X"=525.7394366197182, "Y"=287.80279720279725}, {"X"=526.7408450704224, "Y"=288.80559440559443}, {"X"=527.7422535211266, "Y"=289.8083916083916}, {"X"=527.7422535211266, "Y"=290.81118881118886}, {"X"=528.7436619718309, "Y"=290.81118881118886}, {"X"=528.7436619718309, "Y"=291.81398601398604}, {"X"=529.745070422535, "Y"=290.81118881118886}, {"X"=551.7760563380281, "Y"=293.81958041958046}, {"X"=549.7732394366196, "Y"=297.83076923076925}, {"X"=548.7718309859154, "Y"=299.83636363636367}, {"X"=547.7704225352111, "Y"=301.84195804195804}, {"X"=547.7704225352111, "Y"=302.8447552447553}, {"X"=546.7690140845069, "Y"=303.84755244755246}, {"X"=545.7676056338026, "Y"=304.8503496503497}, {"X"=545.7676056338026, "Y"=306.85594405594406}, {"X"=544.7661971830985, "Y"=308.8615384615385}, {"X"=543.7647887323942, "Y"=311.8699300699301}, {"X"=543.7647887323942, "Y"=312.8727272727273}, {"X"=542.76338028169, "Y"=314.8783216783217}, {"X"=542.76338028169, "Y"=317.8867132867133}, {"X"=541.7619718309858, "Y"=318.8895104895105}, {"X"=540.7605633802816, "Y"=320.8951048951049}, {"X"=540.7605633802816, "Y"=321.8979020979021}, {"X"=539.7591549295773, "Y"=323.9034965034965}, {"X"=538.7577464788731, "Y"=324.90629370629375}, {"X"=537.7563380281689, "Y"=326.9118881118881}, {"X"=537.7563380281689, "Y"=328.91748251748254}, {"X"=536.7549295774646, "Y"=329.9202797202797}, {"X"=535.7535211267605, "Y"=331.92587412587415}, {"X"=535.7535211267605, "Y"=332.9286713286713}, {"X"=534.7521126760562, "Y"=333.93146853146857}, {"X"=534.7521126760562, "Y"=334.93426573426575}, {"X"=533.750704225352, "Y"=335.93706293706293}, {"X"=533.750704225352, "Y"=336.9398601398602}, {"X"=533.750704225352, "Y"=337.94265734265736}, {"X"=532.7492957746477, "Y"=337.94265734265736}, {"X"=532.7492957746477, "Y"=338.94545454545454}, {"X"=533.750704225352, "Y"=337.94265734265736}, {"X"=534.7521126760562, "Y"=336.9398601398602}, {"X"=535.7535211267605, "Y"=336.9398601398602}, {"X"=535.7535211267605, "Y"=335.93706293706293}, {"X"=536.7549295774646, "Y"=335.93706293706293}, {"X"=537.7563380281689, "Y"=335.93706293706293}, {"X"=538.7577464788731, "Y"=334.93426573426575}, {"X"=539.7591549295773, "Y"=334.93426573426575}, {"X"=541.7619718309858, "Y"=333.93146853146857}, {"X"=543.7647887323942, "Y"=332.9286713286713}, {"X"=545.7676056338026, "Y"=332.9286713286713}, {"X"=546.7690140845069, "Y"=332.9286713286713}, {"X"=547.7704225352111, "Y"=332.9286713286713}, {"X"=548.7718309859154, "Y"=332.9286713286713}, {"X"=550.7746478873238, "Y"=332.9286713286713}, {"X"=553.7788732394365, "Y"=333.93146853146857}, {"X"=554.7802816901407, "Y"=333.93146853146857}, {"X"=556.7830985915491, "Y"=334.93426573426575}, {"X"=558.7859154929577, "Y"=335.93706293706293}, {"X"=559.7873239436618, "Y"=335.93706293706293}, {"X"=562.7915492957745, "Y"=335.93706293706293}, {"X"=563.7929577464787, "Y"=335.93706293706293}, {"X"=564.794366197183, "Y"=335.93706293706293}, {"X"=565.7957746478872, "Y"=335.93706293706293}, {"X"=566.7971830985914, "Y"=335.93706293706293}, {"X"=565.7957746478872, "Y"=335.93706293706293}, {"X"=565.7957746478872, "Y"=334.93426573426575}, {"X"=585.8239436619717, "Y"=293.81958041958046}, {"X"=588.8281690140843, "Y"=298.83356643356643}, {"X"=591.832394366197, "Y"=302.8447552447553}, {"X"=592.8338028169013, "Y"=304.8503496503497}, {"X"=594.8366197183097, "Y"=307.8587412587413}, {"X"=595.8380281690139, "Y"=309.86433566433567}, {"X"=596.8394366197182, "Y"=311.8699300699301}, {"X"=597.8408450704223, "Y"=312.8727272727273}, {"X"=598.8422535211266, "Y"=313.8755244755245}, {"X"=599.8436619718308, "Y"=313.8755244755245}, {"X"=599.8436619718308, "Y"=314.8783216783217}, {"X"=599.8436619718308, "Y"=313.8755244755245}, {"X"=598.8422535211266, "Y"=313.8755244755245}, {"X"=598.8422535211266, "Y"=312.8727272727273}, {"X"=620.8732394366195, "Y"=290.81118881118886}, {"X"=618.8704225352111, "Y"=295.8251748251748}, {"X"=616.8676056338027, "Y"=298.83356643356643}, {"X"=614.8647887323942, "Y"=300.83916083916085}, {"X"=613.86338028169, "Y"=302.8447552447553}, {"X"=612.8619718309858, "Y"=304.8503496503497}, {"X"=612.8619718309858, "Y"=305.8531468531469}, {"X"=610.8591549295774, "Y"=307.8587412587413}, {"X"=609.8577464788731, "Y"=310.8671328671329}, {"X"=608.8563380281689, "Y"=312.8727272727273}, {"X"=605.8521126760562, "Y"=316.8839160839161}, {"X"=603.8492957746478, "Y"=318.8895104895105}, {"X"=600.8450704225351, "Y"=323.9034965034965}, {"X"=599.8436619718308, "Y"=325.90909090909093}, {"X"=596.8394366197182, "Y"=328.91748251748254}, {"X"=594.8366197183097, "Y"=331.92587412587415}, {"X"=593.8352112676055, "Y"=333.93146853146857}, {"X"=591.832394366197, "Y"=334.93426573426575}, {"X"=589.8295774647886, "Y"=337.94265734265736}, {"X"=588.8281690140843, "Y"=338.94545454545454}, {"X"=588.8281690140843, "Y"=339.9482517482518}, {"X"=587.8267605633802, "Y"=339.9482517482518}, {"X"=587.8267605633802, "Y"=340.95104895104896}, {"X"=586.8253521126759, "Y"=341.9538461538462}, {"X"=586.8253521126759, "Y"=342.9566433566434}, {"X"=585.8239436619717, "Y"=342.9566433566434}, {"X"=586.8253521126759, "Y"=342.9566433566434}, {"X"=586.8253521126759, "Y"=341.9538461538462}, {"X"=585.8239436619717, "Y"=340.95104895104896}, {"X"=592.8338028169013, "Y"=348.9734265734266}, {"X"=598.8422535211266, "Y"=343.95944055944057}, {"X"=601.8464788732393, "Y"=342.9566433566434}, {"X"=604.8507042253519, "Y"=341.9538461538462}, {"X"=607.8549295774646, "Y"=340.95104895104896}, {"X"=608.8563380281689, "Y"=339.9482517482518}, {"X"=610.8591549295774, "Y"=339.9482517482518}, {"X"=611.8605633802815, "Y"=338.94545454545454}, {"X"=613.86338028169, "Y"=337.94265734265736}, {"X"=617.869014084507, "Y"=336.9398601398602}, {"X"=621.8746478873238, "Y"=334.93426573426575}, {"X"=624.8788732394364, "Y"=333.93146853146857}, {"X"=632.8901408450703, "Y"=331.92587412587415}, {"X"=637.8971830985914, "Y"=329.9202797202797}, {"X"=649.914084507042, "Y"=326.9118881118881}, {"X"=652.9183098591548, "Y"=325.90909090909093}, {"X"=666.9380281690139, "Y"=322.90069930069933}, {"X"=681.9591549295773, "Y"=319.8923076923077}, {"X"=689.9704225352111, "Y"=318.8895104895105}, {"X"=699.9845070422533, "Y"=316.8839160839161}, {"X"=706.9943661971829, "Y"=316.8839160839161}, {"X"=720.0126760563379, "Y"=315.8811188811189}, {"X"=734.032394366197, "Y"=316.8839160839161}, {"X"=744.0464788732393, "Y"=317.8867132867133}, {"X"=752.057746478873, "Y"=319.8923076923077}, {"X"=757.0647887323942, "Y"=321.8979020979021}, {"X"=766.0774647887322, "Y"=324.90629370629375}, {"X"=772.0859154929576, "Y"=326.9118881118881}, {"X"=779.0957746478871, "Y"=330.92307692307696}, {"X"=781.0985915492956, "Y"=332.9286713286713}, {"X"=786.1056338028167, "Y"=336.9398601398602}, {"X"=787.107042253521, "Y"=338.94545454545454}, {"X"=789.1098591549294, "Y"=343.95944055944057}, {"X"=788.1084507042252, "Y"=349.9762237762238}, {"X"=787.107042253521, "Y"=352.9846153846154}, {"X"=782.0999999999998, "Y"=361.006993006993}, {"X"=778.0943661971829, "Y"=365.01818181818186}, {"X"=769.0816901408449, "Y"=373.04055944055943}, {"X"=764.0746478873237, "Y"=377.0517482517483}, {"X"=753.0591549295773, "Y"=384.0713286713287}, {"X"=746.0492957746477, "Y"=386.0769230769231}, {"X"=734.032394366197, "Y"=392.0937062937063}, {"X"=725.019718309859, "Y"=395.1020979020979}, {"X"=714.0042253521125, "Y"=399.11328671328675}, {"X"=703.9901408450703, "Y"=402.12167832167836}, {"X"=698.9830985915492, "Y"=403.12447552447554}, {"X"=691.9732394366196, "Y"=405.13006993006996}, {"X"=686.9661971830984, "Y"=406.13286713286715}, {"X"=672.9464788732392, "Y"=408.13846153846157}, {"X"=667.9394366197181, "Y"=409.14125874125875}, {"X"=656.9239436619716, "Y"=410.14405594405594}, {"X"=651.9169014084506, "Y"=411.1468531468532}, {"X"=641.9028169014083, "Y"=411.1468531468532}, {"X"=635.894366197183, "Y"=411.1468531468532}, {"X"=623.8774647887323, "Y"=410.14405594405594}, {"X"=613.86338028169, "Y"=409.14125874125875}, {"X"=608.8563380281689, "Y"=408.13846153846157}, {"X"=597.8408450704223, "Y"=407.13566433566433}, {"X"=591.832394366197, "Y"=407.13566433566433}, {"X"=576.8112676056337, "Y"=406.13286713286715}, {"X"=571.8042253521126, "Y"=405.13006993006996}, {"X"=562.7915492957745, "Y"=405.13006993006996}, {"X"=560.7887323943661, "Y"=405.13006993006996}, {"X"=549.7732394366196, "Y"=404.1272727272727}, {"X"=540.7605633802816, "Y"=405.13006993006996}, {"X"=534.7521126760562, "Y"=405.13006993006996}, {"X"=521.7338028169013, "Y"=407.13566433566433}, {"X"=516.7267605633801, "Y"=408.13846153846157}, {"X"=507.7140845070421, "Y"=411.1468531468532}, {"X"=503.70845070422524, "Y"=413.15244755244754}, {"X"=494.6957746478872, "Y"=417.1636363636364}, {"X"=490.69014084507035, "Y"=420.172027972028}, {"X"=482.6788732394365, "Y"=426.1888111888112}, {"X"=477.67183098591534, "Y"=431.2027972027972}, {"X"=471.66338028169, "Y"=437.21958041958044}, {"X"=468.6591549295773, "Y"=441.2307692307692}, {"X"=467.65774647887315, "Y"=446.24475524475525}, {"X"=467.65774647887315, "Y"=448.2503496503497}, {"X"=471.66338028169, "Y"=453.2643356643357}, {"X"=478.6732394366196, "Y"=457.2755244755245}, {"X"=482.6788732394365, "Y"=460.2839160839161}, {"X"=492.6929577464788, "Y"=464.29510489510494}, {"X"=498.7014084507041, "Y"=465.2979020979021}, {"X"=509.71690140845055, "Y"=467.3034965034965}, {"X"=515.725352112676, "Y"=467.3034965034965}, {"X"=527.7422535211266, "Y"=467.3034965034965}, {"X"=539.7591549295773, "Y"=467.3034965034965}, {"X"=543.7647887323942, "Y"=467.3034965034965}, {"X"=549.7732394366196, "Y"=469.3090909090909}, {"X"=552.7774647887322, "Y"=471.31468531468533}, {"X"=556.7830985915491, "Y"=475.3258741258742}, {"X"=557.7845070422534, "Y"=477.33146853146854}, {"X"=559.7873239436618, "Y"=481.3426573426574}, {"X"=560.7887323943661, "Y"=485.3538461538462}, {"X"=560.7887323943661, "Y"=487.3594405594406}, {"X"=559.7873239436618, "Y"=490.36783216783215}, {"X"=557.7845070422534, "Y"=491.3706293706294}, {"X"=554.7802816901407, "Y"=494.379020979021}, {"X"=552.7774647887322, "Y"=496.38461538461536}, {"X"=547.7704225352111, "Y"=498.39020979020984}, {"X"=544.7661971830985, "Y"=501.3986013986014}, {"X"=543.7647887323942, "Y"=503.4041958041958}, {"X"=542.76338028169, "Y"=508.41818181818184}, {"X"=542.76338028169, "Y"=510.42377622377626}, {"X"=544.7661971830985, "Y"=514.434965034965}, {"X"=545.7676056338026, "Y"=516.4405594405595}, {"X"=546.7690140845069, "Y"=517.4433566433567}, {"X"=546.7690140845069, "Y"=518.4461538461538}, {"X"=547.7704225352111, "Y"=518.4461538461538}, {"X"=547.7704225352111, "Y"=519.448951048951}]  # Engineer Ambitiously 1st Draft
  w2 = cluster{"X":dbl, "Y":dbl}[] array[4488 elements]  # Engineer Ambitiously
  (unwired) cluster{"Horizontal":i32, "Vertical":i32}[] [{"Horizontal"=354, "Vertical"=79}, {"Horizontal"=359, "Vertical"=724}, {"Horizontal"=928, "Vertical"=727}, {"Horizontal"=920, "Vertical"=76}, {"Horizontal"=375, "Vertical"=75}, {"Horizontal"=348, "Vertical"=534}, {"Horizontal"=379, "Vertical"=519}, {"Horizontal"=407, "Vertical"=510}, {"Horizontal"=436, "Vertical"=501}, {"Horizontal"=463, "Vertical"=490}, {"Horizontal"=491, "Vertical"=484}, {"Horizontal"=514, "Vertical"=473}, {"Horizontal"=528, "Vertical"=466}, {"Horizontal"=536, "Vertical"=452}, {"Horizontal"=523, "Vertical"=437}, {"Horizontal"=518, "Vertical"=417}, {"Horizontal"=512, "Vertical"=396}, {"Horizontal"=508, "Vertical"=372}, {"Horizontal"=503, "Vertical"=348}, {"Horizontal"=490, "Vertical"=331}, {"Horizontal"=491, "Vertical"=315}, {"Horizontal"=502, "Vertical"=290}, {"Horizontal"=511, "Vertical"=302}, {"Horizontal"=520, "Vertical"=312}, {"Horizontal"=529, "Vertical"=324}, {"Horizontal"=531, "Vertical"=338}, {"Horizontal"=536, "Vertical"=353}, {"Horizontal"=547, "Vertical"=354}, {"Horizontal"=563, "Vertical"=359}, {"Horizontal"=570, "Vertical"=361}, {"Horizontal"=586, "Vertical"=363}, {"Horizontal"=595, "Vertical"=363}, {"Horizontal"=610, "Vertical"=363}, {"Horizontal"=617, "Vertical"=349}, {"Horizontal"=623, "Vertical"=335}, {"Horizontal"=629, "Vertical"=318}, {"Horizontal"=618, "Vertical"=309}, {"Horizontal"=601, "Vertical"=306}, {"Horizontal"=587, "Vertical"=303}, {"Horizontal"=567, "Vertical"=299}, {"Horizontal"=551, "Vertical"=301}, {"Horizontal"=539, "Vertical"=305}, {"Horizontal"=529, "Vertical"=306}, {"Horizontal"=520, "Vertical"=296}, {"Horizontal"=512, "Vertical"=281}, {"Horizontal"=506, "Vertical"=277}, {"Horizontal"=502, "Vertical"=269}, {"Horizontal"=508, "Vertical"=250}, {"Horizontal"=516, "Vertical"=232}, {"Horizontal"=525, "Vertical"=213}, {"Horizontal"=539, "Vertical"=188}, {"Horizontal"=547, "Vertical"=174}, {"Horizontal"=563, "Vertical"=162}, {"Horizontal"=579, "Vertical"=144}, {"Horizontal"=587, "Vertical"=136}, {"Horizontal"=610, "Vertical"=128}, {"Horizontal"=629, "Vertical"=129}, {"Horizontal"=656, "Vertical"=127}, {"Horizontal"=666, "Vertical"=131}, {"Horizontal"=697, "Vertical"=140}, {"Horizontal"=711, "Vertical"=143}, {"Horizontal"=745, "Vertical"=163}, {"Horizontal"=750, "Vertical"=169}, {"Horizontal"=757, "Vertical"=193}, {"Horizontal"=771, "Vertical"=200}, {"Horizontal"=767, "Vertical"=224}, {"Horizontal"=774, "Vertical"=238}, {"Horizontal"=779, "Vertical"=268}, {"Horizontal"=783, "Vertical"=284}, {"Horizontal"=765, "Vertical"=286}, {"Horizontal"=746, "Vertical"=291}, {"Horizontal"=737, "Vertical"=300}, {"Horizontal"=718, "Vertical"=302}, {"Horizontal"=696, "Vertical"=299}, {"Horizontal"=679, "Vertical"=302}, {"Horizontal"=655, "Vertical"=304}, {"Horizontal"=650, "Vertical"=306}, {"Horizontal"=636, "Vertical"=308}, {"Horizontal"=620, "Vertical"=309}, {"Horizontal"=643, "Vertical"=317}, {"Horizontal"=651, "Vertical"=334}, {"Horizontal"=656, "Vertical"=342}, {"Horizontal"=664, "Vertical"=358}, {"Horizontal"=674, "Vertical"=367}, {"Horizontal"=689, "Vertical"=360}, {"Horizontal"=712, "Vertical"=361}, {"Horizontal"=731, "Vertical"=353}, {"Horizontal"=738, "Vertical"=346}, {"Horizontal"=747, "Vertical"=326}, {"Horizontal"=744, "Vertical"=315}, {"Horizontal"=751, "Vertical"=304}, {"Horizontal"=759, "Vertical"=294}, {"Horizontal"=773, "Vertical"=291}, {"Horizontal"=785, "Vertical"=286}, {"Horizontal"=770, "Vertical"=296}, {"Horizontal"=778, "Vertical"=306}, {"Horizontal"=776, "Vertical"=317}, {"Horizontal"=775, "Vertical"=326}, {"Horizontal"=773, "Vertical"=340}, {"Horizontal"=771, "Vertical"=353}, {"Horizontal"=765, "Vertical"=360}, {"Horizontal"=762, "Vertical"=383}, {"Horizontal"=763, "Vertical"=406}, {"Horizontal"=761, "Vertical"=420}, {"Horizontal"=778, "Vertical"=434}, {"Horizontal"=782, "Vertical"=446}, {"Horizontal"=798, "Vertical"=459}, {"Horizontal"=811, "Vertical"=468}, {"Horizontal"=829, "Vertical"=476}, {"Horizontal"=847, "Vertical"=485}, {"Horizontal"=865, "Vertical"=489}, {"Horizontal"=878, "Vertical"=495}, {"Horizontal"=891, "Vertical"=500}, {"Horizontal"=903, "Vertical"=505}, {"Horizontal"=926, "Vertical"=511}, {"Horizontal"=912, "Vertical"=713}, {"Horizontal"=794, "Vertical"=706}, {"Horizontal"=812, "Vertical"=684}, {"Horizontal"=820, "Vertical"=665}, {"Horizontal"=829, "Vertical"=650}, {"Horizontal"=835, "Vertical"=631}, {"Horizontal"=844, "Vertical"=612}, {"Horizontal"=853, "Vertical"=594}, {"Horizontal"=859, "Vertical"=579}, {"Horizontal"=851, "Vertical"=571}, {"Horizontal"=840, "Vertical"=563}, {"Horizontal"=827, "Vertical"=556}, {"Horizontal"=837, "Vertical"=547}, {"Horizontal"=849, "Vertical"=536}, {"Horizontal"=851, "Vertical"=528}, {"Horizontal"=844, "Vertical"=519}, {"Horizontal"=840, "Vertical"=498}, {"Horizontal"=832, "Vertical"=485}, {"Horizontal"=829, "Vertical"=473}, {"Horizontal"=758, "Vertical"=419}, {"Horizontal"=760, "Vertical"=437}, {"Horizontal"=762, "Vertical"=465}, {"Horizontal"=755, "Vertical"=482}, {"Horizontal"=751, "Vertical"=506}, {"Horizontal"=744, "Vertical"=525}, {"Horizontal"=739, "Vertical"=547}, {"Horizontal"=731, "Vertical"=561}, {"Horizontal"=726, "Vertical"=580}, {"Horizontal"=723, "Vertical"=604}, {"Horizontal"=719, "Vertical"=620}, {"Horizontal"=715, "Vertical"=637}, {"Horizontal"=706, "Vertical"=665}, {"Horizontal"=705, "Vertical"=683}, {"Horizontal"=701, "Vertical"=700}, {"Horizontal"=698, "Vertical"=709}, {"Horizontal"=694, "Vertical"=718}, {"Horizontal"=689, "Vertical"=722}, {"Horizontal"=676, "Vertical"=712}, {"Horizontal"=674, "Vertical"=695}, {"Horizontal"=667, "Vertical"=682}, {"Horizontal"=671, "Vertical"=666}, {"Horizontal"=660, "Vertical"=646}, {"Horizontal"=664, "Vertical"=635}, {"Horizontal"=668, "Vertical"=624}, {"Horizontal"=675, "Vertical"=620}, {"Horizontal"=679, "Vertical"=623}, {"Horizontal"=692, "Vertical"=630}, {"Horizontal"=693, "Vertical"=633}, {"Horizontal"=698, "Vertical"=635}, {"Horizontal"=711, "Vertical"=628}, {"Horizontal"=721, "Vertical"=615}, {"Horizontal"=726, "Vertical"=586}, {"Horizontal"=746, "Vertical"=531}, {"Horizontal"=758, "Vertical"=482}, {"Horizontal"=753, "Vertical"=456}, {"Horizontal"=740, "Vertical"=475}, {"Horizontal"=727, "Vertical"=490}, {"Horizontal"=713, "Vertical"=503}, {"Horizontal"=696, "Vertical"=531}, {"Horizontal"=683, "Vertical"=529}, {"Horizontal"=671, "Vertical"=538}, {"Horizontal"=659, "Vertical"=550}, {"Horizontal"=642, "Vertical"=552}, {"Horizontal"=628, "Vertical"=553}, {"Horizontal"=602, "Vertical"=550}, {"Horizontal"=592, "Vertical"=529}, {"Horizontal"=586, "Vertical"=528}, {"Horizontal"=579, "Vertical"=519}, {"Horizontal"=570, "Vertical"=508}, {"Horizontal"=564, "Vertical"=492}, {"Horizontal"=557, "Vertical"=481}, {"Horizontal"=553, "Vertical"=470}, {"Horizontal"=548, "Vertical"=456}, {"Horizontal"=540, "Vertical"=468}, {"Horizontal"=541, "Vertical"=485}, {"Horizontal"=542, "Vertical"=508}, {"Horizontal"=539, "Vertical"=527}, {"Horizontal"=544, "Vertical"=555}, {"Horizontal"=543, "Vertical"=588}, {"Horizontal"=539, "Vertical"=614}, {"Horizontal"=539, "Vertical"=631}, {"Horizontal"=539, "Vertical"=656}, {"Horizontal"=542, "Vertical"=673}, {"Horizontal"=539, "Vertical"=687}, {"Horizontal"=545, "Vertical"=712}, {"Horizontal"=542, "Vertical"=723}, {"Horizontal"=547, "Vertical"=727}, {"Horizontal"=572, "Vertical"=724}, {"Horizontal"=578, "Vertical"=696}, {"Horizontal"=578, "Vertical"=682}, {"Horizontal"=586, "Vertical"=659}, {"Horizontal"=588, "Vertical"=638}, {"Horizontal"=593, "Vertical"=613}, {"Horizontal"=601, "Vertical"=601}, {"Horizontal"=609, "Vertical"=614}, {"Horizontal"=613, "Vertical"=626}, {"Horizontal"=625, "Vertical"=640}, {"Horizontal"=614, "Vertical"=670}, {"Horizontal"=610, "Vertical"=680}, {"Horizontal"=604, "Vertical"=701}, {"Horizontal"=604, "Vertical"=706}, {"Horizontal"=602, "Vertical"=710}, {"Horizontal"=597, "Vertical"=718}, {"Horizontal"=596, "Vertical"=718}, {"Horizontal"=597, "Vertical"=718}, {"Horizontal"=596, "Vertical"=717}, {"Horizontal"=596, "Vertical"=717}, {"Horizontal"=597, "Vertical"=715}, {"Horizontal"=598, "Vertical"=709}, {"Horizontal"=598, "Vertical"=709}, {"Horizontal"=597, "Vertical"=709}, {"Horizontal"=573, "Vertical"=709}, {"Horizontal"=585, "Vertical"=684}, {"Horizontal"=591, "Vertical"=655}, {"Horizontal"=597, "Vertical"=623}, {"Horizontal"=599, "Vertical"=596}, {"Horizontal"=588, "Vertical"=609}, {"Horizontal"=577, "Vertical"=631}, {"Horizontal"=566, "Vertical"=639}, {"Horizontal"=539, "Vertical"=591}, {"Horizontal"=545, "Vertical"=484}, {"Horizontal"=563, "Vertical"=510}, {"Horizontal"=582, "Vertical"=478}, {"Horizontal"=595, "Vertical"=486}, {"Horizontal"=606, "Vertical"=492}, {"Horizontal"=641, "Vertical"=500}, {"Horizontal"=652, "Vertical"=495}, {"Horizontal"=660, "Vertical"=496}, {"Horizontal"=684, "Vertical"=488}, {"Horizontal"=695, "Vertical"=478}, {"Horizontal"=701, "Vertical"=471}, {"Horizontal"=695, "Vertical"=427}, {"Horizontal"=683, "Vertical"=432}, {"Horizontal"=660, "Vertical"=437}, {"Horizontal"=651, "Vertical"=441}, {"Horizontal"=635, "Vertical"=438}, {"Horizontal"=615, "Vertical"=436}, {"Horizontal"=605, "Vertical"=434}, {"Horizontal"=594, "Vertical"=429}, {"Horizontal"=587, "Vertical"=422}, {"Horizontal"=591, "Vertical"=415}, {"Horizontal"=603, "Vertical"=422}, {"Horizontal"=619, "Vertical"=424}, {"Horizontal"=629, "Vertical"=424}, {"Horizontal"=645, "Vertical"=423}, {"Horizontal"=653, "Vertical"=422}, {"Horizontal"=661, "Vertical"=422}, {"Horizontal"=679, "Vertical"=421}, {"Horizontal"=686, "Vertical"=419}, {"Horizontal"=687, "Vertical"=418}, {"Horizontal"=705, "Vertical"=409}, {"Horizontal"=696, "Vertical"=390}, {"Horizontal"=687, "Vertical"=382}, {"Horizontal"=676, "Vertical"=378}, {"Horizontal"=664, "Vertical"=386}, {"Horizontal"=648, "Vertical"=397}, {"Horizontal"=642, "Vertical"=397}, {"Horizontal"=626, "Vertical"=394}, {"Horizontal"=616, "Vertical"=389}, {"Horizontal"=605, "Vertical"=383}, {"Horizontal"=606, "Vertical"=375}, {"Horizontal"=616, "Vertical"=361}, {"Horizontal"=624, "Vertical"=344}, {"Horizontal"=631, "Vertical"=329}, {"Horizontal"=641, "Vertical"=322}, {"Horizontal"=648, "Vertical"=330}, {"Horizontal"=657, "Vertical"=349}, {"Horizontal"=669, "Vertical"=360}, {"Horizontal"=681, "Vertical"=369}]  # Pixel Points of Jeffs head
  n1 = Array Size(array=w2) -> (size(s)=w3:i32)
  n2 = Subtract(x=w3, y=w9) -> (x-y=w4:i32)
  n3 = Split 1D Array(array=w2, index=w4) -> (first subarray=w1:cluster{"X":dbl, "Y":dbl}[])  [unwired: 1 out]
  n4 = for "Convert pixels into complex values" {
    tunnel: w1 -> [w24] mode=indexing
    tunnel: [w21] -> w17 mode=indexing
    n5 = Unbundle(w24) -> ("X"=w23:dbl, "Y"=w22:dbl)
    n6 = Re/Im To Complex(1:w22, 2:w23) -> (0:w21:cdb)
  }
  n7 = flat-sequence "Remove DC (value pre-calculated)\nCenters Image at 0,0" {
    tunnel: w17 -> [w27]
    tunnel: [w26] -> w10
    frame #0 {
      n8 = Subtract(x=w27, y=cdb 589.8595700606755+385.7411610770612i ("element")) -> (x-y=w26:cdb[])
    }
  }
  n9 = disable-structure shown="Disabled" {
    disable-tunnel: w10 -> [w29 w38]
    disable-tunnel: [w28 w38] -> w13
    frame Enabled {
      n10 = flat-sequence "Smooting Function" {
        tunnel: w29 -> [w36]
        tunnel: [w30] -> w28
        frame #0 {
          w35 = 2.0 ("dt")
          n11 = Array Size(array=w36) -> (size(s)=w34:i32)
          n12 = Build Array (concatenate)(w36, w36) -> (w37:cdb[])
          n13 = Divide(x=w34, y=w35) -> (x/y=w33:dbl)
          n14 = call-poly <vilib>:"Resample (constant to constant).vi"("anti-aliasing?"=FALSE, "dt"=w35, "X"=w37) -> ("Y"=w31:cdb[])  [unwired: 6 in, 2 out]
          n15 = Split 1D Array(array=w31, index=w33) -> (first subarray=w30:cdb[])  [unwired: 1 out]
        }
      }
    }
    frame Disabled {
    }
  }
  n16 = flat-sequence "Do FFT on signal and Scale Output" {
    tunnel: [w41] -> w8
    tunnel: w13 -> [w40]
    frame #0 {
      n17 = call-poly <vilib>:"FFT.vi"("X"=w40) -> ("FFT {X}"=w42:cdb[])  [unwired: 9 in, 1 out]
      n18 = Array Size(array=w42) -> (size(s)=w39:i32)
      n19 = Divide(x=w42, y=w39) -> (x/y=w41:cdb[])
    }
  }
  n20 = flat-sequence "Sort Vectors by Length" {
    tunnel: w8 -> [w45]
    tunnel: [w43] -> w7
    frame #0 {
      n21 = for {
        tunnel: w45 -> [w55] mode=indexing
        tunnel: [w52] -> w46 mode=indexing
        i -> [w53]
        n22 = Complex To Polar(r * e^(i*theta)=w55) -> (r=w54:dbl)  [unwired: 1 out]
        n23 = Bundle(w54, w53) -> (w52:cluster{dbl, i32})  [unwired: 1 in]
      }
      n24 = Sort 1D Array(array=w46) -> (sorted array=w44:cluster{dbl, i32}[])
      n25 = for "shuffle input array by sorted index" {
        tunnel: w45 -> [w51]
        tunnel: w44 -> [w50] mode=indexing
        tunnel: [w47] -> w43 mode=indexing
        n26 = Unbundle(w50) -> (w48:i32)  [unwired: 1 out]
        n27 = Index Array(array=w51, index=w48) -> (element=w49:cdb)
        n28 = Bundle(w49, w48) -> (w47:cluster{cdb, i32})  [unwired: 1 in]
      }
    }
  }
  n29 = Index Array(array=w8) -> (element=→"Centerpoint Offset":cdb)  [unwired: 1 in]
  n30 = Reverse 1D Array(array=w7) -> (reversed array=w6:cluster{cdb, i32}[])
  n31 = for "Create Time Domain Rotating Phasors based off of FFT" {
    N -> [w56]
    tunnel: [w62] -> w18 mode=indexing
    tunnel: w6 -> [w59] mode=indexing
    workers-P: _ -> [_]
    n32 = Unbundle(w59) -> (w58:cdb, w57:i32)
    n33 = Complex To Polar(r * e^(i*theta)=w58) -> (r=w63:dbl, theta=w60:dbl)
    n34 = flat-sequence "Calculate End Phase based on bin#" {
      tunnel: [w68] -> w65
      tunnel: w57 -> [w67]
      tunnel: w60 -> [w66]
      frame #0 {
        n35 = Multiply(x=6.283185307179586, y=w67) -> (x*y=w69:dbl)
        n36 = Add(x=w66, y=w69) -> (x+y=w68:dbl)
      }
    }
    n37 = call-poly <vilib>:"Ramp Pattern.vi"("exclude end?"=TRUE, "start"=w60, "end"=w65, "samples"=w56) -> ("Ramp Pattern"=w64:dbl[])  [unwired: 6 in, 1 out]
    n38 = Polar To Complex(1:w64, 2:w63) -> (0:w62:cdb[])
  }
  n39 = Transpose 2D Array(2D array=w18) -> (transposed array=w19:cdb[][])
  n40 = for "For each time momet/ instance" {
    tunnel: cluster{"Initial":cdb, "Endpoint":cdb} {"Initial"=0.0+0.0i, "Endpoint"=0.0+0.0i} ("Resultant Vector") -> [w76]
    tunnel: w19 -> [w74] mode=indexing
    tunnel: [w75] -> w16 mode=indexing
    tunnel: [w73] -> w15 mode=indexing
    tunnel: [w72] -> w14 mode=indexing
    tunnel: [w71] -> w12 mode=indexing
    workers-P: _ -> [_]
    n41 = for "Create Arrow for each vector" {
      tunnel: [w85] -> w75 mode=indexing
      shift-right: [w78] -> _
      shift-left: w76 -> [w84]
      tunnel: w74 -> [w83] mode=indexing
      tunnel: [w82] -> w73 mode=concatenating
      tunnel: [w82] -> w72
      tunnel: [w77] -> w71
      n42 = Complex To Polar(r * e^(i*theta)=w83) -> (r=w81:dbl, theta=w80:dbl)
      n43 = expression code="(x/pi)*180.0" "radians to degrees"(w80) -> (w79:dbl)
      n44 = call "Vector Arrow.vi"("Magnitude"=w81, "Initial Vector"=w84, "Phase, deg"=w79) -> ("Resultant Vector"=w78:cluster{"Initial":cdb, "Endpoint":cdb}, "XY Graph - Light"=w82:cdb[])  [unwired: 11 in]
      n45 = Unbundle(w78) -> ("Endpoint"=w77:cdb)  [unwired: 1 out]
      n46 = Bundle("XY Graph - Light"=w82) -> (w85:cluster{"XY Graph - Light":cdb[]})  [unwired: 1 in]
    }
  }
  n47 = disable-structure shown="Enabled" {
    frame Disabled {
      n48 = control-ref of="XY Graph"() -> (w86:refnum<vi>)
      n49 = property class="XYGraph (strict)"(reference=w86, "Active Plot"=u32 1) -> (reference out=w89:refnum<vi>, "Plot.Line Width"=w87:u8)  [unwired: 1 in, 1 out]
      n50 = for {
        N: 1000 -> [_]
        tunnel: w89 -> [w97]
        tunnel: [w96] -> _ mode=indexing
        tunnel: w87 -> [w94]
        i -> [w95]
        n51 = Increment(x=w95) -> (x+1=w91:i32)
        n52 = property class="XYGraph (strict)"(reference=w97, "Active Plot"=w91, "Plot.Line Width"=w94, "Plot.Anti-aliased"=TRUE, "Plot.Plot Color"=u32 14467840) -> (error out=w96:errorcluster)  [unwired: 1 in, 1 out]
      }
    }
    frame Enabled {
    }
  }
  n53 = for "Display Data Over Time" {
    tunnel: w16 -> [w110] mode=indexing
    tunnel: w15 -> [w114] mode=indexing
    tunnel: w13 -> [w112]
    tunnel: w14 -> [w109] mode=indexing
    tunnel: w12 -> [w104]
    tunnel: [w98] -> w5
    i -> [w103]
    # "First Plot: Image Drawing Over Time\nSecond Plot: All Vectors for that instant in time\nLast Plot: Original Image\n(optional 3rd plot is the last vector to highlight location)"
    n54 = Increment(x=w103) -> (x+1=w101:i32)
    n55 = Split 1D Array(array=w104, index=w101) -> (first subarray=w102:cdb[])  [unwired: 1 out]
    n56 = Bundle(w102) -> (w100:cluster{cdb[]})  [unwired: 1 in]
    n57 = Bundle("XY Graph - Light"=w114) -> (w113:cluster{"XY Graph - Light":cdb[]})  [unwired: 1 in]
    n58 = Bundle("XY Graph - Light"=w109) -> (w111:cluster{"XY Graph - Light":cdb[]})  [unwired: 1 in]
    n59 = Bundle(w112) -> (w99:cluster{cdb[]})  [unwired: 1 in]
    n60 = Build Array(w100, w113, w111, w99) -> (w107:cluster{"XY Graph - Light":cdb[]}[])
    n61 = Build Array (concatenate)(w100, w110, w99) -> (w108:cluster{"XY Graph - Light":cdb[]}[])
    n62 = Select(t=w108, s="Individual Plots Per Vector", f=w107) -> (s? t:f=→"XY Graph":cluster{"XY Graph - Light":cdb[]}[])
    n63 = Wait (ms)(milliseconds to wait="milliseconds to wait") -> (millisecond timer value=w98:u32)
  }
  n64 = flat-sequence {
    tunnel: w5 -> [_]
    frame #0 {
      n65 = control-ref of="XY Graph"() -> (w116:refnum<vi>)
      n66 = property class="XYGraph (strict)"(reference=w116, "Active Plot"=u32 1, "Plot.Visible?"=FALSE ("Plot.Visible")) -> ()  [unwired: 1 in, 2 out]
    }
  }
  n67 = flat-sequence {
    frame #0 {
      n68 = control-ref of="XY Graph"() -> (w120:refnum<vi>)
      n69 = property class="XYGraph (strict)"(reference=w120, "Value"=cluster{"XY Graph - Light":cdb[]}[] [], "Active Plot"=u32 1, "Plot.Visible?"=TRUE ("Plot.Visible")) -> ()  [unwired: 1 in, 2 out]
    }
  }
